vi "Q14070-Z060B B.vi"() -> ()   [LabVIEW 2013]
uses:
  <vilib>/Utility/file.llb/Read From Spreadsheet File (string).vi
  <vilib>/express/express arith-compare/Formula/XNode/ExpressFormulaBlockNode.xnode
  PCI8622_32.dll
  <vilib>/printing/EasyPrintingControls.llb/contents.ctl
  <vilib>/Utility/NIReport.llb/NI_ReportGenerationCore.lvlib
  <vilib>/printing/EasyPrintingControls.llb/report_type.ctl
  <vilib>/Utility/NIReport.llb/NI_report.lvclass
  <vilib>/printing/EasyPrinting.llb/Easy Print VI Panel or Documentation (path).vi
panel:
  out "监控点压力 2":dbl
  out "监控点压力":dbl
  out "右拉压力数组":dbl[](array[numeric])
  out "右位移数组":dbl[](array[numeric])
  out "左拉压力数组":dbl[](array[numeric])
  out "左位移数组":dbl[](array[numeric])
  out "左轴向力数组大小":i32
  in  "电动缸快速":dbl=15.0
  in  "电动缸慢速":dbl=1.0
  out "最大轴向力标准(N)":dbl=200.0 caption="L+Lmax(mm)" format="%#.3f"
  out "循环退出":bool
  in  "?":bool
  in  "密码":string
  in  "?":bool
  in  "?":bool
  in  "截取百分比":dbl=0.05
  in  "半行程":dbl=70.0
  in  "是否取消放行按钮":bool
  out "PLC":bool
  out "齿条传动比":dbl=200.0 caption="L+Lmax(mm)" format="%#.3f"
  out "右平均轴向力(N)":dbl caption="L+Lmax(mm)" format="%#.3f"
  out "左平均轴向力(N)":dbl caption="最大位移偏离Lmax(mm)" format="%#.3f"
  in  "确定按钮":bool
  out "员工ID":string
  in  "出支线工步号":dbl
  out "报警提示":string
  in  "报警工步号":dbl
  out "急停":bool
  out "DeviceHandle":u32
  in  "轴向力设定次数":dbl=5.0
  in  "最小间隙(mm)":dbl=0.0005 format="%#.3f"
  out "本备料状态H":bool
  out "本测试状态H":bool
  out "本自动状态H":bool
  out "夹头松开":bool
  out "测头右位":bool
  out "测头左位":bool
  in  "测头气缸右移":bool
  in  "测头气缸左移":bool
  in  "轴向力已做次数":dbl
  out "轴向力及全行程间隙合格":bool
  out "轴向力启动":bool
  out "间隙启动":bool
  out "夹头夹紧位":bool
  in  "夹头松开":bool
  in  "夹头夹紧":bool
  out "找帽扭矩":dbl=5.0 caption="压力传感器" format="%#.2f"
  out "error out":errorcluster
  out "型号数量":i32
  out "error out 4":errorcluster
  in  "间隙设定调整次数":dbl=5.0
  out "读取产品ID":string
  out "本备料状态":bool
  out "本测试状态":bool
  out "本自动状态":bool
  out "FGCS":string
  out "KSJJ":string
  out "Z060BRFID":string
  out "轴向力Y":dbl[](array[numeric])
  out "轴向力X":dbl[](array[numeric])
  out "间隙X数组":dbl[](array[numeric])
  out "间隙Y数组":dbl[](array[numeric])
  out "error out 3":errorcluster caption="错误输出"
  out "rfid工步号":u32
  out "芯片ID":string="201209190001"
  out "rfid完成":bool
  out "rfid触发":bool
  out "本序已做":bool
  in  "回零完成":bool
  in  "电动缸回零":bool
  in  "单点间隙已调试次数":dbl
  in  "需调整角度(度)":dbl
  in  "转向器中心":dbl
  out "扭矩到达":bool
  out "黄灯":bool
  out "红灯":bool
  out "基准位移":dbl caption="压力传感器" format="%#.4f"
  out "上序不合格":bool
  out "单点间隙合格":bool
  out "上序合格":bool
  out "测头机构电机":u32
  out "复位":bool
  in  "型号选择":u16(ring)=1 items=["J709", "J728", "J706"]
  in  "联线按钮":bool
  in  "工步号":u32
  in  "产品ID":string="201209190001"
  out "间隙位移(mm)":dbl caption="压力传感器" format="%#.3f"
  out "齿条推拉力(N)":dbl format="%#.2f"
  out "齿条扭矩(Nm)":dbl format="%#.2f"
  out "通讯状态":bool
  out "员工姓名":string
  out "工步提示":string
  out "ADODB._Connection Out 2":refnum<k7>
  out "旋转齿条电机":u32
  out "电动缸电机":u32
  in  "停止":bool
  in  "参数加载":bool
  in  "选项卡控件":T1(tab)
  in  "180°外全行程间隙标准(mm)":dbl=0.1 format="%#.3f"
  out "扭动曲线":cluster{"Y":dbl[], "Y":dbl[]}[](graph) caption="压球涨堵头1"
  out "中间位置间隙":dbl caption="间隙值L(mm)" format="%#.3f"
  in  "中间位置最大间隙标准(mm)":dbl=0.07 format="%#.3f"
  out "右180°外全行程间隙":dbl caption="正向最大间隙L1(mm)" format="%#.3f"
  out "左180°外全行程间隙":dbl caption="正向最大间隙L1(mm)" format="%#.3f"
  out "右180°内全行程间隙":dbl caption="正向最大间隙L1(mm)" format="%#.3f"
  out "左180°内全行程间隙":dbl caption="正向最大间隙L1(mm)" format="%#.3f"
  in  "180°内全行程间隙标准(mm)":dbl=0.07 format="%#.3f"
  in  "找帽OK":bool
  out "左全行程间隙":dbl caption="正向最大间隙L1(mm)" format="%#.3f"
  out "右全行程间隙":dbl caption="正向最大间隙L1(mm)" format="%#.3f"
  out "总圈数最大值":dbl
  out "总圈数标准":dbl
  out "总行程最大值":dbl
  out "总行程标准(mm)":dbl
  out "力波动标准(N)":dbl=60.0 caption="L+Lmax(mm)" format="%#.3f"
  out "轴向力标准(N)":dbl=100.0 caption="L+Lmax(mm)" format="%#.3f"
  out "右轴向力波动(N)":dbl caption="L+Lmax(mm)" format="%_4g"
  out "右最大轴向力(N)":dbl caption="L+Lmax(mm)" format="%_4g"
  out "左轴向力波动(N)":dbl caption="最大位移偏离Lmax(mm)" format="%_4g"
  out "左最大轴向力(N)":dbl caption="最大位移偏离Lmax(mm)" format="%_4g"
  out "行程跳动曲线":cluster{"Y":dbl[], "Y":dbl[]}[](graph) caption="压球涨堵头1"
  out "平均轴向力标准(N) max":dbl=200.0 caption="L+Lmax(mm)" format="%#.3f"
  out "总行程":dbl format="%_4g"
  out "总圈数":dbl format="%_4g"
  in  "不合格品":bool
  in  "扭矩停止值":dbl=16.0
  in  "齿条右极限":dbl=-70.0 caption="压力传感器" format="%#.2f"
  in  "齿条左极限":dbl=-262.0 caption="压力传感器" format="%#.2f"
  in  "齿条移动速度":dbl=5.0 caption="压力传感器" format="%#.2f"
  in  "旋转齿条轴找帽转速":dbl=5.0 caption="压力传感器" format="%#.2f"
  in  "测量点扭矩":dbl=4.0 caption="压力传感器" format="%#.2f"
  in  "旋转齿条轴测量转速":dbl caption="压力传感器" format="%#.2f"
  in  "测头机构轴后退位":dbl=30.0 caption="压力传感器" format="%#.2f"
  in  "测头机构轴待检位":dbl caption="压力传感器" format="%#.2f"
  in  "测头机构轴检测位":dbl caption="压力传感器" format="%#.2f"
  in  "测头机构轴移动速度":dbl caption="压力传感器" format="%#.2f"
  in  "机械间隙值":dbl=3.5
  in  "阻挡":bool
  in  "放行":bool
  in  "夹头松开":bool
  in  "夹头夹紧":bool
  in  "测头气缸右移":bool
  in  "测头气缸左移":bool
  in  "支线下降":bool
  in  "支线顶升":bool
  in  "出支线":bool
  in  "进支线":bool
  in  "主线下降":bool
  in  "主线顶升":bool
  in  "下阻挡器放行":bool
  in  "上阻挡器放行":bool
  in  "测头机构轴使能":bool
  in  "测头机构轴后退":bool
  in  "测头机构轴前进":bool
  in  "电动缸速度(mm/s)":dbl=10.0 format="%#.3f"
  out "电动缸位置(mm)":dbl=10000.0 format="%#.3f"
  in  "旋转齿条轴速度(°/s)":dbl=10.0 format="%#.3f"
  out "旋转齿条轴位置(°)":dbl=10000.0 format="%#.3f"
  in  "测头机构轴速度(mm/s)":dbl=10.0 format="%#.3f"
  out "测头机构轴位置(mm)":dbl=10000.0 format="%#.3f"
  in  "旋转齿条轴右转":bool
  in  "旋转齿条轴左转":bool
  in  "旋转齿条轴使能":bool
  in  "电动缸后退":bool
  in  "电动缸使能":bool
  in  "电动缸前进":bool
  in  "齿条扭矩比例偏移":dbl=1.0 format="%#.2f"
  in  "齿条扭矩零点偏移":dbl format="%#.2f"
  in  "齿条推拉力比例偏移":dbl=1.0 format="%#.2f"
  in  "齿条推拉力零点偏移":dbl format="%#.2f"
  in  "间隙位移比例偏移":dbl=1.0 format="%#.2f"
  in  "间隙位移零点偏移":dbl format="%#.2f"
  in  "传感器参数保存":bool
  in  "参数修改":bool
  in  "参数查询":bool
  in  "参数浏览表":string[][](table)
  # "芜湖机械转向器装配线"
  # "间隙及轴向力检测"
  # "湖北唯思凌科装备制造有限公司 设计开发 (C)2015"
  # "Q14070机械转向器装配线"
  # "≤"
  # "间隙测量结果"
  # "间隙测量判定值"
  # "≤"
  # "≤"
  # "≤"
  # "轴向力测量结果"
  # "轴向力测量标准"
  # "≥"
  # "≤"
  # "≥"
  # "≤"
  # "≤"
  # "≥"
  # "不得大于20NM"
  # "传感器校验区"
  # "关于传感器校验：\n1、传感器校验需要由具备资质的单位或部门进行校验。\n2、具备权限的用户才能够修改传感器校验参数和试验参数。\n3、修改校验参数方法：先将比例偏移置为1，修改零点偏移，使零点值与校验的传感器一致；然后根据增幅调整比例偏移。"
  # "注意：\n具备权限的用户才能够修改传感器校验参数和试验参数！"
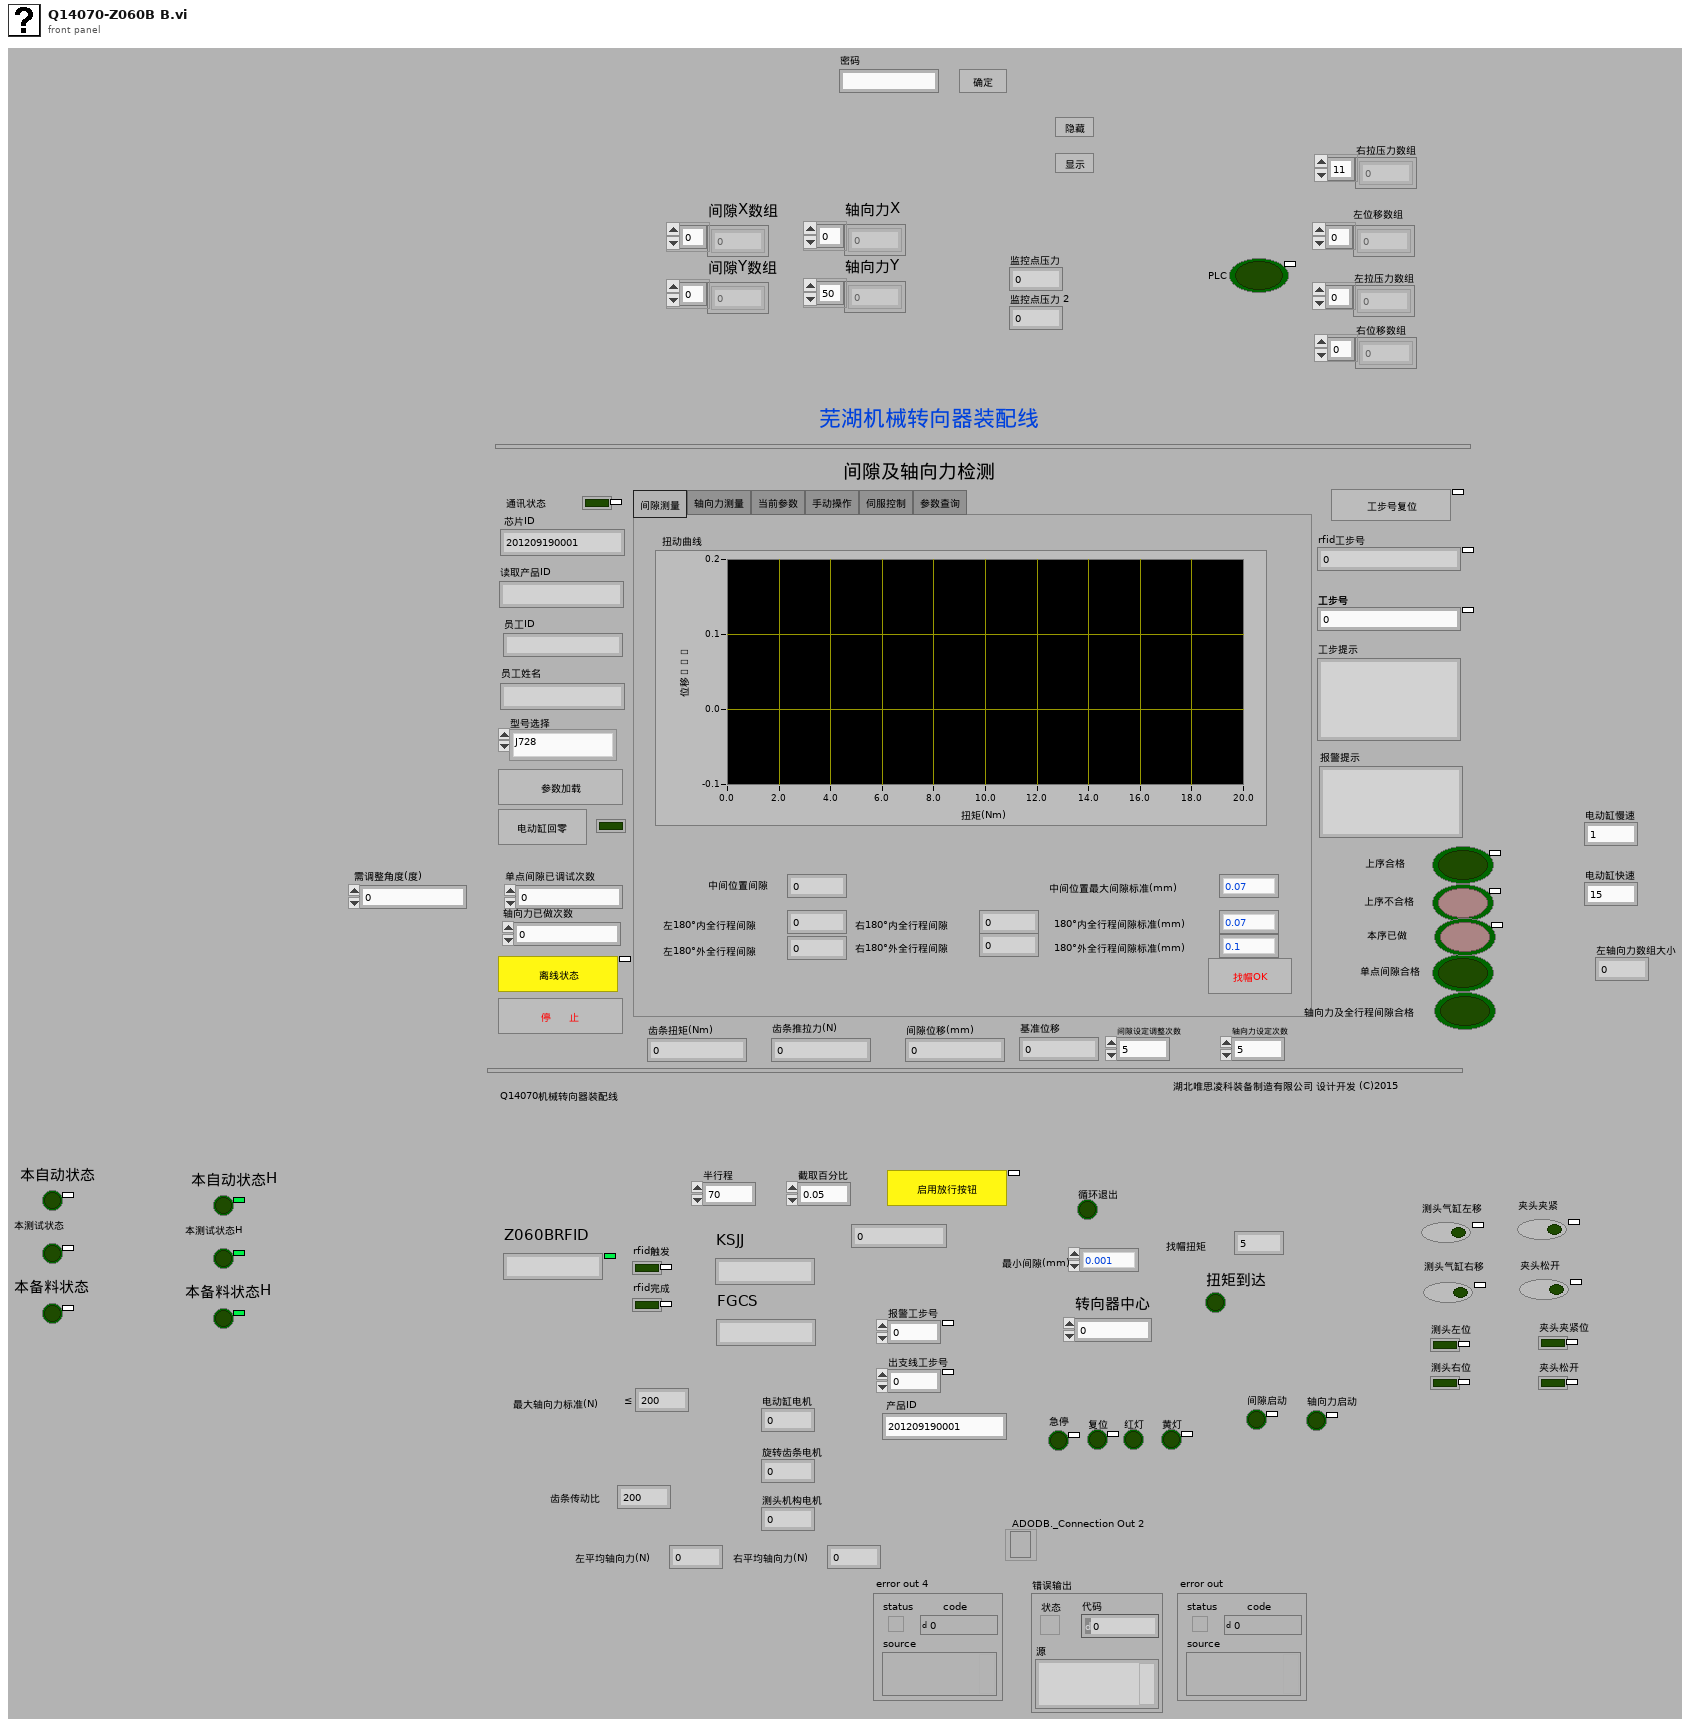
[diagram p1: front panel]
types:
  T1 = enum32{"间隙测量", "轴向力测量", "当前参数", "手动操作", "伺服控制", "传感器校验", "参数查询"}
  T2 = enum8{"Enabled", "Disabled", "Disabled and Grayed Out"}
  T3 = typedef "NI_ReportGenerationCore.lvlib/report_type.ctl" = u16
  T4 = typedef "NI_ReportGenerationCore.lvlib/contents.ctl" = u16
  T5 = typedef "imagedata.ctl" = cluster{"image type":i32, "image depth":i32, "image":u8[], "mask":u8[], "colors":u32[], "Rectangle":cluster{"left":i16, "top":i16, "right":i16, "bottom":i16}}
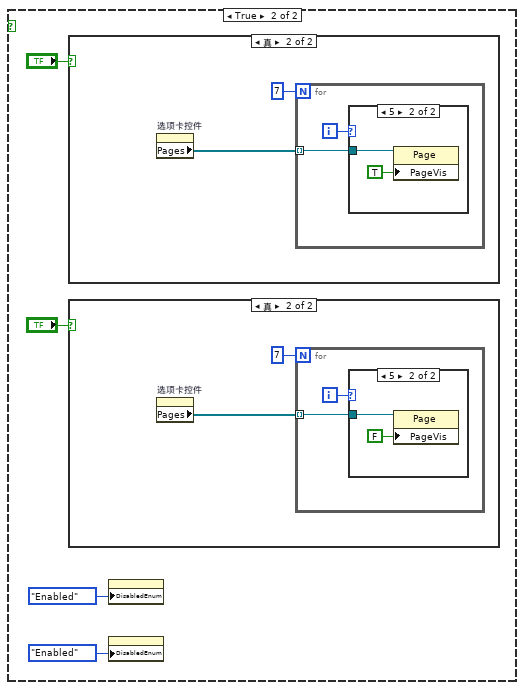
[diagram p2: hidden frame]
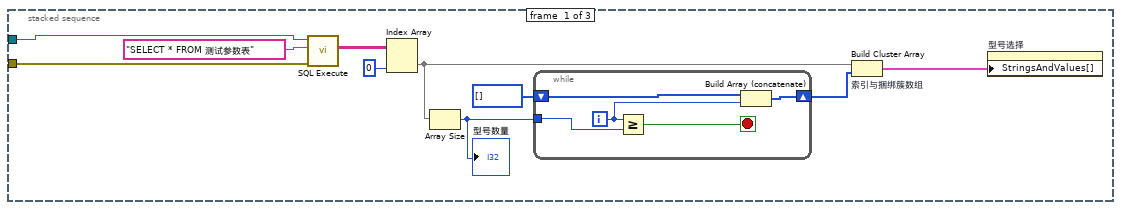
[diagram p9: hidden frame]
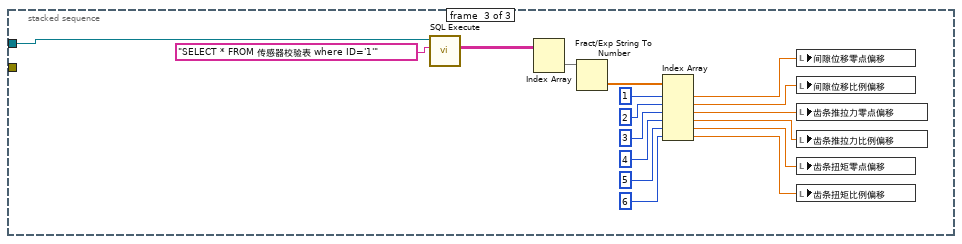
[diagram p10: hidden frame]
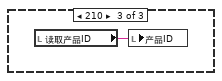
[diagram p12: hidden frame]
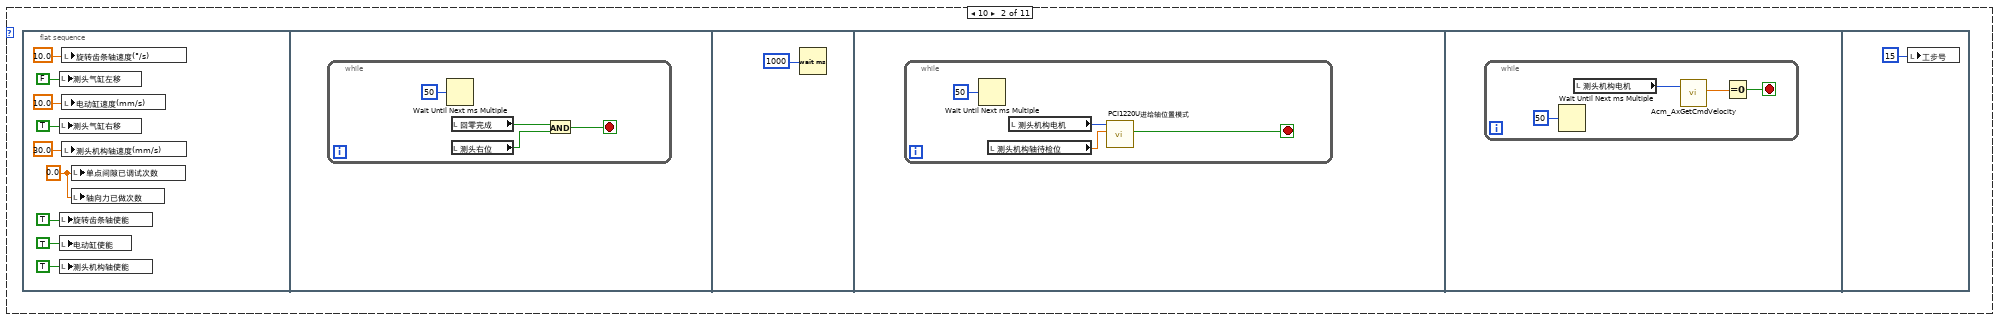
[diagram p14: hidden frame]
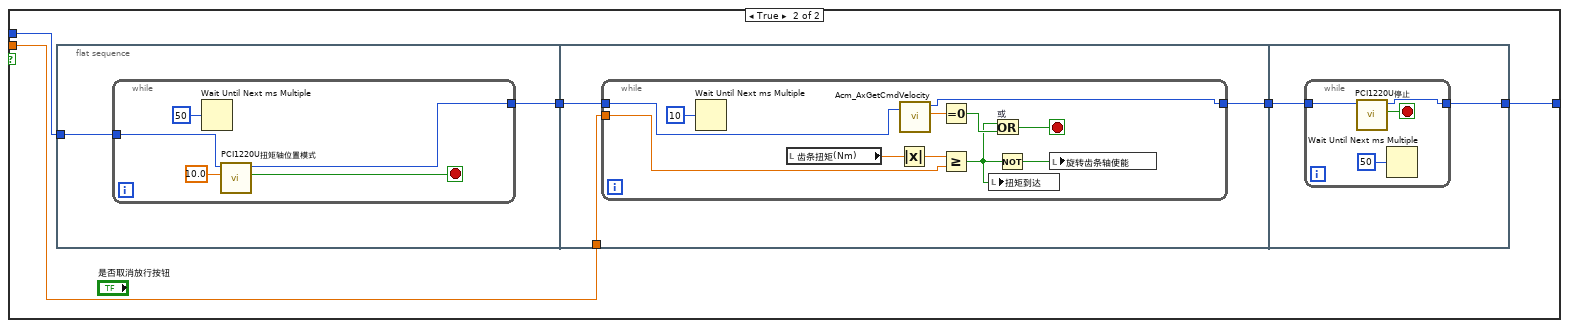
[diagram p15: hidden frame]
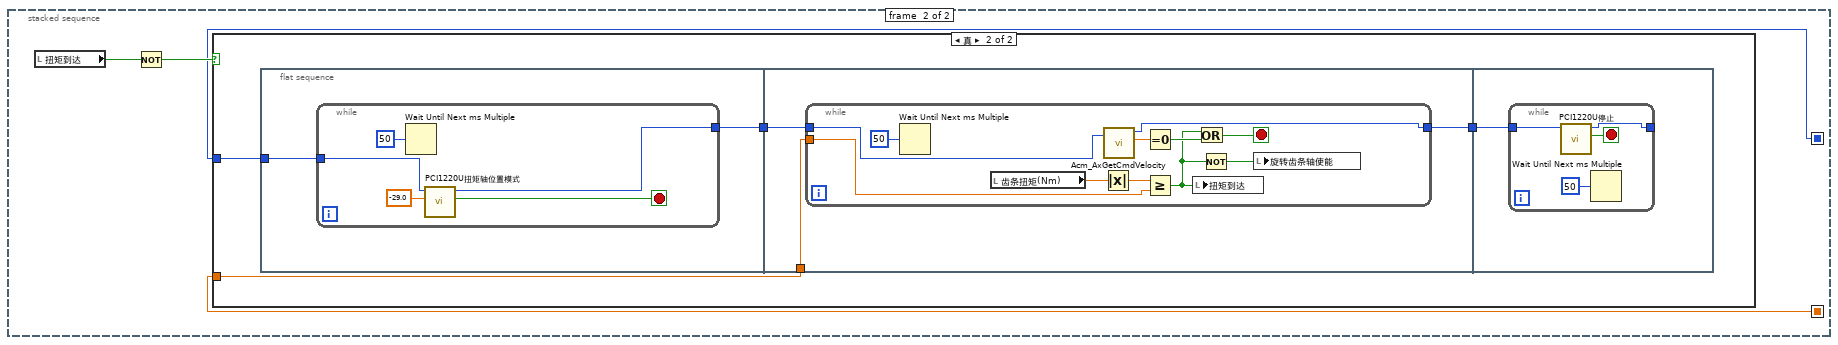
[diagram p16: hidden frame]
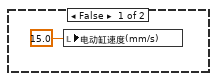
[diagram p17: hidden frame]
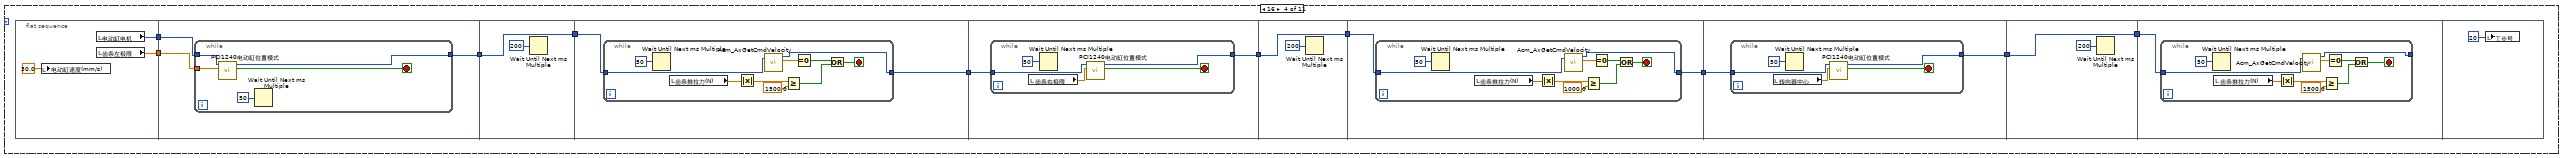
[diagram p19: hidden frame]
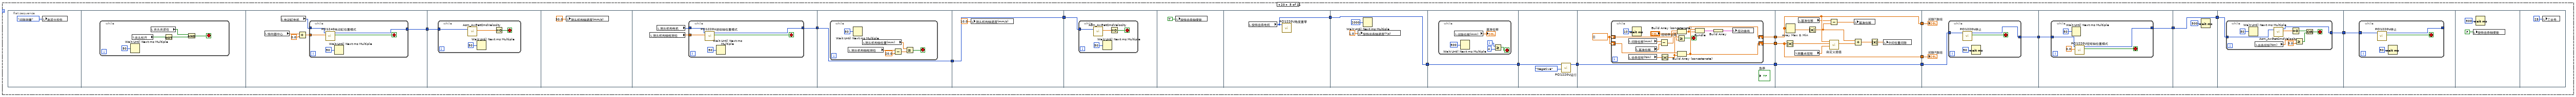
[diagram p20: hidden frame]
diagram:
  n1 = while {
    stop <- FALSE stop-if-true
    n2 = Equal?(x="密码", y="jizhuan") -> (x = y?=w8:bool)
    n3 = Compound Arithmetic op=AND(w8, "?") -> (w6:bool)
    n4 = case shown="假" w6 {
      frame False {
        n5 = property class="Bool (严格)"("DisabledEnum"=T2."Disabled and Grayed Out" ("禁用")) -> ()  [unwired: 2 in, 2 out]
        n6 = property class="Bool (严格)"("DisabledEnum"=T2."Disabled and Grayed Out" ("禁用")) -> ()  [unwired: 2 in, 2 out]
      }
      frame True {
        n7 = case shown="真" "?" {
          frame False {
          }
          frame True {
            n8 = property on="选项卡控件" class="TabCtl (严格)"() -> ("Pages"=w23:refnum<vi>[])  [unwired: 2 in, 2 out]
            n9 = for {
              N: 7 -> [_]
              tunnel: w23 -> [w25] mode=indexing
              i -> [w26]
              n10 = case shown="5" w26 {
                tunnel: w25 -> [_ w28]
                frame 0, Default {
                }
                frame 5 {
                  n11 = property class="Page"(reference=w28, "PageVis"=TRUE ("选项卡可见")) -> ()  [unwired: 1 in, 2 out]
                }
              }
            }
          }
        }
        n12 = case shown="真" "?" {
          frame False {
          }
          frame True {
            n13 = property on="选项卡控件" class="TabCtl (严格)"() -> ("Pages"=w17:refnum<vi>[])  [unwired: 2 in, 2 out]
            n14 = for {
              N: 7 -> [_]
              tunnel: w17 -> [w19] mode=indexing
              i -> [w20]
              n15 = case shown="5" w20 {
                tunnel: w19 -> [_ w22]
                frame 0, Default {
                }
                frame 5 {
                  n16 = property class="Page"(reference=w22, "PageVis"=FALSE ("选项卡可见")) -> ()  [unwired: 1 in, 2 out]
                }
              }
            }
          }
        }
        n17 = property class="Bool (严格)"("DisabledEnum"=T2."Enabled" ("禁用")) -> ()  [unwired: 2 in, 2 out]
        n18 = property class="Bool (严格)"("DisabledEnum"=T2."Enabled" ("禁用")) -> ()  [unwired: 2 in, 2 out]
      }
    }
  }
  n19 = flat-sequence {
    tunnel: [w32] -> w2
    tunnel: [w30] -> w1
    tunnel: w2 -> [w42]
    tunnel: w1 -> [w41]
    frame #0 {
      n20 = First Call?() -> (First Call?: T/F=w29:bool)
      n21 = case shown="真" w29 {
        frame False {
        }
        frame True {
          n22 = while {
            i -> [w37]
            stop <- w35 stop-if-true
            w40 = TRUE ("电动缸使能")
            n23 = local write "回零完成"(FALSE ("回零完成")) -> ()
            n24 = Wait Until Next ms Multiple(millisecond multiple=u32 50 ("毫秒倍数")) -> ()  [unwired: 1 out]
            n25 = local write "电动缸使能"(w40) -> ()
            n26 = local write "测头机构轴使能"(w40) -> ()
            n27 = local write "旋转齿条轴使能"(w40) -> ()
            n28 = Greater Or Equal?(x=w37, y=30) -> (x >= y?=w35:bool)
          }
        }
      }
      n29 = call "ADO Connection Create.vi"() -> ("error out"=w33:errorcluster, "ADODB._Connection Out"=w34:refnum<k7>)  [unwired: 10 in]
      n30 = call "ADO Connection Open.vi"("error in (no error)"=w33, "ConnectionString"="Provider=Microsoft.Jet.OLEDB.4.0;Data Source=D:\\Q14070-Z060人机界面\\参数\\参数Z060.mdb;Persist Security Info=False;Jet OLEDB:Database Password=1234;", "ADODB._Connection In"=w34) -> ("error out"=w30:errorcluster, "ADODB._Connection Out"=w32:refnum<k7>)  [unwired: 7 in]
    }
    frame #1 {
      n31 = while {
        tunnel: w42 -> [w44]
        tunnel: w41 -> [w43]
        stop <- w48 stop-if-true
        n32 = Wait (ms)(milliseconds to wait=u32 50 ("等待时间（毫秒）")) -> ()  [unwired: 1 out]
        n33 = First Call?() -> (First Call?: T/F=w47:bool)
        n34 = Or(x=w47, y="参数加载") -> (x .or. y?=w46:bool)
        n35 = case shown="真" w46 {
          tunnel: w44 -> [_ w51]
          tunnel: w43 -> [_ w50]
          frame False {
          }
          frame True {
            n36 = stacked-sequence {
              tunnel: w51 -> [w57 w68 w126]
              tunnel: w50 -> [w52 _ _]
              frame #0 {
                n37 = call "SQL Execute.vi"("error in (no error)"=w52, "Command Text"="SELECT * FROM 测试参数表", "ADODB._Connection In"=w57) -> ("Data"=w55:string[][])  [unwired: 5 in, 3 out]
                n38 = Index Array(array=w55, index (col)=0 ("索引 (行)")) -> (element=w59:string[])  [unwired: 1 in]
                n39 = Array Size(array=w59) -> (size(s)=w54:i32)
                "型号数量" <- w54
                n40 = while {
                  shift-right: [w66] -> w58
                  shift-left: i32[] [] -> [w65]
                  tunnel: w54 -> [w63]
                  i -> [w64]
                  stop <- w62 stop-if-true
                  n41 = Greater Or Equal?(x=w64, y=w63) -> (x >= y?=w62:bool)
                  n42 = Build Array (concatenate)(w65, w64) -> (w66:i32[])
                }
                n43 = Build Cluster Array "索引与捆绑簇数组"(w59, w58) -> (w53:cluster{"String":string, i32}[])
                n44 = property on="型号选择" class="Ring (严格)"("StringsAndValues[]"=w53) -> ()  [unwired: 2 in, 2 out]
              }
              frame #1 {
                n45 = property on="型号选择" class="Ring (严格)"() -> ("RingText.Text"=w69:string)  [unwired: 2 in, 2 out]
                n46 = call "创建文本2"("型号选择"=w69) -> ("Result"=w73:string)  [unwired: 13 in, 1 out]
                n47 = call "SQL Execute.vi"("Command Text"=w73, "ADODB._Connection In"=w68) -> ("Data"=w72:string[][])  [unwired: 6 in, 3 out]
                n48 = Index Array(array=w72, index (row)=0 ("索引 (行)")) -> (element=w70:string[])  [unwired: 1 in]
                n49 = Fract/Exp String To Number ("分数/指数字符串至数值转换")(string=w70) -> (number=w67:dbl[])  [unwired: 3 in, 1 out]
                n50 = stacked-sequence {
                  tunnel: w67 -> [w102]
                  frame #0 {
                    n51 = Index Array ("索引数组")(array=w102, index #1=2 ("索引"), index #2=3 ("索引"), index #3=4 ("索引"), index #4=5 ("索引"), index #5=6 ("索引"), index #6=7 ("索引"), index #7=8 ("索引"), index #8=9 ("索引"), index #9=10 ("索引"), index #10=11 ("索引"), index #11=12 ("索引"), index #12=13 ("索引"), index #13=14 ("索引"), index #14=15 ("索引"), index #15=16 ("索引"), index #16=17 ("索引"), index #17=18 ("索引"), index #18=19 ("索引"), index #19=20 ("索引")) -> (element #1=w101:dbl, element #2=w100:dbl, element #3=w99:dbl, element #4=w98:dbl, element #5=w97:dbl, element #6=w96:dbl, element #7=w95:dbl, element #8=w94:dbl, element #9=w93:dbl, element #10=w92:dbl, element #11=w85:dbl, element #12=w84:dbl, element #13=→"齿条传动比":dbl, element #14=→"力波动标准(N)":dbl, element #15=→"轴向力标准(N)":dbl, element #16=→"平均轴向力标准(N) max":dbl, element #17=→"总圈数标准":dbl, element #18=→"总圈数最大值":dbl, element #19=w80:dbl)
                    n52 = local write "测头机构轴移动速度"(w101) -> ()
                    n53 = local write "测头机构轴检测位"(w100) -> ()
                    n54 = local write "测头机构轴待检位"(w99) -> ()
                    n55 = local write "测头机构轴后退位"(w98) -> ()
                    n56 = local write "齿条移动速度"(w97) -> ()
                    n57 = local write "齿条左极限"(w96) -> ()
                    n58 = local write "齿条右极限"(w95) -> ()
                    n59 = local write "旋转齿条轴找帽转速"(w94) -> ()
                    n60 = local write "旋转齿条轴测量转速"(w93) -> ()
                    n61 = local write "测量点扭矩"(w92) -> ()
                    n62 = local write "总行程标准(mm)"(w85) -> ()
                    n63 = local write "总行程最大值"(w84) -> ()
                    n64 = local write "转向器中心"(w80) -> ()
                  }
                }
              }
              frame #2 {
                n65 = call "SQL Execute.vi"("Command Text"="SELECT * FROM 传感器校验表 where ID='1'", "ADODB._Connection In"=w126) -> ("Data"=w128:string[][])  [unwired: 6 in, 3 out]
                n66 = Index Array(array=w128) -> (element=w129:string[])  [unwired: 2 in]
                n67 = Fract/Exp String To Number ("分数/指数字符串至数值转换")(string=w129) -> (number=w119:dbl[])  [unwired: 3 in, 1 out]
                n68 = Index Array(array=w119, index #1=1 ("索引"), index #2=2 ("索引"), index #3=3 ("索引"), index #4=4 ("索引"), index #5=5 ("索引"), index #6=6 ("索引")) -> (element #1=w118:dbl, element #2=w117:dbl, element #3=w116:dbl, element #4=w115:dbl, element #5=w114:dbl, element #6=w113:dbl)
                n69 = local write "间隙位移零点偏移"(w118) -> ()
                n70 = local write "间隙位移比例偏移"(w117) -> ()
                n71 = local write "齿条推拉力零点偏移"(w116) -> ()
                n72 = local write "齿条推拉力比例偏移"(w115) -> ()
                n73 = local write "齿条扭矩零点偏移"(w114) -> ()
                n74 = local write "齿条扭矩比例偏移"(w113) -> ()
              }
            }
          }
        }
        n75 = local read "停止"() -> (w48:bool)
        "ADODB._Connection Out 2" <- w44
      }
    }
  }
  n76 = while {
    stop <- w131 stop-if-true
    n77 = stacked-sequence {
      frame #0 {
        n78 = flat-sequence {
          frame #0 {
          }
          frame #1 {
            "PLC" <- "阻挡"
          }
          frame #2 {
            n79 = First Call?() -> (First Call?: T/F=w133:bool)
            n80 = case shown="真" w133 {
              frame False {
              }
              frame True {
                n81 = call "员工管理测试程序.vi"() -> ("员工姓名"=w135:string, "员工ID"=w134:string)  [unwired: 10 in]
                n82 = local write "员工ID"(w134) -> ()
                n83 = local write "员工姓名"(w135) -> ()
              }
            }
          }
          frame #3 {
          }
          frame #4 {
          }
          frame #5 {
          }
          frame #6 {
          }
        }
      }
      frame #1 {
        n84 = flat-sequence {
          frame #0 {
            n85 = property on="型号选择" class="Ring (严格)"() -> ("RingText.Text"=w139:string)  [unwired: 2 in, 2 out]
            n86 = case shown="\"J728\"" w139 {
              frame "J709", Default {
                w140 = FALSE ("可见")
                w141 = TRUE ("可见")
                n87 = property on="左全行程间隙" class="DigNum (严格)"("Visible"=w141) -> ()  [unwired: 2 in, 2 out]
                n88 = property on="右全行程间隙" class="DigNum (严格)"("Visible"=w141) -> ()  [unwired: 2 in, 2 out]
                n89 = property on="左180°内全行程间隙" class="DigNum (严格)"("Visible"=w140) -> ()  [unwired: 2 in, 2 out]
                n90 = property on="左180°外全行程间隙" class="DigNum (严格)"("Visible"=w140) -> ()  [unwired: 2 in, 2 out]
                n91 = property on="右180°内全行程间隙" class="DigNum (严格)"("Visible"=w140) -> ()  [unwired: 2 in, 2 out]
                n92 = property on="右180°外全行程间隙" class="DigNum (严格)"("Visible"=w140) -> ()  [unwired: 2 in, 2 out]
              }
              frame "J706" {
                w142 = TRUE ("可见")
                w143 = FALSE ("可见")
                n93 = property on="左全行程间隙" class="DigNum (严格)"("Visible"=w143) -> ()  [unwired: 2 in, 2 out]
                n94 = property on="右全行程间隙" class="DigNum (严格)"("Visible"=w143) -> ()  [unwired: 2 in, 2 out]
                n95 = property on="左180°内全行程间隙" class="DigNum (严格)"("Visible"=w142) -> ()  [unwired: 2 in, 2 out]
                n96 = property on="左180°外全行程间隙" class="DigNum (严格)"("Visible"=w142) -> ()  [unwired: 2 in, 2 out]
                n97 = property on="右180°内全行程间隙" class="DigNum (严格)"("Visible"=w142) -> ()  [unwired: 2 in, 2 out]
                n98 = property on="右180°外全行程间隙" class="DigNum (严格)"("Visible"=w142) -> ()  [unwired: 2 in, 2 out]
              }
              frame "J728" {
                w144 = TRUE ("可见")
                w145 = FALSE ("可见")
                n99 = property on="左全行程间隙" class="DigNum (严格)"("Visible"=w145) -> ()  [unwired: 2 in, 2 out]
                n100 = property on="右全行程间隙" class="DigNum (严格)"("Visible"=w145) -> ()  [unwired: 2 in, 2 out]
                n101 = property on="左180°内全行程间隙" class="DigNum (严格)"("Visible"=w144) -> ()  [unwired: 2 in, 2 out]
                n102 = property on="左180°外全行程间隙" class="DigNum (严格)"("Visible"=w144) -> ()  [unwired: 2 in, 2 out]
                n103 = property on="右180°内全行程间隙" class="DigNum (严格)"("Visible"=w144) -> ()  [unwired: 2 in, 2 out]
                n104 = property on="右180°外全行程间隙" class="DigNum (严格)"("Visible"=w144) -> ()  [unwired: 2 in, 2 out]
              }
            }
          }
          frame #1 {
            (unwired) string[] ["I急停按钮", "I自动旋钮", "I启动按钮", "I备用按钮", "I复位按钮", "I上阻挡器放行", "I下阻挡器放行", "I进支线按钮"] ("I0说明")
            (unwired) string[] ["I出支线按钮", "I主线顶升按钮", "I主线下降按钮", "I支线顶升按钮", "I支线下降按钮", "I气压报警", "未使用", "未使用"] ("I0说明")
            n105 = local read "间隙位移(mm)"() -> (w148:dbl)
            n106 = Greater Or Equal?(x=w148, y=4.0) -> (x >= y?=w146:bool)
            n107 = case shown="真" w146 {
              frame False {
              }
              frame True {
                n108 = local write "测头机构轴使能"(FALSE ("测头机构轴使能")) -> ()
              }
            }
          }
          frame #2 {
            (unwired) string[] ["I电动缸SRDY", "I电动缸ZSPD", "I电动缸ALRM", "I间隙进给SRDY", "I间隙进给ZSPD", "I间隙进给ALRM", "I间隙旋转SRPD", "I间隙旋转ZSPD"] ("I0说明")
            n109 = local read "测头机构轴位置(mm)"() -> (w152:dbl)
            n110 = Greater Or Equal?(x=w152, y=90.0) -> (x >= y?=w150:bool)
            n111 = case shown="假" w150 {
              frame False {
                w153 = T2."Enabled" ("禁用")
                n112 = property on="测头气缸左移" class="Bool (严格)"("DisabledEnum"=w153) -> ()  [unwired: 2 in, 2 out]
                n113 = property on="测头气缸右移" class="Bool (严格)"("DisabledEnum"=w153) -> ()  [unwired: 2 in, 2 out]
                n114 = property on="测头气缸左移" class="Bool"("DisabledEnum"=w153) -> ()  [unwired: 2 in, 2 out]
                n115 = property on="测头气缸右移" class="Bool"("DisabledEnum"=w153) -> ()  [unwired: 2 in, 2 out]
              }
              frame True {
                w154 = T2."Disabled" ("禁用")
                w155 = FALSE ("测头气缸右移")
                n116 = local write "测头气缸右移"(w155) -> ()
                n117 = local write "测头气缸左移"(w155) -> ()
                n118 = property on="测头气缸左移" class="Bool (严格)"("DisabledEnum"=w154) -> ()  [unwired: 2 in, 2 out]
                n119 = property on="测头气缸右移" class="Bool (严格)"("DisabledEnum"=w154) -> ()  [unwired: 2 in, 2 out]
                n120 = property on="测头气缸左移" class="Bool"("DisabledEnum"=w154) -> ()  [unwired: 2 in, 2 out]
                n121 = property on="测头气缸右移" class="Bool"("DisabledEnum"=w154) -> ()  [unwired: 2 in, 2 out]
              }
            }
          }
          frame #3 {
            (unwired) string[] ["I间隙旋转ALRM", "I扭矩旋转SRPD", "I扭矩旋转ZSPD", "I扭矩旋转ALRM", "I拧紧机合格", "I拧紧机不合格", "I拧紧机报警", "未使用"] ("I0说明")
          }
        }
        n122 = local read "急停"() -> (w138:bool)
        n123 = local read "复位"() -> (w137:bool)
        n124 = Compound Arithmetic op=OR(invert w138, w137) -> (→"循环退出":bool)
      }
      frame #2 {
        n125 = flat-sequence {
          frame #0 {
            (unwired) string[] ["I自制气缸进位", "I自制气缸原位", "I上工位检测", "I本工位检测", "I下工位检测", "I主线顶升上位", "I主线顶升下位", "I支线顶升上位"] ("I0说明")
          }
          frame #1 {
            (unwired) string[] ["I支线顶升下位", "I支线进到位", "I支线退到位", "I位移气缸原位", "I位移气缸进位", "I拧紧机在位", "I电动缸原位", "I电动缸进位"] ("I0说明")
          }
          frame #2 {
            (unwired) string[] ["未使用", "未使用", "未使用", "未使用", "未使用", "未使用", "未使用", "未使用"] ("I0说明")
          }
          frame #3 {
            (unwired) string[] ["未使用", "未使用", "未使用", "未使用", "未使用", "未使用", "未使用", "未使用"] ("I0说明")
          }
        }
        n126 = local read "本备料状态"() -> (w156:bool)
        n127 = local read "本自动状态"() -> (w158:bool)
        n128 = local read "本测试状态"() -> (w157:bool)
        n129 = local write "本备料状态H"(w156) -> ()
        n130 = local write "本自动状态H"(w158) -> ()
        n131 = local write "本测试状态H"(w157) -> ()
      }
      frame #3 {
        n132 = local read "报警工步号"() -> (w160:dbl)
        n133 = local read "工步号"() -> (w162:u32)
        n134 = case shown="3" w160 {
          tunnel: [_ "操作步骤错请取胶瓶" "操作步骤错误请点标" "测头气缸不在原位" "急停被按下" "气压报警" "电动缸伺服报警" "旋转伺服服报警" "测头伺服服报警"] -> w159
          frame 0, Default {
          }
          frame 1 {
          }
          frame 3 {
          }
          frame 2 {
          }
          frame 4 {
          }
          frame 5 {
          }
          frame 6 {
          }
          frame 7 {
          }
          frame 8 {
          }
        }
        "报警提示" <- w159
        n135 = case shown="0, 默认" w162 {
          tunnel: [w172 "请取胶瓶" ("工步描述") "请对锁紧螺母加力" ("工步描述") "灵敏度测试中" ("工步描述") "有油刚度测试中" ("工步描述") "安装好锁紧螺母后，按顶升按钮，夹具夹紧" ("工步描述") "请点击启动按钮进行试验" ("工步描述") "探头气缸右移" ("工步描述") "电动缸前进找中" ("工步描述") "探头前进测试开始" ("工步描述") "探头退回" ("工步描述") "轴向力测试中" ("工步描述") "测头后退夹抓松开" ("工步描述") "伺服回零" ("工步描述") "力特性试验完成" ("工步描述") "套好输出轴把手，按启动按钮，做回正力试验" ("工步描述") "回正力试验中" ("工步描述") "试验完成，将把手拉回，取下油管，按顶升按钮" ("工步描述") "拆下锁紧螺母和输入轴万向节，按顶升按钮" ("工步描述")] -> w161
          frame 0, Default {
            n136 = local read "联线按钮"() -> (w171:bool)
            n137 = case shown="真" w171 {
              tunnel: ["等待工件" ("工步描述") "等待扫描条码" ("工步描述")] -> w172
              frame False {
              }
              frame True {
              }
            }
          }
          frame 1 {
          }
          frame 2 {
          }
          frame 3 {
          }
          frame 4 {
          }
          frame 5 {
          }
          frame 6 {
          }
          frame 10 {
          }
          frame 15 {
          }
          frame 20 {
          }
          frame 30 {
          }
          frame 40 {
          }
          frame 45 {
          }
          frame 50 {
          }
          frame 55 {
          }
          frame 60 {
          }
          frame 70 {
          }
          frame 80 {
          }
          frame 56 {
          }
        }
        "工步提示" <- w161
      }
      frame #4 {
        n138 = local read "急停"() -> (w193:bool)
        n139 = local read "红灯"() -> (w195:bool)
        n140 = local read "复位"() -> (w196:bool)
        n141 = local read "复位"() -> (w198:bool)
        n142 = local read "停止"() -> (w200:bool)
        n143 = local read "红灯"() -> (w197:bool)
        n144 = case shown="假" w193 {
          frame False {
            n145 = local write "红灯"(TRUE ("红灯")) -> ()
          }
          frame True {
            n146 = local write "红灯"(FALSE ("复位")) -> ()
          }
        }
        n147 = Or(x=w195, y=w196) -> (x .or. y?=w194:bool)
        n148 = Compound Arithmetic op=OR(w198, w200, w197) -> (w199:bool)
        n149 = case shown="真" w194 {
          frame False {
          }
          frame True {
            n150 = local write "回零完成"(FALSE ("夹头夹紧控制")) -> ()
          }
        }
        n151 = case shown="真" w199 {
          frame False {
          }
          frame True {
            n152 = local read "电动缸电机"() -> (w206:u32)
            n153 = local read "旋转齿条电机"() -> (w205:u32)
            n154 = local read "测头机构电机"() -> (w204:u32)
            n155 = call "PCI1220U停止.vi"("AxisHandle IN"=w206) -> ()  [unwired: 9 in, 2 out]
            n156 = call "PCI1220U停止.vi"("AxisHandle IN"=w205) -> ()  [unwired: 9 in, 2 out]
            n157 = call "PCI1220U停止.vi"("AxisHandle IN"=w204) -> ()  [unwired: 9 in, 2 out]
          }
        }
      }
      frame #5 {
        n158 = local read "齿条扭矩(Nm)"() -> (w209:dbl)
        n159 = local read "旋转齿条轴左转"() -> (w215:bool)
        n160 = local read "旋转齿条轴右转"() -> (w210:bool)
        n161 = Absolute Value(x=w209) -> (abs(x)=w214:dbl)
        n162 = Not(x=w215) -> (.not. x?=w211:bool)
        n163 = Less?(x=w214, y=20.0) -> (x < y?=w212:bool)
        n164 = local read "黄灯"() -> (w207:bool)
        n165 = Compound Arithmetic op=AND(w210, w211, w212, w207) -> (w208:bool)
        n166 = case shown="真" w208 {
          frame False {
          }
          frame True {
            n167 = flat-sequence {
              tunnel: [w219] -> w217
              tunnel: w217 -> [w221]
              tunnel: [w221] -> w216
              tunnel: w216 -> [w232]
              frame #0 {
                n168 = local read "旋转齿条电机"() -> (w218:u32)
                n169 = call "PCI1220U运行.vi"("方向"=enum32{"Negative", "Positive"}."Negative" ("Direction"), "AxisHandle IN"=w218) -> ("AxisHandle OUT"=w219:u32)  [unwired: 9 in]
              }
              frame #1 {
                n170 = while {
                  stop <- w225 stop-if-true
                  n171 = Wait (ms)(milliseconds to wait=u32 50 ("毫秒倍数")) -> ()  [unwired: 1 out]
                  n172 = local read "齿条扭矩(Nm)"() -> (w230:dbl)
                  n173 = local read "旋转齿条轴右转"() -> (w227:bool)
                  n174 = Absolute Value(x=w230) -> (abs(x)=w229:dbl)
                  n175 = Not(x=w227) -> (.not. x?=w224:bool)
                  n176 = Greater?(x=w229, y=10.0) -> (0:w226:bool)
                  n177 = local read "复位"() -> (w223:bool)
                  n178 = local read "红灯"() -> (w222:bool)
                  n179 = Compound Arithmetic op=OR(w226, w224, w223, w222) -> (w225:bool)
                }
              }
              frame #2 {
                n180 = call "PCI1220U停止.vi"("AxisHandle IN"=w232) -> ()  [unwired: 9 in, 2 out]
              }
            }
          }
        }
      }
      frame #6 {
        n181 = local read "齿条扭矩(Nm)"() -> (w237:dbl)
        n182 = local read "旋转齿条轴右转"() -> (w241:bool)
        n183 = local read "旋转齿条轴左转"() -> (w239:bool)
        n184 = Absolute Value(x=w237) -> (abs(x)=w236:dbl)
        n185 = Not(x=w241) -> (.not. x?=w238:bool)
        n186 = Less?(x=w236, y=20.0) -> (x < y?=w234:bool)
        n187 = local read "黄灯"() -> (w233:bool)
        n188 = Compound Arithmetic op=AND(w239, w238, w234, w233) -> (w240:bool)
        n189 = case shown="真" w240 {
          frame False {
          }
          frame True {
            n190 = flat-sequence {
              tunnel: [w245] -> w243
              tunnel: w243 -> [w247]
              tunnel: [w247] -> w242
              tunnel: w242 -> [w258]
              frame #0 {
                n191 = local read "旋转齿条电机"() -> (w244:u32)
                n192 = call "PCI1220U运行.vi"("方向"=enum32{"Negative", "Positive"}."Positive" ("Direction"), "AxisHandle IN"=w244) -> ("AxisHandle OUT"=w245:u32)  [unwired: 9 in]
              }
              frame #1 {
                n193 = while {
                  stop <- w250 stop-if-true
                  n194 = Wait (ms)(milliseconds to wait=u32 50 ("毫秒倍数")) -> ()  [unwired: 1 out]
                  n195 = local read "齿条扭矩(Nm)"() -> (w256:dbl)
                  n196 = local read "旋转齿条轴左转"() -> (w253:bool)
                  n197 = Absolute Value(x=w256) -> (abs(x)=w255:dbl)
                  n198 = Not(x=w253) -> (.not. x?=w251:bool)
                  n199 = Greater?(x=w255, y=10.0) -> (0:w252:bool)
                  n200 = local read "复位"() -> (w249:bool)
                  n201 = local read "红灯"() -> (w248:bool)
                  n202 = Compound Arithmetic op=OR(w249, w248, w252, w251) -> (w250:bool)
                }
              }
              frame #2 {
                n203 = call "PCI1220U停止.vi"("AxisHandle IN"=w258) -> ()  [unwired: 9 in, 2 out]
              }
            }
          }
        }
      }
      frame #7 {
        n204 = local read "齿条推拉力(N)"() -> (w263:dbl)
        n205 = Absolute Value(x=w263) -> (abs(x)=w267:dbl)
        n206 = local read "电动缸后退"() -> (w259:bool)
        n207 = local read "电动缸前进"() -> (w260:bool)
        n208 = Less?(x=w267, y=1000.0) -> (x < y?=w265:bool)
        n209 = Not(x=w259) -> (.not. x?=w264:bool)
        n210 = local read "黄灯"() -> (w261:bool)
        n211 = Compound Arithmetic op=AND(w260, w264, w261, w265) -> (w262:bool)
        n212 = case shown="真" w262 {
          frame False {
          }
          frame True {
            n213 = flat-sequence {
              tunnel: [w271] -> w269
              tunnel: w269 -> [w273]
              tunnel: [w273] -> w268
              tunnel: w268 -> [w284]
              frame #0 {
                n214 = local read "电动缸电机"() -> (w270:u32)
                n215 = call "PCI1220U运行.vi"("方向"=enum32{"Negative", "Positive"}."Positive" ("Direction"), "AxisHandle IN"=w270) -> ("AxisHandle OUT"=w271:u32)  [unwired: 9 in]
              }
              frame #1 {
                n216 = while {
                  stop <- w281 stop-if-true
                  n217 = Wait (ms)(milliseconds to wait=u32 50 ("毫秒倍数")) -> ()  [unwired: 1 out]
                  n218 = local read "齿条推拉力(N)"() -> (w275:dbl)
                  n219 = Absolute Value(x=w275) -> (abs(x)=w277:dbl)
                  n220 = local read "电动缸前进"() -> (w278:bool)
                  n221 = Greater?(x=w277, y=1000.0) -> (0:w274:bool)
                  n222 = Not(x=w278) -> (.not. x?=w282:bool)
                  n223 = local read "复位"() -> (w280:bool)
                  n224 = local read "红灯"() -> (w279:bool)
                  n225 = Compound Arithmetic op=OR(w280, w279, w282, w274) -> (w281:bool)
                }
              }
              frame #2 {
                n226 = call "PCI1220U停止.vi"("AxisHandle IN"=w284) -> ()  [unwired: 9 in, 2 out]
              }
            }
          }
        }
      }
      frame #8 {
        n227 = local read "齿条推拉力(N)"() -> (w289:dbl)
        n228 = Absolute Value(x=w289) -> (abs(x)=w293:dbl)
        n229 = local read "电动缸前进"() -> (w285:bool)
        n230 = local read "电动缸后退"() -> (w286:bool)
        n231 = Less?(x=w293, y=1000.0) -> (x < y?=w291:bool)
        n232 = Not(x=w285) -> (.not. x?=w290:bool)
        n233 = local read "黄灯"() -> (w287:bool)
        n234 = Compound Arithmetic op=AND(w286, w290, w287, w291) -> (w288:bool)
        n235 = case shown="真" w288 {
          frame False {
          }
          frame True {
            n236 = flat-sequence {
              tunnel: [w297] -> w295
              tunnel: w295 -> [w299]
              tunnel: [w299] -> w294
              tunnel: w294 -> [w310]
              frame #0 {
                n237 = local read "电动缸电机"() -> (w296:u32)
                n238 = call "PCI1220U运行.vi"("方向"=enum32{"Negative", "Positive"}."Negative" ("Direction"), "AxisHandle IN"=w296) -> ("AxisHandle OUT"=w297:u32)  [unwired: 9 in]
              }
              frame #1 {
                n239 = while {
                  stop <- w307 stop-if-true
                  n240 = Wait (ms)(milliseconds to wait=u32 50 ("毫秒倍数")) -> ()  [unwired: 1 out]
                  n241 = local read "齿条推拉力(N)"() -> (w303:dbl)
                  n242 = Absolute Value(x=w303) -> (abs(x)=w301:dbl)
                  n243 = local read "电动缸后退"() -> (w304:bool)
                  n244 = Greater?(x=w301, y=1000.0) -> (0:w300:bool)
                  n245 = Not(x=w304) -> (.not. x?=w308:bool)
                  n246 = local read "复位"() -> (w305:bool)
                  n247 = local read "红灯"() -> (w306:bool)
                  n248 = Compound Arithmetic op=OR(w305, w306, w308, w300) -> (w307:bool)
                }
              }
              frame #2 {
                n249 = call "PCI1220U停止.vi"("AxisHandle IN"=w310) -> ()  [unwired: 9 in, 2 out]
              }
            }
          }
        }
      }
      frame #9 {
        n250 = local read "测头机构轴后退"() -> (w311:bool)
        n251 = local read "测头机构轴前进"() -> (w312:bool)
        n252 = Not(x=w311) -> (.not. x?=w315:bool)
        n253 = local read "黄灯"() -> (w313:bool)
        n254 = Compound Arithmetic op=AND(w312, w315, w313) -> (w314:bool)
        n255 = case shown="真" w314 {
          frame False {
          }
          frame True {
            n256 = flat-sequence {
              tunnel: [w319] -> w317
              tunnel: w317 -> [w321]
              tunnel: [w321] -> w316
              tunnel: w316 -> [w328]
              frame #0 {
                n257 = local read "测头机构电机"() -> (w318:u32)
                n258 = call "PCI1220U运行.vi"("方向"=enum32{"Negative", "Positive"}."Positive" ("Direction"), "AxisHandle IN"=w318) -> ("AxisHandle OUT"=w319:u32)  [unwired: 9 in]
              }
              frame #1 {
                n259 = while {
                  stop <- w325 stop-if-true
                  n260 = local read "测头机构轴前进"() -> (w322:bool)
                  n261 = Wait (ms)(milliseconds to wait=u32 50 ("毫秒倍数")) -> ()  [unwired: 1 out]
                  n262 = Not(x=w322) -> (.not. x?=w326:bool)
                  n263 = local read "复位"() -> (w324:bool)
                  n264 = local read "红灯"() -> (w323:bool)
                  n265 = Compound Arithmetic op=OR(w324, w323, w326) -> (w325:bool)
                }
              }
              frame #2 {
                n266 = call "PCI1220U停止.vi"("AxisHandle IN"=w328) -> ()  [unwired: 9 in, 2 out]
              }
            }
          }
        }
      }
      frame #10 {
        n267 = local read "测头机构轴前进"() -> (w329:bool)
        n268 = local read "测头机构轴后退"() -> (w330:bool)
        n269 = Not(x=w329) -> (.not. x?=w333:bool)
        n270 = local read "黄灯"() -> (w331:bool)
        n271 = Compound Arithmetic op=AND(w330, w333, w331) -> (w332:bool)
        n272 = case shown="真" w332 {
          frame False {
          }
          frame True {
            n273 = flat-sequence {
              tunnel: [w337] -> w335
              tunnel: w335 -> [w339]
              tunnel: [w339] -> w334
              tunnel: w334 -> [w346]
              frame #0 {
                n274 = local read "测头机构电机"() -> (w336:u32)
                n275 = call "PCI1220U运行.vi"("方向"=enum32{"Negative", "Positive"}."Negative" ("Direction"), "AxisHandle IN"=w336) -> ("AxisHandle OUT"=w337:u32)  [unwired: 9 in]
              }
              frame #1 {
                n276 = while {
                  stop <- w343 stop-if-true
                  n277 = local read "测头机构轴后退"() -> (w340:bool)
                  n278 = Wait (ms)(milliseconds to wait=u32 50 ("毫秒倍数")) -> ()  [unwired: 1 out]
                  n279 = Not(x=w340) -> (.not. x?=w344:bool)
                  n280 = local read "复位"() -> (w341:bool)
                  n281 = local read "红灯"() -> (w342:bool)
                  n282 = Compound Arithmetic op=OR(w341, w342, w344) -> (w343:bool)
                }
              }
              frame #2 {
                n283 = call "PCI1220U停止.vi"("AxisHandle IN"=w346) -> ()  [unwired: 9 in, 2 out]
              }
            }
          }
        }
      }
      frame #11 {
        n284 = local read "电动缸回零"() -> (w347:bool)
        n285 = case shown="真" w347 {
          frame False {
          }
          frame True {
            n286 = stacked-sequence {
              frame #0 {
                n287 = flat-sequence {
                  tunnel: [w363] -> w353
                  tunnel: [w356] -> w352
                  tunnel: w353 -> [w366]
                  tunnel: [w366] -> w351
                  tunnel: [w364] -> w350
                  tunnel: w352 -> [w364]
                  tunnel: w351 -> [w368]
                  tunnel: [w368] -> w349
                  tunnel: w350 -> [w367]
                  tunnel: [w367] -> w348
                  tunnel: w349 -> [w384]
                  tunnel: w348 -> [w383]
                  frame #0 {
                    n288 = local write "电动缸速度(mm/s)"(15.0 ("电动缸速度(mm/s)")) -> ()
                    n289 = local write "测头机构轴速度(mm/s)"(10.0 ("电动缸速度(mm/s)")) -> ()
                  }
                  frame #1 {
                    n290 = local read "测头机构电机"() -> (w360:u32)
                    n291 = local read "电动缸电机"() -> (w357:u32)
                    n292 = call <userlib>:"Acm_AxHome.vi"("DirMode"=u32 0, "HomeMode"=u32 11, "AxisHandle"=w360) -> ("AxisHandle"=w363:u32)  [unwired: 1 in, 2 out]
                    n293 = call <userlib>:"Acm_AxHome.vi"("DirMode"=u32 1, "HomeMode"=u32 11, "AxisHandle"=w357) -> ("AxisHandle"=w356:u32)  [unwired: 1 in, 2 out]
                  }
                  frame #2 {
                    n294 = Wait Until Next ms Multiple(millisecond multiple=u32 100 ("毫秒倍数")) -> ()  [unwired: 1 out]
                  }
                  frame #3 {
                    n295 = while {
                      tunnel: w368 -> [w382]
                      stop <- w378 stop-if-true
                      n296 = call <userlib>:"Acm_AxGetCmdVelocity.vi"("AxisHandle"=w382) -> ("Velocity"=w381:dbl)  [unwired: 1 in, 3 out]
                      n297 = Wait Until Next ms Multiple(millisecond multiple=u32 50 ("毫秒倍数")) -> ()  [unwired: 1 out]
                      n298 = Equal To 0?(x=w381) -> (x = 0?=w379:bool)
                      n299 = local read "急停"() -> (w376:bool)
                      n300 = local read "复位"() -> (w377:bool)
                      n301 = Compound Arithmetic op=OR(invert w376, w377, w379) -> (w378:bool)
                    }
                    n302 = while {
                      tunnel: w367 -> [w375]
                      stop <- w370 stop-if-true
                      n303 = call <userlib>:"Acm_AxGetCmdVelocity.vi"("AxisHandle"=w375) -> ("Velocity"=w374:dbl)  [unwired: 1 in, 3 out]
                      n304 = Wait Until Next ms Multiple(millisecond multiple=u32 50 ("毫秒倍数")) -> ()  [unwired: 1 out]
                      n305 = Equal To 0?(x=w374) -> (x = 0?=w369:bool)
                      n306 = local read "急停"() -> (w371:bool)
                      n307 = local read "复位"() -> (w372:bool)
                      n308 = Compound Arithmetic op=OR(invert w371, w372, w369) -> (w370:bool)
                    }
                  }
                  frame #4 {
                    n309 = call "PCI1220U角度置零.vi"("AxisHandle IN"=w384) -> ()  [unwired: 10 in, 1 out]
                    n310 = call "PCI1220U角度置零.vi"("AxisHandle IN"=w383) -> ()  [unwired: 10 in, 1 out]
                  }
                }
              }
              frame #1 {
                n311 = flat-sequence {
                  tunnel: [w396] -> w391
                  tunnel: w391 -> [w398]
                  tunnel: [w398] -> w390
                  tunnel: w390 -> [w399]
                  tunnel: [w399] -> w389
                  tunnel: w389 -> [w408]
                  tunnel: [w407] -> w386
                  tunnel: w386 -> [w410]
                  tunnel: [w410] -> w385
                  tunnel: w385 -> [w412]
                  tunnel: [w411] -> w388
                  tunnel: w388 -> [w421]
                  tunnel: [w421] -> w387
                  tunnel: w387 -> [w429]
                  frame #0 {
                    n312 = local write "旋转齿条轴速度(°/s)"(5.0 ("电动缸速度(mm/s)")) -> ()
                  }
                  frame #1 {
                    n313 = local read "旋转齿条电机"() -> (w393:u32)
                    n314 = call <userlib>:"Acm_AxHome.vi"("DirMode"=u32 0, "HomeMode"=u32 11, "AxisHandle"=w393) -> ("AxisHandle"=w396:u32)  [unwired: 1 in, 2 out]
                  }
                  frame #2 {
                    n315 = Wait Until Next ms Multiple(millisecond multiple=u32 100 ("毫秒倍数")) -> ()  [unwired: 1 out]
                  }
                  frame #3 {
                    n316 = while {
                      tunnel: w399 -> [w406]
                      stop <- w400 stop-if-true
                      n317 = call <userlib>:"Acm_AxGetCmdVelocity.vi"("AxisHandle"=w406) -> ("Velocity"=w405:dbl)  [unwired: 1 in, 3 out]
                      n318 = Wait Until Next ms Multiple(millisecond multiple=u32 50 ("毫秒倍数")) -> ()  [unwired: 1 out]
                      n319 = Equal To 0?(x=w405) -> (x = 0?=w401:bool)
                      n320 = local read "急停"() -> (w403:bool)
                      n321 = local read "复位"() -> (w402:bool)
                      n322 = Compound Arithmetic op=OR(invert w403, w402, w401) -> (w400:bool)
                    }
                  }
                  frame #4 {
                    n323 = call "PCI1220U角度置零.vi"("AxisHandle IN"=w408) -> ("AxisHandle OUT"=w407:u32)  [unwired: 10 in]
                  }
                  frame #5 {
                    n324 = Wait (ms)(milliseconds to wait=u32 100 ("等待时间（毫秒）")) -> ()  [unwired: 1 out]
                  }
                  frame #6 {
                    n325 = while {
                      tunnel: [w419] -> w411
                      tunnel: w412 -> [w417]
                      stop <- w414 stop-if-true
                      n326 = call "PCI1220U扭矩轴位置模式.vi"("Distance"=10.0, "AxisHandle IN"=w417) -> ("AbsSuccess"=w413:bool, "AxisHandle OUT"=w419:u32)  [unwired: 8 in]
                      n327 = Wait Until Next ms Multiple(millisecond multiple=u32 50 ("毫秒倍数")) -> ()  [unwired: 1 out]
                      n328 = local read "急停"() -> (w416:bool)
                      n329 = local read "复位"() -> (w415:bool)
                      n330 = Compound Arithmetic op=OR(invert w416, w415, w413) -> (w414:bool)
                    }
                  }
                  frame #7 {
                    n331 = while {
                      tunnel: w421 -> [w427]
                      stop <- w422 stop-if-true
                      n332 = call <userlib>:"Acm_AxGetCmdVelocity.vi"("AxisHandle"=w427) -> ("Velocity"=w428:dbl)  [unwired: 1 in, 3 out]
                      n333 = Wait Until Next ms Multiple(millisecond multiple=u32 50 ("毫秒倍数")) -> ()  [unwired: 1 out]
                      n334 = Equal To 0?(x=w428) -> (x = 0?=w423:bool)
                      n335 = local read "急停"() -> (w425:bool)
                      n336 = local read "复位"() -> (w424:bool)
                      n337 = Compound Arithmetic op=OR(w423, invert w425, w424) -> (w422:bool)
                    }
                  }
                  frame #8 {
                    n338 = call "PCI1220U角度置零.vi"("AxisHandle IN"=w429) -> ()  [unwired: 10 in, 1 out]
                  }
                }
              }
              frame #2 {
                n339 = flat-sequence {
                  frame #0 {
                    n340 = while {
                      stop <- w430 stop-if-true
                      n341 = local read "电动缸回零"() -> (w437:bool)
                      n342 = local write "回零完成"(TRUE ("回零完成")) -> ()
                      n343 = local write "电动缸回零"(FALSE ("电动缸回零")) -> ()
                      n344 = Wait Until Next ms Multiple(millisecond multiple=u32 50 ("毫秒倍数")) -> ()  [unwired: 1 out]
                      n345 = Not(x=w437) -> (.not. x?=w431:bool)
                      n346 = local read "急停"() -> (w432:bool)
                      n347 = local read "复位"() -> (w433:bool)
                      n348 = Compound Arithmetic op=OR(w431, invert w432, w433) -> (w430:bool)
                    }
                  }
                }
              }
            }
          }
        }
      }
    }
    n349 = Wait (ms)(milliseconds to wait=u32 50 ("毫秒倍数")) -> ()  [unwired: 1 out]
    n350 = local read "停止"() -> (w131:bool)
  }
  n351 = flat-sequence {
    tunnel: [w438] -> w4
    tunnel: w4 -> [w444]
    tunnel: [w443] -> w3
    tunnel: w3 -> [w510]
    frame #0 {
      n352 = call "PCI1240U初始化.vi"() -> ("旋转电机"=→"旋转齿条电机":u32, "电动缸电机"=→"电动缸电机":u32, "DeviceHandle"=→"DeviceHandle":u32, "进给电机"=→"测头机构电机":u32)  [unwired: 6 in, 2 out]
      n353 = call "PCI8622配置.vi"() -> ("DeviceID"=w438:i32)  [unwired: 11 in]
    }
    frame #1 {
      n354 = while {
        tunnel: w444 -> [w446]
        tunnel: [w445] -> w443
        stop <- "停止" stop-if-true
        n355 = stacked-sequence {
          tunnel: w446 -> [_ _ w486]
          tunnel: [_ _ w486] -> w445
          frame #0 {
            n356 = local read "测头机构电机"() -> (w455:u32)
            n357 = Boolean To (0,1)(Boolean="测头机构轴使能") -> (0, 1=w453:i16)
            n358 = call <userlib>:"Acm_AxSetSvOn.vi"("OnOff"=w453, "AxisHandle"=w455) -> ("AxisHandle"=w452:u32)  [unwired: 1 in, 2 out]
            n359 = call "PCI1220U进给轴速度设置.vi"("Change Velocity"="测头机构轴速度(mm/s)", "AxisHandle IN"=w452) -> ("AxisHandle OUT"=w450:u32)  [unwired: 9 in]
            n360 = call "PCI1220U进给轴读取位置.vi"("AxisHandle IN"=w450) -> ("位置"=→"测头机构轴位置(mm)":dbl)  [unwired: 9 in, 1 out]
          }
          frame #1 {
            n361 = local read "旋转齿条电机"() -> (w464:u32)
            n362 = local read "电动缸电机"() -> (w465:u32)
            n363 = Boolean To (0,1)(Boolean="电动缸使能") -> (0, 1=w469:i16)
            n364 = Boolean To (0,1)(Boolean="旋转齿条轴使能") -> (0, 1=w463:i16)
            n365 = call <userlib>:"Acm_AxSetSvOn.vi"("OnOff"=w469, "AxisHandle"=w465) -> ("AxisHandle"=w468:u32)  [unwired: 1 in, 2 out]
            n366 = call <userlib>:"Acm_AxSetSvOn.vi"("OnOff"=w463, "AxisHandle"=w464) -> ("AxisHandle"=w466:u32)  [unwired: 1 in, 2 out]
            n367 = call "PCI1240电动缸速度设置.vi"("Change Velocity"="电动缸速度(mm/s)", "AxisHandle IN"=w468) -> ("AxisHandle OUT"=w456:u32)  [unwired: 9 in]
            n368 = call "PCI1220U扭矩轴速度设置.vi"("Change Velocity"="旋转齿条轴速度(°/s)", "AxisHandle IN"=w466) -> ("AxisHandle OUT"=w467:u32)  [unwired: 9 in]
            n369 = call "PCI1240电动缸读取位置.vi"("AxisHandle IN"=w456) -> ("位置"=→"电动缸位置(mm)":dbl)  [unwired: 9 in, 1 out]
            n370 = call "PCI1220U扭矩轴读取位置.vi"("AxisHandle IN"=w467) -> ("位置"=→"旋转齿条轴位置(°)":dbl)  [unwired: 9 in, 1 out]
          }
          frame #2 {
            w502 = 0  # nRetSizeWords
            w503 = 2048  # nReadSizeWords
            # "hDevice"
            n371 = Initialize Array(u16 0, 2048 ("dimension size")) -> (w493:u16[])
            n372 = dll-call lib="PCI8622_32.dll" fn="PCI8622_ReadDeviceProAD_Npt" label="ReadDeviceProAD_Npt"("hDevice"=w486, "ADBuffer[]"=w493, "nReadSizeWords"=w503, "nRetSizeWords"=w502) -> ("ADBuffer[]"=w496:u16[])  [unwired: 7 in, 2 out]
            n373 = Divide(x=w496, y=65536.01) -> (x/y=w497:dbl[])
            n374 = Multiply(x=w497, y=20) -> (x*y=w500:dbl[])
            n375 = Subtract(x=w500, y=10) -> (x-y=w492:dbl[])
            n376 = Decimate 1D Array ("抽取一维数组")(w492) -> (w480:dbl[], w481:dbl[], w479:dbl[])  [unwired: 5 out]
            n377 = Add Array Elements(numeric array=w480) -> (sum=w489:dbl)
            n378 = Add Array Elements(numeric array=w481) -> (sum=w485:dbl)
            n379 = Add Array Elements(numeric array=w479) -> (sum=w490:dbl)
            n380 = Array Size(array=w480) -> (size(s)=w488:i32)
            n381 = Array Size(array=w481) -> (size(s)=w487:i32)
            n382 = Array Size(array=w479) -> (size(s)=w491:i32)
            n383 = local read "齿条推拉力比例偏移"() -> (w505:dbl)
            n384 = local read "齿条推拉力零点偏移"() -> (w504:dbl)
            n385 = local read "齿条扭矩比例偏移"() -> (w509:dbl)
            n386 = local read "齿条扭矩零点偏移"() -> (w508:dbl)
            n387 = Divide(x=w489, y=w488) -> (x/y=w478:dbl)
            n388 = Divide(x=w485, y=w487) -> (x/y=w475:dbl)
            n389 = Divide(x=w490, y=w491) -> (x/y=w472:dbl)
            n390 = local read "间隙位移比例偏移"() -> (w507:dbl)
            n391 = local read "间隙位移零点偏移"() -> (w506:dbl)
            n392 = Multiply(x=w478, y=2.0) -> (x*y=w473:dbl)
            n393 = Multiply(x=w475, y=200.0) -> (x*y=w474:dbl)
            n394 = Subtract(x=w472, y=4.43) -> (x-y=w470:dbl)
            n395 = call "传感器校订.vi"("零点"=w508, "比例"=w509, "传感器"=w473) -> ("示值"=→"齿条扭矩(Nm)":dbl)  [unwired: 8 in]
            n396 = call "传感器校订.vi"("零点"=w504, "比例"=w505, "传感器"=w474) -> ("示值"=→"齿条推拉力(N)":dbl)  [unwired: 8 in]
            n397 = call "传感器校订.vi"("零点"=w506, "比例"=w507, "传感器"=w470) -> ("示值"=→"间隙位移(mm)":dbl)  [unwired: 8 in]
          }
        }
        n398 = Wait Until Next ms Multiple(millisecond multiple=u32 50 ("毫秒倍数")) -> ()  [unwired: 1 out]
      }
    }
    frame #2 {
      n399 = dll-call lib="PCI8622_32.dll" fn="PCI8622_ReleaseDevice" label="ReleaseDevice"("hDevice"=w510) -> ()  [unwired: 5 in, 2 out]
      n400 = dll-call lib="PCI8622_32.dll" fn="PCI8622_StopDeviceProAD" label="StopDeviceProAD"("hDevice"=w510) -> ("hDevice"=w511:i32)  [unwired: 4 in, 2 out]
      n401 = dll-call lib="PCI8622_32.dll" fn="PCI8622_ReleaseDeviceProAD" label="ReleaseDeviceProAD"("hDevice"=w511) -> ()  [unwired: 5 in, 2 out]
    }
  }
  n402 = while {
    stop <- w512 stop-if-true
    n403 = Wait (ms)(milliseconds to wait=u32 50 ("毫秒倍数")) -> ()  [unwired: 1 out]
    n404 = event shown="[1] \"停止\": 值改变" {
      selector: _ -> [_ _ _ _ _ _]
      dyn-events: _ -> [_ _ _ _ _ _]
      timeout: 500 -> [_ _ _ _ _ _]
      event Timeout {
        n405 = event-data() -> ()  [unwired: 3 out]
      }
      event "停止": Value Change {
        n406 = event-data() -> ()  [unwired: 6 out]
        n407 = flat-sequence {
          frame #0 {
            n408 = Wait (ms)(milliseconds to wait=u32 1000 ("毫秒倍数")) -> ()  [unwired: 1 out]
          }
          frame #1 {
            n409 = Quit LabVIEW(quit? (T)=TRUE ("停止？(T)")) -> ()
          }
        }
      }
      event "参数修改": Value Change {
        n410 = event-data() -> ()  [unwired: 6 out]
        n411 = while {
          i -> [w519]
          stop <- w518 stop-if-true
          n412 = local read "参数浏览表"() -> (w521:string[][])
          n413 = local read "型号数量"() -> (w520:i32)
          n414 = Wait Until Next ms Multiple(millisecond multiple=u32 50 ("毫秒倍数")) -> ()  [unwired: 1 out]
          n415 = Greater Or Equal?(x=w519, y=w520) -> (x >= y?=w518:bool)
          n416 = Index Array(array=w521, index (col)=w519) -> (element=w517:string[])  [unwired: 1 in]
          n417 = stacked-sequence {
            tunnel: w517 -> [w557]
            frame #0 {
              n418 = Index Array(array=w557, index #1=0 ("索引"), index #2=2 ("索引"), index #3=3 ("索引"), index #4=4 ("索引"), index #5=5 ("索引"), index #6=6 ("索引"), index #7=7 ("索引"), index #8=8 ("索引"), index #9=9 ("索引"), index #10=10 ("索引"), index #11=11 ("索引"), index #12=12 ("索引"), index #13=13 ("索引"), index #14=14 ("索引"), index #15=15 ("索引"), index #16=16 ("索引"), index #17=17 ("索引"), index #18=18 ("索引"), index #19=19 ("索引"), index #20=20 ("索引")) -> (element #1=w524:string, element #2=w553:string, element #3=w552:string, element #4=w551:string, element #5=w550:string, element #6=w549:string, element #7=w548:string, element #8=w547:string, element #9=w546:string, element #10=w545:string, element #11=w544:string, element #12=w535:string, element #13=w534:string, element #14=w533:string, element #15=w532:string, element #16=w531:string, element #17=w530:string, element #18=w527:string, element #19=w526:string, element #20=w523:string)
              n419 = local read "ADODB._Connection Out 2"() -> (w542:refnum<k7>)
              n420 = call "创建文本"("测头机构轴移动速度"=w553, "测头机构轴检测位"=w552, "测头机构轴待检位"=w551, "测头机构轴后退位"=w550, "齿条移动速度"=w549, "齿条左极限"=w548, "齿条右极限"=w547, "旋转齿条轴找帽转速"=w546, "旋转齿条轴测量转速"=w545, "测量点扭矩"=w544, "总行程最小值"=w535, "总行程最大值"=w534, "最大轴向力"=w533, "轴向力波动"=w532, "平均轴向力最小值"=w531, "平均轴向力最大值"=w530, "总圈数最小值"=w527, "总圈数最大值"=w526, "中间位置"=w523, "产品型号"=w524) -> ("Result"=w543:string)  [unwired: 6 in, 1 out]
              n421 = call "SQL Execute.vi"("Command Text"=w543, "ADODB._Connection In"=w542) -> ("error out"=w555:errorcluster, "ADODB._Connection Out"=w556:refnum<k7>)  [unwired: 6 in, 2 out]
              n422 = call "ADO Connection Close.vi"("error in (no error)"=w555, "ADODB._Connection In"=w556) -> ("error out"=→"error out":errorcluster)  [unwired: 8 in, 1 out]
            }
          }
        }
      }
      event "参数查询": Value Change {
        n423 = event-data() -> ()  [unwired: 6 out]
        n424 = flat-sequence {
          tunnel: [w580] -> w573
          tunnel: [w579] -> w572
          tunnel: [w578] -> w569
          tunnel: w573 -> [w584]
          tunnel: w572 -> [w586]
          tunnel: [w586] -> w571
          tunnel: [w585] -> w570
          tunnel: w569 -> [w585]
          tunnel: w571 -> [_]
          tunnel: w570 -> [_]
          frame #0 {
            n425 = call-poly <vilib>:"Read From Spreadsheet File.vi"("file path (dialog if empty)"=path "D:/Q14070-Z060人机界面/参数/参数项.txt") -> ("first row"=w574:string[])  [unwired: 6 in, 4 out]
            n426 = property on="参数浏览表" class="Tbl (严格)"("Row Headers[]"=w574) -> ()  [unwired: 2 in, 2 out]
          }
          frame #1 {
            n427 = local read "ADODB._Connection Out 2"() -> (w577:refnum<k7>)
            n428 = call "SQL Execute.vi"("Command Text"="SELECT * FROM 测试参数表;", "ADODB._Connection In"=w577) -> ("error out"=w578:errorcluster, "Data"=w582:string[][], "ADODB._Connection Out"=w579:refnum<k7>)  [unwired: 6 in, 1 out]
            n429 = Transpose 2D Array "二维数组转置"(2D array=w582) -> (transposed array=w580:string[][])
            n430 = Index Array(array=w580, index (row)=0 ("索引 (行)")) -> (element=w581:string[])  [unwired: 1 in]
            n431 = property on="参数浏览表" class="Tbl (严格)"("Column Headers[]"=w581) -> ()  [unwired: 2 in, 2 out]
          }
          frame #2 {
            n432 = local write "参数浏览表"(w584) -> ()
          }
          frame #3 {
          }
        }
      }
      event "传感器参数保存": Value Change {
        n433 = event-data() -> ()  [unwired: 6 out]
        n434 = flat-sequence {
          frame #0 {
            n435 = local read "齿条推拉力零点偏移"() -> (w591:dbl)
            n436 = local read "齿条推拉力比例偏移"() -> (w587:dbl)
            n437 = local read "间隙位移零点偏移"() -> (w598:dbl)
            n438 = local read "齿条扭矩零点偏移"() -> (w590:dbl)
            n439 = local read "间隙位移比例偏移"() -> (w588:dbl)
            n440 = local read "齿条扭矩比例偏移"() -> (w589:dbl)
            n441 = local read "ADODB._Connection Out 2"() -> (w606:refnum<k7>)
            n442 = Number To Fractional String(number=w598, precision (6)=i16 2 ("精度(6)")) -> (F-format string=w605:string)  [unwired: 2 in]
            n443 = Number To Fractional String(number=w591, precision (6)=i16 2 ("精度(6)")) -> (F-format string=w604:string)  [unwired: 2 in]
            n444 = Number To Fractional String(number=w590, precision (6)=i16 2 ("精度(6)")) -> (F-format string=w603:string)  [unwired: 2 in]
            n445 = Number To Fractional String(number=w588, precision (6)=i16 2 ("精度(6)")) -> (F-format string=w602:string)  [unwired: 2 in]
            n446 = Number To Fractional String(number=w587, precision (6)=i16 2 ("精度(6)")) -> (F-format string=w601:string)  [unwired: 2 in]
            n447 = Number To Fractional String(number=w589, precision (6)=i16 2 ("精度(6)")) -> (F-format string=w600:string)  [unwired: 2 in]
            n448 = call "创建文本3"("4"=w602, "6"=w600, "1"=w605, "2"=w604, "3"=w603, "5"=w601) -> ("Result"=w607:string)  [unwired: 8 in, 1 out]
            n449 = call "SQL Execute.vi"("Command Text"=w607, "ADODB._Connection In"=w606) -> ("error out"=→"error out 4":errorcluster)  [unwired: 6 in, 3 out]
          }
        }
      }
      event "产品ID": Value Change {
        n450 = event-data() -> ()  [unwired: 7 out]
        n451 = Format Date/Time String(time format string (%c)="%Y%m%d%H%M" ("时间格式字符串(%c)")) -> (date/time string=w608:string)  [unwired: 2 in]
        n452 = local write "KSJJ"(w608) -> ()
      }
    }
    n453 = local read "停止"() -> (w512:bool)
  }
  n454 = while {
    stop <- w612 stop-if-true
    n455 = local read "工步号"() -> (w610:u32)
    n456 = Wait (ms)(milliseconds to wait=u32 50 ("毫秒倍数")) -> ()  [unwired: 1 out]
    n457 = case shown="15" w610 {
      frame 0, Default {
      }
      frame 10 {
        n458 = flat-sequence {
          frame #0 {
            w613 = 0.0 ("已调试次数")
            n459 = local write "测头气缸左移"(FALSE ("测头气缸左移")) -> ()
            n460 = local write "测头气缸右移"(TRUE ("测头气缸右移")) -> ()
            n461 = local write "旋转齿条轴使能"(TRUE ("旋转齿条轴使能")) -> ()
            n462 = local write "电动缸使能"(TRUE ("电动缸使能")) -> ()
            n463 = local write "测头机构轴使能"(TRUE ("调整机构轴使能")) -> ()
            n464 = local write "旋转齿条轴速度(°/s)"(10.0 ("旋转齿条轴速度(°/s)")) -> ()
            n465 = local write "电动缸速度(mm/s)"(10.0 ("电动缸速度(mm/s)")) -> ()
            n466 = local write "测头机构轴速度(mm/s)"(30.0 ("调整机构轴速度(mm/s)")) -> ()
            n467 = local write "单点间隙已调试次数"(w613) -> ()
            n468 = local write "轴向力已做次数"(w613) -> ()
          }
          frame #1 {
            n469 = while {
              stop <- w622 stop-if-true
              n470 = Wait Until Next ms Multiple(millisecond multiple=u32 50 ("毫秒倍数")) -> ()  [unwired: 1 out]
              n471 = local read "回零完成"() -> (w624:bool)
              n472 = local read "测头右位"() -> (w623:bool)
              n473 = And(x=w624, y=w623) -> (x .and. y?=w622:bool)
            }
          }
          frame #2 {
            n474 = Wait (ms)(milliseconds to wait=u32 1000 ("等待时间（毫秒）")) -> ()  [unwired: 1 out]
          }
          frame #3 {
            n475 = while {
              stop <- w630 stop-if-true
              n476 = Wait Until Next ms Multiple(millisecond multiple=u32 50 ("毫秒倍数")) -> ()  [unwired: 1 out]
              n477 = local read "测头机构轴待检位"() -> (w627:dbl)
              n478 = local read "测头机构电机"() -> (w628:u32)
              n479 = call "PCI1220U进给轴位置模式.vi"("Distance"=w627, "AxisHandle IN"=w628) -> ("AbsSuccess"=w630:bool)  [unwired: 8 in, 1 out]
            }
          }
          frame #4 {
            n480 = while {
              stop <- w633 stop-if-true
              n481 = Wait Until Next ms Multiple(millisecond multiple=u32 50 ("毫秒倍数")) -> ()  [unwired: 1 out]
              n482 = local read "测头机构电机"() -> (w631:u32)
              n483 = call <userlib>:"Acm_AxGetCmdVelocity.vi"("AxisHandle"=w631) -> ("Velocity"=w634:dbl)  [unwired: 1 in, 3 out]
              n484 = Equal To 0?(x=w634) -> (x = 0?=w633:bool)
            }
          }
          frame #5 {
            n485 = local write "工步号"(u32 15 ("工步号")) -> ()
          }
        }
      }
      frame 15 {
        n486 = flat-sequence {
          tunnel: [w648] -> w639
          tunnel: w639 -> [w750]
          tunnel: [w750] -> w637
          tunnel: w637 -> [w754]
          tunnel: [w754] -> w636
          tunnel: [w761] -> w642
          tunnel: ["转向器中心"] -> w641
          tunnel: w636 -> [w761]
          tunnel: w642 -> [w770]
          tunnel: w641 -> [w769]
          tunnel: [w768] -> w640
          tunnel: w640 -> [w777]
          tunnel: [w776] -> w638
          tunnel: w638 -> [w788]
          frame #0 {
            n487 = local write "扭矩到达"(FALSE ("扭矩到达")) -> ()
            n488 = local write "旋转齿条轴速度(°/s)"(10.0 ("旋转齿条轴速度(°/s)")) -> ()
            n489 = local write "选项卡控件"(T1."间隙测量" ("选项卡控件")) -> ()
            "找帽扭矩" <- 10.0 ("找帽扭矩")
          }
          frame #1 {
            n490 = while {
              stop <- w651 stop-if-true
              n491 = stacked-sequence {
                seq-local: [w653 _] -> [_ w694]
                seq-local: [w657 _] -> [_ w693]
                frame #0 {
                  n492 = local read "扭矩到达"() -> (w655:bool)
                  n493 = local read "旋转齿条电机"() -> (w654:u32)
                  n494 = local read "找帽扭矩"() -> (w653:dbl)
                  n495 = Not(x=w655) -> (.not. x?=w656:bool)
                  n496 = case shown="假" w656 {
                    tunnel: [w659 w660] -> w657
                    tunnel: w654 -> [w659 w664]
                    tunnel: w653 -> [_ w662]
                    frame False {
                      n497 = local write "电动缸速度(mm/s)"(15.0 ("电动缸速度(mm/s)")) -> ()
                    }
                    frame True {
                      n498 = flat-sequence {
                        tunnel: w664 -> [w666]
                        tunnel: [w665] -> w663
                        tunnel: w663 -> [w674]
                        tunnel: w662 -> [w673]
                        tunnel: [w672] -> w661
                        tunnel: w661 -> [w687]
                        tunnel: [w686] -> w660
                        frame #0 {
                          n499 = while {
                            tunnel: [w670] -> w665
                            tunnel: w666 -> [w667]
                            stop <- w669 stop-if-true
                            n500 = Wait Until Next ms Multiple(millisecond multiple=u32 50 ("毫秒倍数")) -> ()  [unwired: 1 out]
                            n501 = call "PCI1220U扭矩轴位置模式.vi"("Distance"=10.0, "AxisHandle IN"=w667) -> ("AbsSuccess"=w669:bool, "AxisHandle OUT"=w670:u32)  [unwired: 8 in]
                          }
                        }
                        frame #1 {
                          n502 = while {
                            tunnel: w674 -> [w684]
                            tunnel: w673 -> [w679]
                            tunnel: [w678] -> w672
                            stop <- w680 stop-if-true
                            n503 = Wait Until Next ms Multiple(millisecond multiple=u32 10 ("毫秒倍数")) -> ()  [unwired: 1 out]
                            n504 = local read "齿条扭矩(Nm)"() -> (w677:dbl)
                            n505 = Absolute Value(x=w677) -> (abs(x)=w682:dbl)
                            n506 = call <userlib>:"Acm_AxGetCmdVelocity.vi"("AxisHandle"=w684) -> ("Velocity"=w683:dbl, "AxisHandle"=w678:u32)  [unwired: 1 in, 2 out]
                            n507 = Equal To 0?(x=w683) -> (x = 0?=w681:bool)
                            n508 = Greater Or Equal?(x=w682, y=w679) -> (x >= y?=w676:bool)
                            n509 = local write "扭矩到达"(w676) -> ()
                            n510 = Or "或"(x=w676, y=w681) -> (x .or. y?=w680:bool)
                            n511 = Not(x=w676) -> (.not. x?=w675:bool)
                            n512 = local write "旋转齿条轴使能"(w675) -> ()
                          }
                        }
                        frame #2 {
                          n513 = while {
                            tunnel: w687 -> [w691]
                            tunnel: [w688] -> w686
                            stop <- w690 stop-if-true
                            n514 = call "PCI1220U停止.vi"("AxisHandle IN"=w691) -> ("完成"=w690:bool, "AxisHandle OUT"=w688:u32)  [unwired: 9 in]
                            n515 = Wait Until Next ms Multiple(millisecond multiple=u32 50 ("毫秒倍数")) -> ()  [unwired: 1 out]
                          }
                        }
                      }
                    }
                  }
                }
                frame #1 {
                  n516 = local read "扭矩到达"() -> (w692:bool)
                  n517 = Not(x=w692) -> (.not. x?=w695:bool)
                  n518 = case shown="真" w695 {
                    tunnel: w693 -> [_ w700]
                    tunnel: w694 -> [_ w698]
                    frame False {
                      n519 = local write "电动缸速度(mm/s)"(15.0 ("电动缸速度(mm/s)")) -> ()
                    }
                    frame True {
                      n520 = flat-sequence {
                        tunnel: w700 -> [w701]
                        tunnel: [w702] -> w699
                        tunnel: w699 -> [w710]
                        tunnel: w698 -> [w709]
                        tunnel: [w708] -> w697
                        tunnel: w697 -> [w722]
                        frame #0 {
                          n521 = while {
                            tunnel: [w706] -> w702
                            tunnel: w701 -> [w703]
                            stop <- w705 stop-if-true
                            n522 = Wait Until Next ms Multiple(millisecond multiple=u32 50 ("毫秒倍数")) -> ()  [unwired: 1 out]
                            n523 = call "PCI1220U扭矩轴位置模式.vi"("Distance"=-29.0, "AxisHandle IN"=w703) -> ("AbsSuccess"=w705:bool, "AxisHandle OUT"=w706:u32)  [unwired: 8 in]
                          }
                        }
                        frame #1 {
                          n524 = while {
                            tunnel: w710 -> [w720]
                            tunnel: [w715] -> w708
                            tunnel: w709 -> [w714]
                            stop <- w716 stop-if-true
                            n525 = Wait Until Next ms Multiple(millisecond multiple=u32 50 ("毫秒倍数")) -> ()  [unwired: 1 out]
                            n526 = local read "齿条扭矩(Nm)"() -> (w713:dbl)
                            n527 = Absolute Value(x=w713) -> (abs(x)=w718:dbl)
                            n528 = call <userlib>:"Acm_AxGetCmdVelocity.vi"("AxisHandle"=w720) -> ("Velocity"=w719:dbl, "AxisHandle"=w715:u32)  [unwired: 1 in, 2 out]
                            n529 = Equal To 0?(x=w719) -> (x = 0?=w717:bool)
                            n530 = Greater Or Equal?(x=w718, y=w714) -> (x >= y?=w711:bool)
                            n531 = local write "扭矩到达"(w711) -> ()
                            n532 = Or(x=w711, y=w717) -> (x .or. y?=w716:bool)
                            n533 = Not(x=w711) -> (.not. x?=w712:bool)
                            n534 = local write "旋转齿条轴使能"(w712) -> ()
                          }
                        }
                        frame #2 {
                          n535 = while {
                            tunnel: w722 -> [w726]
                            tunnel: [w723] -> _
                            stop <- w725 stop-if-true
                            n536 = call "PCI1220U停止.vi"("AxisHandle IN"=w726) -> ("完成"=w725:bool, "AxisHandle OUT"=w723:u32)  [unwired: 9 in]
                            n537 = Wait Until Next ms Multiple(millisecond multiple=u32 50 ("毫秒倍数")) -> ()  [unwired: 1 out]
                          }
                        }
                      }
                    }
                  }
                }
              }
              n538 = Wait Until Next ms Multiple(millisecond multiple=u32 50 ("毫秒倍数")) -> ()  [unwired: 1 out]
              n539 = local read "扭矩到达"() -> (w651:bool)
            }
            n540 = Wait Until Next ms Multiple(millisecond multiple=u32 50 ("毫秒倍数")) -> ()  [unwired: 1 out]
            n541 = flat-sequence {
              tunnel: [w728] -> w650
              tunnel: w650 -> [w734]
              tunnel: [w734] -> w647
              tunnel: [w743] -> w648
              tunnel: w647 -> [w743]
              frame #0 {
                n542 = local write "电动缸速度(mm/s)"(5.0 ("电动缸速度(mm/s)")) -> ()
              }
              frame #1 {
                n543 = while {
                  tunnel: [w732] -> w728
                  stop <- w731 stop-if-true
                  n544 = local read "电动缸电机"() -> (w733:u32)
                  n545 = local read "齿条左极限"() -> (w729:dbl)
                  n546 = Wait Until Next ms Multiple(millisecond multiple=u32 50 ("毫秒倍数")) -> ()  [unwired: 1 out]
                  n547 = call "PCI1240电动缸位置模式 .vi"("Distance"=w729, "AxisHandle IN"=w733) -> ("AbsSuccess"=w731:bool, "AxisHandle OUT"=w732:u32)  [unwired: 8 in]
                }
              }
              frame #2 {
                n548 = while {
                  tunnel: w734 -> [w741]
                  stop <- w738 stop-if-true
                  n549 = Wait Until Next ms Multiple(millisecond multiple=u32 50 ("毫秒倍数")) -> ()  [unwired: 1 out]
                  n550 = local read "齿条推拉力(N)"() -> (w737:dbl)
                  n551 = call <userlib>:"Acm_AxGetCmdVelocity.vi"("AxisHandle"=w741) -> ("Velocity"=w742:dbl)  [unwired: 1 in, 3 out]
                  n552 = Less Or Equal?(x=w737, y=-500.0) -> (x <= y?=w735:bool)
                  n553 = Equal To 0?(x=w742) -> (x = 0?=w739:bool)
                  n554 = Or(x=w739, y=w735) -> (x .or. y?=w738:bool)
                }
              }
              frame #3 {
                n555 = while {
                  tunnel: w743 -> [w747]
                  tunnel: [w744] -> _
                  stop <- w746 stop-if-true
                  n556 = call "PCI1220U停止.vi"("AxisHandle IN"=w747) -> ("完成"=w746:bool, "AxisHandle OUT"=w744:u32)  [unwired: 9 in]
                  n557 = Wait Until Next ms Multiple(millisecond multiple=u32 50 ("毫秒倍数")) -> ()  [unwired: 1 out]
                }
              }
            }
          }
          frame #2 {
            n558 = while {
              stop <- "找帽OK" stop-if-true
              n559 = Wait Until Next ms Multiple(millisecond multiple=u32 50 ("毫秒倍数")) -> ()  [unwired: 1 out]
            }
            n560 = local write "夹头松开"(FALSE ("夹头松开")) -> ()
            n561 = local write "夹头夹紧"(TRUE ("夹头夹紧")) -> ()
            n562 = Wait (ms)(milliseconds to wait=u32 1000 ("毫秒倍数")) -> ()  [unwired: 1 out]
          }
          frame #3 {
            n563 = while {
              stop <- w756 stop-if-true
              n564 = local read "夹头松开"() -> (w759:bool)
              n565 = Wait Until Next ms Multiple(millisecond multiple=u32 50 ("毫秒倍数")) -> ()  [unwired: 1 out]
              n566 = local read "夹头夹紧位"() -> (w757:bool)
              n567 = Not(x=w759) -> (.not. x?=w758:bool)
              n568 = And(x=w757, y=w758) -> (x .and. y?=w756:bool)
            }
          }
          frame #4 {
            n569 = disable-structure shown="禁用" {
              disable-tunnel: [w763 _] -> _
              frame Disabled {
                n570 = local read "齿条左极限"() -> (w767:dbl)
                n571 = local read "齿条右极限"() -> (w766:dbl)
                n572 = Add(x=w767, y=w766) -> (x+y=w765:dbl)
                n573 = Divide(x=w765, y=2.0) -> (x/y=w763:dbl)
              }
              frame Enabled {
              }
            }
            n574 = local write "电动缸速度(mm/s)"(15.0 ("电动缸轴移动速度")) -> ()
          }
          frame #5 {
            n575 = while {
              tunnel: w770 -> [w775]
              tunnel: w769 -> [w774]
              tunnel: [w771] -> w768
              stop <- w773 stop-if-true
              n576 = call "PCI1240电动缸位置模式 .vi"("Distance"=w774, "AxisHandle IN"=w775) -> ("AbsSuccess"=w773:bool, "AxisHandle OUT"=w771:u32)  [unwired: 8 in]
              n577 = Wait Until Next ms Multiple(millisecond multiple=u32 50 ("毫秒倍数")) -> ()  [unwired: 1 out]
            }
          }
          frame #6 {
            n578 = while {
              tunnel: w777 -> [w787]
              tunnel: [w778] -> w776
              stop <- w779 stop-if-true
              n579 = Wait Until Next ms Multiple(millisecond multiple=u32 50 ("毫秒倍数")) -> ()  [unwired: 1 out]
              n580 = local read "齿条推拉力(N)"() -> (w784:dbl)
              n581 = Absolute Value(x=w784) -> (abs(x)=w783:dbl)
              n582 = call <userlib>:"Acm_AxGetCmdVelocity.vi"("AxisHandle"=w787) -> ("Velocity"=w786:dbl, "AxisHandle"=w778:u32)  [unwired: 1 in, 2 out]
              n583 = Greater Or Equal?(x=w783, y=1500.0) -> (x >= y?=w780:bool)
              n584 = Equal To 0?(x=w786) -> (x = 0?=w781:bool)
              n585 = Or(x=w781, y=w780) -> (x .or. y?=w779:bool)
            }
          }
          frame #7 {
            n586 = while {
              tunnel: w788 -> [w792]
              tunnel: [w791] -> _
              stop <- w790 stop-if-true
              n587 = call "PCI1220U停止.vi"("AxisHandle IN"=w792) -> ("完成"=w790:bool, "AxisHandle OUT"=w791:u32)  [unwired: 9 in]
              n588 = Wait (ms)(milliseconds to wait=u32 50 ("毫秒倍数")) -> ()  [unwired: 1 out]
            }
          }
          frame #8 {
            n589 = local write "工步号"(u32 16 ("工步号")) -> ()
          }
        }
      }
      frame 16 {
        n590 = flat-sequence {
          tunnel: [w806] -> w803
          tunnel: [w805] -> w802
          tunnel: w803 -> [w809]
          tunnel: w802 -> [w808]
          tunnel: [w807] -> w801
          tunnel: w801 -> [w816]
          tunnel: [w816] -> w800
          tunnel: w800 -> [w818]
          tunnel: [w817] -> w799
          tunnel: w799 -> [w830]
          tunnel: [w829] -> w797
          tunnel: [w836] -> w798
          tunnel: w797 -> [w836]
          tunnel: w798 -> [w839]
          tunnel: [w838] -> w796
          tunnel: w796 -> [w851]
          tunnel: [w850] -> w794
          tunnel: [w857] -> w795
          tunnel: w794 -> [w857]
          tunnel: w795 -> [w859]
          frame #0 {
            n591 = local write "电动缸速度(mm/s)"(30.0 ("齿条移动速度")) -> ()
            n592 = local read "电动缸电机"() -> (w806:u32)
            n593 = local read "齿条左极限"() -> (w805:dbl)
          }
          frame #1 {
            n594 = while {
              tunnel: w809 -> [w814]
              tunnel: w808 -> [w813]
              tunnel: [w810] -> w807
              stop <- w812 stop-if-true
              n595 = call "PCI1240电动缸位置模式 .vi"("Distance"=w813, "AxisHandle IN"=w814) -> ("AbsSuccess"=w812:bool, "AxisHandle OUT"=w810:u32)  [unwired: 8 in]
              n596 = Wait Until Next ms Multiple(millisecond multiple=u32 50 ("毫秒倍数")) -> ()  [unwired: 1 out]
            }
          }
          frame #2 {
            n597 = Wait Until Next ms Multiple(millisecond multiple=u32 200 ("毫秒倍数")) -> ()  [unwired: 1 out]
          }
          frame #3 {
            n598 = while {
              tunnel: w818 -> [w828]
              tunnel: [w819] -> w817
              stop <- w820 stop-if-true
              n599 = Wait Until Next ms Multiple(millisecond multiple=u32 50 ("毫秒倍数")) -> ()  [unwired: 1 out]
              n600 = local read "齿条推拉力(N)"() -> (w825:dbl)
              n601 = Absolute Value(x=w825) -> (abs(x)=w824:dbl)
              n602 = call <userlib>:"Acm_AxGetCmdVelocity.vi"("AxisHandle"=w828) -> ("Velocity"=w827:dbl, "AxisHandle"=w819:u32)  [unwired: 1 in, 2 out]
              n603 = Greater Or Equal?(x=w824, y=1500.0) -> (x >= y?=w821:bool)
              n604 = Equal To 0?(x=w827) -> (x = 0?=w822:bool)
              n605 = Or(x=w822, y=w821) -> (x .or. y?=w820:bool)
            }
          }
          frame #4 {
            n606 = while {
              tunnel: w830 -> [w835]
              tunnel: [w832] -> w829
              stop <- w834 stop-if-true
              n607 = local read "齿条右极限"() -> (w831:dbl)
              n608 = Wait Until Next ms Multiple(millisecond multiple=u32 50 ("毫秒倍数")) -> ()  [unwired: 1 out]
              n609 = call "PCI1240电动缸位置模式 .vi"("Distance"=w831, "AxisHandle IN"=w835) -> ("AbsSuccess"=w834:bool, "AxisHandle OUT"=w832:u32)  [unwired: 8 in]
            }
          }
          frame #5 {
            n610 = Wait Until Next ms Multiple(millisecond multiple=u32 200 ("毫秒倍数")) -> ()  [unwired: 1 out]
          }
          frame #6 {
            n611 = while {
              tunnel: w839 -> [w849]
              tunnel: [w840] -> w838
              stop <- w841 stop-if-true
              n612 = Wait Until Next ms Multiple(millisecond multiple=u32 50 ("毫秒倍数")) -> ()  [unwired: 1 out]
              n613 = local read "齿条推拉力(N)"() -> (w846:dbl)
              n614 = Absolute Value(x=w846) -> (abs(x)=w845:dbl)
              n615 = call <userlib>:"Acm_AxGetCmdVelocity.vi"("AxisHandle"=w849) -> ("Velocity"=w848:dbl, "AxisHandle"=w840:u32)  [unwired: 1 in, 2 out]
              n616 = Greater Or Equal?(x=w845, y=1000.0) -> (x >= y?=w842:bool)
              n617 = Equal To 0?(x=w848) -> (x = 0?=w843:bool)
              n618 = Or(x=w843, y=w842) -> (x .or. y?=w841:bool)
            }
          }
          frame #7 {
            n619 = while {
              tunnel: w851 -> [w856]
              tunnel: [w853] -> w850
              stop <- w855 stop-if-true
              n620 = local read "转向器中心"() -> (w852:dbl)
              n621 = Wait Until Next ms Multiple(millisecond multiple=u32 50 ("毫秒倍数")) -> ()  [unwired: 1 out]
              n622 = call "PCI1240电动缸位置模式 .vi"("Distance"=w852, "AxisHandle IN"=w856) -> ("AbsSuccess"=w855:bool, "AxisHandle OUT"=w853:u32)  [unwired: 8 in]
            }
          }
          frame #8 {
            n623 = Wait Until Next ms Multiple(millisecond multiple=u32 200 ("毫秒倍数")) -> ()  [unwired: 1 out]
          }
          frame #9 {
            n624 = while {
              tunnel: w859 -> [w869]
              tunnel: [w860] -> _
              stop <- w861 stop-if-true
              n625 = Wait Until Next ms Multiple(millisecond multiple=u32 50 ("毫秒倍数")) -> ()  [unwired: 1 out]
              n626 = local read "齿条推拉力(N)"() -> (w866:dbl)
              n627 = Absolute Value(x=w866) -> (abs(x)=w865:dbl)
              n628 = call <userlib>:"Acm_AxGetCmdVelocity.vi"("AxisHandle"=w869) -> ("Velocity"=w868:dbl, "AxisHandle"=w860:u32)  [unwired: 1 in, 2 out]
              n629 = Greater Or Equal?(x=w865, y=1500.0) -> (x >= y?=w862:bool)
              n630 = Equal To 0?(x=w868) -> (x = 0?=w863:bool)
              n631 = Or(x=w863, y=w862) -> (x .or. y?=w861:bool)
            }
          }
          frame #10 {
            n632 = local write "工步号"(u32 20 ("工步号")) -> ()
          }
        }
      }
      frame 20 {
        n633 = flat-sequence {
          tunnel: [w899] -> w880
          tunnel: w880 -> [w905]
          tunnel: [w912] -> w876
          tunnel: w876 -> [w919]
          tunnel: [w919] -> w875
          tunnel: w875 -> [w927]
          tunnel: [w927] -> w874
          tunnel: w874 -> [w928]
          tunnel: [w934] -> w878
          tunnel: [w936] -> w879
          tunnel: w878 -> [w936]
          tunnel: [w938] -> w885
          tunnel: w879 -> [w938]
          tunnel: w885 -> [w945]
          tunnel: [w944] -> w884
          tunnel: [w949] -> w883
          tunnel: [w948] -> w882
          tunnel: w884 -> [w947]
          tunnel: [w947] -> w881
          tunnel: [w976] -> w888
          tunnel: [w973] -> w887
          tunnel: w883 -> [w973]
          tunnel: [w972] -> w886
          tunnel: w882 -> [w972]
          tunnel: w881 -> [w976]
          tunnel: w888 -> [w980]
          tunnel: [w979] -> w877
          tunnel: w887 -> [w977]
          tunnel: w886 -> [w978]
          tunnel: w877 -> [w986]
          tunnel: [w985] -> w872
          tunnel: w872 -> [w993]
          tunnel: [w993] -> w871
          tunnel: w871 -> [w995]
          tunnel: [w994] -> w873
          tunnel: w873 -> [w1005]
          frame #0 {
            n634 = local write "选项卡控件"(T1."间隙测量" ("选项卡控件")) -> ()
          }
          frame #1 {
            n635 = while {
              stop <- w890 stop-if-true
              n636 = Wait Until Next ms Multiple(millisecond multiple=u32 50 ("毫秒倍数")) -> ()  [unwired: 1 out]
              n637 = local read "夹头松开"() -> (w892:bool)
              n638 = local read "夹头夹紧位"() -> (w891:bool)
              n639 = Not(x=w892) -> (.not. x?=w893:bool)
              n640 = And(x=w891, y=w893) -> (x .and. y?=w890:bool)
            }
          }
          frame #2 {
            n641 = local read "转向器中心"() -> (w895:dbl)
            n642 = local read "电动缸电机"() -> (w898:u32)
            n643 = Add(x=w895, y=0.0) -> (x+y=w897:dbl)
            n644 = while {
              tunnel: w898 -> [w904]
              tunnel: w897 -> [w903]
              tunnel: [w900] -> w899
              stop <- w902 stop-if-true
              n645 = call "PCI1240电动缸位置模式 .vi"("Distance"=w903, "AxisHandle IN"=w904) -> ("AbsSuccess"=w902:bool, "AxisHandle OUT"=w900:u32)  [unwired: 8 in]
              n646 = Wait Until Next ms Multiple(millisecond multiple=u32 50 ("毫秒倍数")) -> ()  [unwired: 1 out]
            }
          }
          frame #3 {
            n647 = while {
              tunnel: w905 -> [w909]
              stop <- w907 stop-if-true
              n648 = call <userlib>:"Acm_AxGetCmdVelocity.vi"("AxisHandle"=w909) -> ("Velocity"=w908:dbl)  [unwired: 1 in, 3 out]
              n649 = Wait Until Next ms Multiple(millisecond multiple=u32 50 ("毫秒倍数")) -> ()  [unwired: 1 out]
              n650 = Equal To 0?(x=w908) -> (x = 0?=w907:bool)
            }
          }
          frame #4 {
            n651 = local write "测头机构轴速度(mm/s)"(30.0 ("测头机构轴速度(mm/s)")) -> ()
          }
          frame #5 {
            n652 = local read "测头机构轴检测位"() -> (w911:dbl)
            n653 = local read "测头机构电机"() -> (w913:u32)
            n654 = while {
              tunnel: w913 -> [w916]
              tunnel: w911 -> [w915]
              tunnel: [w914] -> w912
              stop <- w918 stop-if-true
              n655 = call "PCI1220U进给轴位置模式.vi"("Distance"=w915, "AxisHandle IN"=w916) -> ("AbsSuccess"=w918:bool, "AxisHandle OUT"=w914:u32)  [unwired: 8 in]
              n656 = Wait Until Next ms Multiple(millisecond multiple=u32 50 ("毫秒倍数")) -> ()  [unwired: 1 out]
            }
          }
          frame #6 {
            n657 = while {
              stop <- w922 stop-if-true
              n658 = local read "测头机构轴检测位"() -> (w924:dbl)
              n659 = Wait Until Next ms Multiple(millisecond multiple=u32 50 ("毫秒倍数")) -> ()  [unwired: 1 out]
              n660 = local read "测头机构轴位置(mm)"() -> (w921:dbl)
              n661 = Subtract(x=w924, y=20.0) -> (x-y=w920:dbl)
              n662 = Greater Or Equal?(x=w921, y=w920) -> (x >= y?=w922:bool)
            }
          }
          frame #7 {
            n663 = local write "测头机构轴速度(mm/s)"(10.0 ("测头机构轴速度(mm/s)")) -> ()
          }
          frame #8 {
            n664 = while {
              tunnel: w928 -> [w932]
              stop <- w930 stop-if-true
              n665 = call <userlib>:"Acm_AxGetCmdVelocity.vi"("AxisHandle"=w932) -> ("Velocity"=w931:dbl)  [unwired: 1 in, 3 out]
              n666 = Wait Until Next ms Multiple(millisecond multiple=u32 50 ("毫秒倍数")) -> ()  [unwired: 1 out]
              n667 = Equal To 0?(x=w931) -> (x = 0?=w930:bool)
            }
          }
          frame #9 {
            n668 = local write "旋转齿条轴使能"(TRUE ("旋转齿条轴使能")) -> ()
          }
          frame #10 {
            n669 = local read "旋转齿条电机"() -> (w934:u32)
            n670 = call "PCI1220U角度置零.vi"("AxisHandle IN"=w934) -> ()  [unwired: 10 in, 1 out]
          }
          frame #11 {
            n671 = local write "旋转齿条轴速度(°/s)"(1.0 ("旋转齿条轴速度(°/s)")) -> ()
            n672 = Wait Until Next ms Multiple(millisecond multiple=u32 2000 ("毫秒倍数")) -> ()  [unwired: 1 out]
          }
          frame #12 {
            n673 = while {
              i -> [w941]
              stop <- w939 stop-if-true
              n674 = local read "间隙位移(mm)"() -> (→"基准位移":dbl)
              n675 = Wait Until Next ms Multiple(millisecond multiple=u32 500 ("毫秒倍数")) -> ()  [unwired: 1 out]
              n676 = Greater Or Equal?(x=w941, y=4) -> (x >= y?=w939:bool)
            }
          }
          frame #13 {
            n677 = call "PCI1220U运行.vi"("方向"=enum32{"Negative", "Positive"}."Negative" ("Direction"), "AxisHandle IN"=w945) -> ("AxisHandle OUT"=w944:u32)  [unwired: 9 in]
          }
          frame #14 {
            w950 = dbl[] []
            n678 = while {
              shift-right: [w961] -> w949
              shift-left: w950 -> [w963]
              shift-right: [w960] -> w948
              shift-left: w950 -> [w962]
              stop <- w953 stop-if-true
              n679 = local read "间隙位移(mm)"() -> (w956:dbl)
              n680 = local read "齿条扭矩(Nm)"() -> (w957:dbl)
              n681 = Wait (ms)(milliseconds to wait=u32 10 ("毫秒倍数")) -> ()  [unwired: 1 out]
              n682 = local read "基准位移"() -> (w954:dbl)
              n683 = Subtract(x=w956, y=w954) -> (x-y=w955:dbl)
              n684 = Absolute Value(x=w957) -> (abs(x)=w952:dbl)
              n685 = Greater Or Equal?(x=w952, y="扭矩停止值") -> (x >= y?=w953:bool)
              n686 = Build Array (concatenate) ("创建数组")(w962, w955) -> (w960:dbl[])
              n687 = Build Array (concatenate) ("创建数组")(w963, w952) -> (w961:dbl[])
              n688 = Bundle ("捆绑")(w961, w960) -> (w958:cluster{dbl[], dbl[]})  [unwired: 1 in]
              n689 = Build Array ("创建数组")(w958) -> (w959:cluster{dbl[], dbl[]}[])
              n690 = local write "扭动曲线"(w959) -> ()
            }
          }
          frame #15 {
            n691 = Absolute Value(x=w973) -> (abs(x)=w974:dbl[])
            n692 = Array Max & Min(array=w972) -> (min value=w971:dbl)  [unwired: 3 out]
            n693 = local read "测量点扭矩"() -> (w975:dbl)
            n694 = local read "基准位移"() -> (w969:dbl)
            n695 = Absolute Value(x=w971) -> (abs(x)=w968:dbl)
            n696 = Subtract(x=w969, y=w968) -> (x-y=w967:dbl)
            n697 = call "自定义插值.vi"("压力"=w975, "扭矩数组"=w974, "位移数组"=w972) -> ("扭矩值"=w970:dbl)  [unwired: 8 in]
            n698 = Add(x=w968, y=w970) -> (x+y=w965:dbl)
            n699 = local write "基准位移"(w967) -> ()
            n700 = Absolute Value(x=w965) -> (abs(x)=w966:dbl)
            n701 = local write "中间位置间隙"(w966) -> ()
          }
          frame #16 {
            n702 = while {
              tunnel: w980 -> [w984]
              tunnel: [w983] -> w979
              stop <- w982 stop-if-true
              n703 = call "PCI1220U停止.vi"("AxisHandle IN"=w984) -> ("完成"=w982:bool, "AxisHandle OUT"=w983:u32)  [unwired: 9 in]
              n704 = Wait (ms)(milliseconds to wait=u32 50 ("毫秒倍数")) -> ()  [unwired: 1 out]
            }
            "间隙Y数组" <- w978
            "间隙X数组" <- w977
          }
          frame #17 {
            n705 = while {
              tunnel: [w991] -> w985
              tunnel: w986 -> [w989]
              stop <- w990 stop-if-true
              n706 = Wait Until Next ms Multiple(millisecond multiple=u32 50 ("毫秒倍数")) -> ()  [unwired: 1 out]
              n707 = call "PCI1220U扭矩轴位置模式.vi"("Distance"=0.0, "AxisHandle IN"=w989) -> ("AbsSuccess"=w990:bool, "AxisHandle OUT"=w991:u32)  [unwired: 8 in]
            }
          }
          frame #18 {
            n708 = Wait (ms)(milliseconds to wait=u32 500 ("等待时间（毫秒）")) -> ()  [unwired: 1 out]
          }
          frame #19 {
            n709 = while {
              tunnel: w995 -> [w1003]
              tunnel: [w999] -> w994
              stop <- w1000 stop-if-true
              n710 = Wait Until Next ms Multiple(millisecond multiple=u32 50 ("毫秒倍数")) -> ()  [unwired: 1 out]
              n711 = local read "齿条扭矩(Nm)"() -> (w998:dbl)
              n712 = call <userlib>:"Acm_AxGetCmdVelocity.vi"("AxisHandle"=w1003) -> ("Velocity"=w1004:dbl, "AxisHandle"=w999:u32)  [unwired: 1 in, 2 out]
              n713 = Equal To 0?(x=w1004) -> (x = 0?=w1001:bool)
              n714 = Greater Or Equal?(x=w998, y=3.0) -> (x >= y?=w996:bool)
              n715 = Or(x=w1001, y=w996) -> (x .or. y?=w1000:bool)
            }
          }
          frame #20 {
            n716 = while {
              tunnel: w1005 -> [w1009]
              tunnel: [w1008] -> _
              stop <- w1007 stop-if-true
              n717 = call "PCI1220U停止.vi"("AxisHandle IN"=w1009) -> ("完成"=w1007:bool, "AxisHandle OUT"=w1008:u32)  [unwired: 9 in]
              n718 = Wait (ms)(milliseconds to wait=u32 50 ("毫秒倍数")) -> ()  [unwired: 1 out]
            }
          }
          frame #21 {
            n719 = local write "旋转齿条轴使能"(FALSE ("旋转齿条轴使能")) -> ()
            n720 = Wait (ms)(milliseconds to wait=u32 500 ("毫秒倍数")) -> ()  [unwired: 1 out]
          }
          frame #22 {
            n721 = local write "工步号"(u32 25 ("工步号")) -> ()
          }
        }
      }
      frame 25 {
        n722 = flat-sequence {
          frame #0 {
            n723 = local read "中间位置最大间隙标准(mm)"() -> (w1014:dbl)
            n724 = local read "中间位置间隙"() -> (w1015:dbl)
            n725 = local read "最小间隙(mm)"() -> (w1013:dbl)
            n726 = In Range and Coerce(upper limit=w1014, x=w1015, lower limit=w1013) -> (In Range?=w1018:bool)  [unwired: 1 out]
            n727 = case shown="假" w1018 {
              tunnel: [FALSE ("本序合格") TRUE ("本序合格")] -> w1017
              tunnel: [w1023 0.0 ("需调整角度(度)")] -> w1016
              tunnel: w1015 -> [w1021 _]
              tunnel: w1014 -> [w1020 _]
              tunnel: w1013 -> [w1019 _]
              frame False {
                n728 = xnode "公式"("X"=w1021, "Xmax"=w1020, "Xmin"=w1019) -> ("结果"=w1023:dbl)  [unwired: 1 in, 1 out]
              }
              frame True {
              }
            }
            n729 = local write "需调整角度(度)"(w1016) -> ()
            n730 = local write "单点间隙合格"(w1017) -> ()
          }
          frame #1 {
            n731 = local read "单点间隙合格"() -> (w1038:bool)
            n732 = case shown="假" w1038 {
              frame False {
                n733 = local read "单点间隙已调试次数"() -> (w1041:dbl)
                n734 = Less?(x=w1041, y="间隙设定调整次数") -> (x < y?=w1040:bool)
                n735 = case shown="假" w1040 {
                  frame False {
                    n736 = local write "工步号"(u32 45 ("变更工步号")) -> ()
                  }
                  frame True {
                    n737 = local write "工步号"(u32 30 ("变更工步号")) -> ()
                  }
                }
              }
              frame True {
                n738 = local write "工步号"(u32 40 ("变更工步号")) -> ()
              }
            }
          }
        }
      }
      frame 30 {
        # "人工调整"
        n739 = flat-sequence {
          tunnel: [w1047] -> w1045
          tunnel: w1045 -> [w1054]
          frame #0 {
            n740 = local write "测头机构轴速度(mm/s)"(30.0 ("测头机构轴速度(mm/s)")) -> ()
          }
          frame #1 {
            n741 = local read "测头机构电机"() -> (w1048:u32)
            n742 = while {
              tunnel: w1048 -> [w1051]
              tunnel: [w1050] -> w1047
              stop <- w1053 stop-if-true
              n743 = Wait Until Next ms Multiple(millisecond multiple=u32 50 ("毫秒倍数")) -> ()  [unwired: 1 out]
              n744 = local read "测头机构轴待检位"() -> (w1049:dbl)
              n745 = call "PCI1220U进给轴位置模式.vi"("Distance"=w1049, "AxisHandle IN"=w1051) -> ("AbsSuccess"=w1053:bool, "AxisHandle OUT"=w1050:u32)  [unwired: 8 in]
            }
          }
          frame #2 {
            n746 = while {
              tunnel: w1054 -> [w1058]
              stop <- w1056 stop-if-true
              n747 = call <userlib>:"Acm_AxGetCmdVelocity.vi"("AxisHandle"=w1058) -> ("Velocity"=w1057:dbl)  [unwired: 1 in, 3 out]
              n748 = Wait Until Next ms Multiple(millisecond multiple=u32 50 ("毫秒倍数")) -> ()  [unwired: 1 out]
              n749 = Equal To 0?(x=w1057) -> (x = 0?=w1056:bool)
            }
          }
          frame #3 {
            n750 = while {
              stop <- w1060 stop-if-true
              n751 = Wait Until Next ms Multiple(millisecond multiple=u32 50 ("毫秒倍数")) -> ()  [unwired: 1 out]
              n752 = local read "测头机构轴位置(mm)"() -> (w1062:dbl)
              n753 = Less Or Equal?(x=w1062, y=35.0) -> (x <= y?=w1060:bool)
            }
          }
          frame #4 {
            n754 = local write "测头气缸左移"(TRUE ("测头气缸左移")) -> ()
            n755 = local write "测头气缸右移"(FALSE ("测头气缸右移")) -> ()
          }
          frame #5 {
            n756 = while {
              stop <- w1065 stop-if-true
              # "等待启动"
              n757 = local read "间隙启动"() -> (w1065:bool)
              n758 = Wait Until Next ms Multiple(millisecond multiple=u32 50 ("毫秒倍数")) -> ()  [unwired: 1 out]
            }
          }
          frame #6 {
            n759 = local read "不合格品"() -> (w1067:bool)
            n760 = case shown="真" w1067 {
              frame False {
                n761 = flat-sequence {
                  frame #0 {
                    n762 = local write "测头气缸右移"(TRUE ("测头气缸左移")) -> ()
                    n763 = local write "测头气缸左移"(FALSE ("测头气缸左移")) -> ()
                    n764 = local read "单点间隙已调试次数"() -> (w1070:dbl)
                    n765 = Add(x=w1070, y=1.0 ("已调试次数")) -> (x+y=w1072:dbl)
                    n766 = local write "单点间隙已调试次数"(w1072) -> ()
                  }
                  frame #1 {
                    n767 = while {
                      stop <- w1073 stop-if-true
                      n768 = Wait Until Next ms Multiple(millisecond multiple=u32 50 ("毫秒倍数")) -> ()  [unwired: 1 out]
                      n769 = local read "测头右位"() -> (w1073:bool)
                    }
                  }
                  frame #2 {
                    n770 = local write "工步号"(u32 20 ("工步号")) -> ()
                  }
                }
              }
              frame True {
                n771 = local write "工步号"(u32 45 ("工步号")) -> ()
              }
            }
          }
        }
      }
      frame 40 {
        n772 = flat-sequence {
          tunnel: [w1198] -> w1194
          tunnel: w1194 -> [w1200]
          tunnel: [w1199] -> w1193
          tunnel: w1193 -> [w1208]
          tunnel: [w1208] -> w1192
          tunnel: w1192 -> [w1220]
          tunnel: [w1220] -> w1191
          tunnel: w1191 -> [w1222]
          tunnel: [w1221] -> w1190
          tunnel: w1190 -> [w1230]
          tunnel: [w1230] -> w1189
          tunnel: w1189 -> [w1240]
          tunnel: [w1240] -> w1188
          tunnel: w1188 -> [w1248]
          tunnel: [w1248] -> w1187
          tunnel: w1187 -> [w1250]
          tunnel: [w1251] -> w1186
          tunnel: [w1249] -> w1185
          tunnel: w1186 -> [w1264]
          tunnel: w1185 -> [w1259]
          tunnel: [w1262] -> w1184
          tunnel: [w1261] -> w1183
          tunnel: [w1260] -> w1182
          tunnel: [w1259] -> w1181
          tunnel: [w1299] -> w1180
          tunnel: [w1302] -> w1179
          tunnel: w1184 -> [w1302]
          tunnel: [w1301] -> w1178
          tunnel: w1183 -> [w1301]
          tunnel: [w1300] -> w1177
          tunnel: w1182 -> [w1300]
          tunnel: w1181 -> [w1299]
          tunnel: w1180 -> [w1308]
          tunnel: [w1304] -> w1176
          tunnel: [w1307] -> w1175
          tunnel: w1179 -> [w1307]
          tunnel: [w1306] -> w1174
          tunnel: w1178 -> [w1306]
          tunnel: [w1305] -> w1173
          tunnel: w1177 -> [w1305]
          tunnel: [w1303] -> w1172
          tunnel: [w1323] -> w1168
          tunnel: [w1322] -> w1169
          tunnel: [w1321] -> w1170
          tunnel: w1176 -> [w1316]
          tunnel: w1175 -> [w1320]
          tunnel: w1174 -> [w1319]
          tunnel: w1173 -> [w1318]
          tunnel: w1172 -> [w1317]
          tunnel: [w1316] -> w1171
          tunnel: [w1374] -> w1167
          tunnel: [w1359] -> w1166
          tunnel: [w1373] -> w1165
          tunnel: [w1372] -> w1164
          tunnel: [w1371] -> w1163
          tunnel: [w1370] -> w1162
          tunnel: [w1369] -> w1161
          tunnel: w1171 -> [w1373]
          tunnel: w1170 -> [w1372]
          tunnel: w1169 -> [w1359]
          tunnel: w1168 -> [w1374]
          tunnel: [w1360] -> w1160
          tunnel: w1167 -> [w1396]
          tunnel: [w1396] -> w1159
          tunnel: w1166 -> [w1395]
          tunnel: [w1395] -> w1158
          tunnel: w1165 -> [w1394]
          tunnel: [w1383] -> w1157
          tunnel: [w1382] -> w1156
          tunnel: [w1393] -> w1155
          tunnel: w1164 -> [w1393]
          tunnel: w1163 -> [w1390]
          tunnel: w1162 -> [w1392]
          tunnel: w1161 -> [w1391]
          tunnel: [w1385] -> w1154
          tunnel: [w1384] -> w1153
          tunnel: w1160 -> [w1381]
          tunnel: w1159 -> [w1409]
          tunnel: w1158 -> [w1408]
          tunnel: w1157 -> [w1404]
          tunnel: w1156 -> [w1411]
          tunnel: [w1411] -> w1151
          tunnel: w1155 -> [w1410]
          tunnel: [w1406] -> w1150
          tunnel: w1154 -> [w1413]
          tunnel: [w1413] -> w1149
          tunnel: w1153 -> [w1412]
          tunnel: [w1412] -> w1148
          tunnel: [w1407] -> w1152
          tunnel: [w1405] -> w1147
          tunnel: [w1404] -> w1146
          tunnel: w1152 -> [w1456]
          tunnel: [w1456] -> w1145
          tunnel: [w1450] -> w1144
          tunnel: w1151 -> [w1455]
          tunnel: [w1455] -> w1143
          tunnel: w1150 -> [w1454]
          tunnel: [w1454] -> w1142
          tunnel: w1149 -> [w1453]
          tunnel: [w1453] -> w1141
          tunnel: w1148 -> [w1452]
          tunnel: [w1452] -> w1140
          tunnel: [w1451] -> w1139
          tunnel: w1147 -> [w1451]
          tunnel: w1146 -> [w1450]
          tunnel: w1145 -> [w1463]
          tunnel: [w1463] -> w1138
          tunnel: w1144 -> [w1457]
          tunnel: w1143 -> [w1462]
          tunnel: [w1462] -> w1137
          tunnel: w1142 -> [w1461]
          tunnel: [w1461] -> w1136
          tunnel: w1141 -> [w1460]
          tunnel: [w1460] -> w1135
          tunnel: w1140 -> [w1459]
          tunnel: [w1459] -> w1134
          tunnel: [w1457] -> w1133
          tunnel: [w1458] -> w1132
          tunnel: w1139 -> [w1458]
          tunnel: [w1479] -> w1131
          tunnel: [w1478] -> w1130
          tunnel: w1138 -> [w1471]
          tunnel: [w1470] -> w1129
          tunnel: w1137 -> [w1473]
          tunnel: [w1473] -> w1128
          tunnel: w1136 -> [w1474]
          tunnel: [w1477] -> w1127
          tunnel: w1135 -> [w1475]
          tunnel: w1134 -> [w1476]
          tunnel: [w1476] -> w1126
          tunnel: [w1475] -> w1125
          tunnel: w1133 -> [w1470]
          tunnel: w1132 -> [w1472]
          tunnel: w1131 -> [w1520]
          tunnel: w1130 -> [w1526]
          tunnel: [w1526] -> w1124
          tunnel: w1129 -> [w1523]
          tunnel: [w1523] -> w1123
          tunnel: w1128 -> [w1525]
          tunnel: [w1525] -> w1122
          tunnel: w1127 -> [w1524]
          tunnel: [w1524] -> w1121
          tunnel: [w1520] -> w1120
          tunnel: [w1519] -> w1119
          tunnel: [w1518] -> w1118
          tunnel: w1126 -> [w1516]
          tunnel: w1125 -> [w1517]
          tunnel: [w1517] -> w1117
          tunnel: [w1516] -> w1116
          tunnel: [w1515] -> w1115
          tunnel: w1124 -> [w1539]
          tunnel: [w1573] -> w1114
          tunnel: w1123 -> [w1573]
          tunnel: [w1572] -> w1113
          tunnel: w1122 -> [w1572]
          tunnel: w1121 -> [w1571]
          tunnel: [w1569] -> w1112
          tunnel: w1120 -> [w1568]
          tunnel: w1119 -> [w1566]
          tunnel: w1118 -> [w1565]
          tunnel: [w1563] -> w1111
          tunnel: [w1562] -> w1110
          tunnel: [w1561] -> w1109
          tunnel: [w1536] -> w1108
          tunnel: [w1535] -> w1107
          tunnel: w1117 -> [w1558]
          tunnel: w1116 -> [w1557]
          tunnel: [w1558] -> w1106
          tunnel: [w1557] -> w1105
          tunnel: [w1556] -> w1104
          tunnel: [w1555] -> w1103
          tunnel: [w1552] -> w1102
          tunnel: [w1547] -> w1101
          tunnel: [w1542] -> w1100
          tunnel: [w1534] -> w1099
          tunnel: w1115 -> [w1533]
          tunnel: w1114 -> [w1600]
          tunnel: [w1600] -> w1098
          tunnel: w1113 -> [_]
          tunnel: [w1597] -> w1097
          tunnel: w1112 -> [w1599]
          tunnel: [w1596] -> w1096
          tunnel: w1111 -> [w1595]
          tunnel: w1110 -> [w1594]
          tunnel: w1109 -> [w1593]
          tunnel: [w1592] -> w1095
          tunnel: [w1591] -> w1094
          tunnel: w1108 -> [w1590]
          tunnel: w1107 -> [w1589]
          tunnel: w1106 -> [w1585]
          tunnel: w1105 -> [w1584]
          tunnel: [w1585] -> w1093
          tunnel: [w1584] -> w1092
          tunnel: [w1583] -> w1091
          tunnel: [w1582] -> w1090
          tunnel: w1104 -> [w1582]
          tunnel: [w1581] -> w1089
          tunnel: w1103 -> [w1581]
          tunnel: [w1580] -> w1088
          tunnel: [w1579] -> w1087
          tunnel: w1102 -> [w1578]
          tunnel: [w1577] -> w1086
          tunnel: w1101 -> [w1577]
          tunnel: [w1576] -> w1085
          tunnel: w1100 -> [w1576]
          tunnel: w1099 -> [w1575]
          tunnel: w1098 -> [w1617]
          tunnel: [w1617] -> w1084
          tunnel: w1097 -> [w1616]
          tunnel: [w1616] -> w1083
          tunnel: w1096 -> [w1615]
          tunnel: [w1615] -> w1082
          tunnel: w1095 -> [w1610]
          tunnel: w1094 -> [w1609]
          tunnel: w1093 -> [w1612]
          tunnel: w1092 -> [w1611]
          tunnel: w1091 -> [w1608]
          tunnel: w1090 -> [w1607]
          tunnel: w1089 -> [w1606]
          tunnel: w1088 -> [w1605]
          tunnel: w1087 -> [w1604]
          tunnel: w1086 -> [w1602]
          tunnel: w1085 -> [w1601]
          tunnel: w1084 -> [w1631]
          tunnel: [w1630] -> w1081
          tunnel: w1083 -> [w1629]
          tunnel: w1082 -> [w1628]
          tunnel: [w1628] -> w1080
          tunnel: w1081 -> [w1638]
          tunnel: [w1638] -> w1079
          tunnel: w1080 -> [w1637]
          tunnel: [w1637] -> w1078
          tunnel: w1079 -> [w1645]
          tunnel: [w1644] -> w1077
          tunnel: w1078 -> [w1643]
          tunnel: w1077 -> [w1651]
          frame #0 {
            n773 = local read "电动缸快速"() -> (w1195:dbl)
            n774 = local write "单点间隙已调试次数"(0.0 ("单点间隙已调试次数")) -> ()
            n775 = local write "选项卡控件"(T1."轴向力测量" ("选项卡控件")) -> ()
            n776 = local write "电动缸速度(mm/s)"(w1195) -> ()
            n777 = local read "电动缸电机"() -> (w1198:u32)
          }
          frame #1 {
            n778 = while {
              tunnel: w1200 -> [w1207]
              tunnel: [w1206] -> w1199
              stop <- w1201 stop-if-true
              n779 = local read "齿条左极限"() -> (w1204:dbl)
              n780 = Wait (ms)(milliseconds to wait=u32 50 ("毫秒倍数")) -> ()  [unwired: 1 out]
              n781 = local read "循环退出"() -> (w1203:bool)
              n782 = call "PCI1240电动缸位置模式 .vi"("Distance"=w1204, "AxisHandle IN"=w1207) -> ("AbsSuccess"=w1202:bool, "AxisHandle OUT"=w1206:u32)  [unwired: 8 in]
              n783 = Compound Arithmetic op=OR(w1202, w1203) -> (w1201:bool)
            }
          }
          frame #2 {
            n784 = while {
              tunnel: w1208 -> [w1209]
              stop <- w1211 stop-if-true
              n785 = Wait (ms)(milliseconds to wait=u32 50 ("毫秒倍数")) -> ()  [unwired: 1 out]
              n786 = local read "齿条推拉力(N)"() -> (w1215:dbl)
              n787 = call <userlib>:"Acm_AxGetCmdVelocity.vi"("AxisHandle"=w1209) -> ("Velocity"=w1217:dbl)  [unwired: 1 in, 3 out]
              n788 = Less Or Equal?(x=w1215, y=-500.0) -> (x <= y?=w1212:bool)
              n789 = local read "循环退出"() -> (w1210:bool)
              n790 = Equal To 0?(x=w1217) -> (x = 0?=w1213:bool)
              n791 = Compound Arithmetic op=OR(w1213, w1212, w1210) -> (w1211:bool)
            }
          }
          frame #3 {
            n792 = Wait (ms)(milliseconds to wait=u32 100 ("等待时间（毫秒）")) -> ()  [unwired: 1 out]
            n793 = local read "电动缸慢速"() -> (w1218:dbl)
            n794 = local write "电动缸速度(mm/s)"(w1218) -> ()
          }
          frame #4 {
            n795 = while {
              tunnel: w1222 -> [w1229]
              tunnel: [w1227] -> w1221
              stop <- w1223 stop-if-true
              n796 = Wait (ms)(milliseconds to wait=u32 50 ("毫秒倍数")) -> ()  [unwired: 1 out]
              n797 = call "PCI1240电动缸位置模式 .vi"("Distance"=10000.0, "AxisHandle IN"=w1229) -> ("AbsSuccess"=w1224:bool, "AxisHandle OUT"=w1227:u32)  [unwired: 8 in]
              n798 = local read "循环退出"() -> (w1225:bool)
              n799 = Compound Arithmetic op=OR(w1224, w1225) -> (w1223:bool)
            }
          }
          frame #5 {
            n800 = while {
              tunnel: w1230 -> [w1231]
              stop <- w1233 stop-if-true
              n801 = Wait (ms)(milliseconds to wait=u32 50 ("毫秒倍数")) -> ()  [unwired: 1 out]
              n802 = local read "齿条推拉力(N)"() -> (w1237:dbl)
              n803 = call <userlib>:"Acm_AxGetCmdVelocity.vi"("AxisHandle"=w1231) -> ("Velocity"=w1239:dbl)  [unwired: 1 in, 3 out]
              n804 = local read "循环退出"() -> (w1232:bool)
              n805 = Less Or Equal?(x=w1237, y=-500.0) -> (x <= y?=w1234:bool)
              n806 = Equal To 0?(x=w1239) -> (x = 0?=w1235:bool)
              n807 = Compound Arithmetic op=OR(w1235, w1234, w1232) -> (w1233:bool)
            }
          }
          frame #6 {
            n808 = while {
              tunnel: w1240 -> [w1245]
              stop <- w1241 stop-if-true
              n809 = call "PCI1220U停止.vi"("AxisHandle IN"=w1245) -> ("完成"=w1242:bool)  [unwired: 9 in, 1 out]
              n810 = Wait (ms)(milliseconds to wait=u32 50 ("毫秒倍数")) -> ()  [unwired: 1 out]
              n811 = local read "循环退出"() -> (w1243:bool)
              n812 = Compound Arithmetic op=OR(w1242, w1243) -> (w1241:bool)
            }
          }
          frame #7 {
            n813 = local read "电动缸快速"() -> (w1246:dbl)
            n814 = Wait (ms)(milliseconds to wait=u32 100 ("毫秒倍数")) -> ()  [unwired: 1 out]
            n815 = local write "电动缸速度(mm/s)"(w1246) -> ()
          }
          frame #8 {
            n816 = while {
              tunnel: w1250 -> [w1258]
              tunnel: [w1256] -> w1249
              stop <- w1252 stop-if-true
              n817 = local read "齿条右极限"() -> (w1255:dbl)
              n818 = Wait (ms)(milliseconds to wait=u32 50 ("毫秒倍数")) -> ()  [unwired: 1 out]
              n819 = call "PCI1240电动缸位置模式 .vi"("Distance"=w1255, "AxisHandle IN"=w1258) -> ("AbsSuccess"=w1253:bool, "AxisHandle OUT"=w1256:u32)  [unwired: 8 in]
              n820 = local read "循环退出"() -> (w1254:bool)
              n821 = Compound Arithmetic op=OR(w1253, w1254) -> (w1252:bool)
            }
            n822 = local read "转向器中心"() -> (w1251:dbl)
          }
          frame #9 {
            w1263 = dbl[] []
            n823 = while {
              shift-right: [w1286] -> w1261
              shift-left: w1263 -> [w1296]
              shift-right: [w1294] -> w1262
              shift-left: w1263 -> [w1295]
              tunnel: w1259 -> [w1290]
              tunnel: w1264 -> [w1289]
              shift-right: [w1285] -> w1260
              shift-left: w1263 -> [w1287]
              stop <- w1279 stop-if-true
              n824 = call <userlib>:"Acm_AxGetCmdVelocity.vi"("AxisHandle"=w1290) -> ("Velocity"=w1284:dbl)  [unwired: 1 in, 3 out]
              n825 = local read "电动缸位置(mm)"() -> (w1266:dbl)
              n826 = local read "齿条推拉力(N)"() -> (w1282:dbl)
              n827 = local read "间隙位移(mm)"() -> (w1275:dbl)
              n828 = Wait (ms)(milliseconds to wait=u32 50 ("毫秒倍数")) -> ()  [unwired: 1 out]
              n829 = local read "基准位移"() -> (w1291:dbl)
              n830 = local read "中间位置间隙"() -> (w1276:dbl)
              n831 = local read "循环退出"() -> (w1265:bool)
              n832 = Subtract(x=w1266, y=w1289) -> (x-y=w1269:dbl)
              n833 = Subtract(x=w1275, y=w1291) -> (x-y=w1278:dbl)
              n834 = Equal To 0?(x=w1284) -> (x = 0?=w1281:bool)
              n835 = Greater Or Equal?(x=w1275, y=4.0) -> (x >= y?=w1273:bool)
              n836 = Less Or Equal?(x=w1275, y=-1.0) -> (x <= y?=w1274:bool)
              n837 = Greater Or Equal?(x=w1282, y=500.0) -> (x >= y?=w1280:bool)
              n838 = Or(x=w1273, y=w1274) -> (x .or. y?=w1272:bool)
              n839 = Add(x=w1278, y=w1276) -> (x+y=w1277:dbl)
              n840 = Compound Arithmetic op=OR(w1281, w1280, w1265) -> (w1279:bool)
              n841 = Multiply(x=w1269, y=1.0) -> (x*y=w1267:dbl)
              n842 = Build Array (concatenate) ("创建数组")(w1287, w1282) -> (w1285:dbl[])
              n843 = Build Array (concatenate) ("创建数组")(w1296, w1267) -> (w1286:dbl[])
              n844 = property on="间隙位移(mm)" class="DigNum (严格)"("Blinking"=w1272) -> ()  [unwired: 2 in, 2 out]
              n845 = Build Array (concatenate) ("创建数组")(w1295, w1277) -> (w1294:dbl[])
              n846 = Bundle ("捆绑")(w1286, w1285) -> (w1288:cluster{dbl[], dbl[]})  [unwired: 1 in]
              n847 = Bundle ("捆绑")(w1286, w1294) -> (w1292:cluster{dbl[], dbl[]})  [unwired: 1 in]
              n848 = Build Array ("创建数组")(w1292, w1288) -> (w1293:cluster{dbl[], dbl[]}[])
              n849 = local write "行程跳动曲线"(w1293) -> ()
            }
          }
          frame #10 {
            n850 = local read "电动缸慢速"() -> (w1298:dbl)
            n851 = local write "电动缸速度(mm/s)"(w1298) -> ()
          }
          frame #11 {
            n852 = while {
              tunnel: w1308 -> [w1315]
              tunnel: [w1313] -> w1304
              stop <- w1309 stop-if-true
              n853 = Wait (ms)(milliseconds to wait=u32 50 ("毫秒倍数")) -> ()  [unwired: 1 out]
              n854 = call "PCI1240电动缸位置模式 .vi"("Distance"=-10.0, "AxisHandle IN"=w1315) -> ("AbsSuccess"=w1310:bool, "AxisHandle OUT"=w1313:u32)  [unwired: 8 in]
              n855 = local read "循环退出"() -> (w1311:bool)
              n856 = Compound Arithmetic op=OR(w1310, w1311) -> (w1309:bool)
            }
            n857 = local read "转向器中心"() -> (w1303:dbl)
          }
          frame #12 {
            n858 = while {
              shift-right: [w1345] -> w1322
              shift-left: w1319 -> [w1355]
              shift-right: [w1353] -> w1323
              shift-left: w1320 -> [w1354]
              tunnel: w1316 -> [w1349]
              tunnel: w1317 -> [w1348]
              shift-right: [w1344] -> w1321
              shift-left: w1318 -> [w1346]
              stop <- w1338 stop-if-true
              n859 = call <userlib>:"Acm_AxGetCmdVelocity.vi"("AxisHandle"=w1349) -> ("Velocity"=w1343:dbl)  [unwired: 1 in, 3 out]
              n860 = local read "电动缸位置(mm)"() -> (w1325:dbl)
              n861 = local read "齿条推拉力(N)"() -> (w1341:dbl)
              n862 = local read "间隙位移(mm)"() -> (w1334:dbl)
              n863 = Wait (ms)(milliseconds to wait=u32 50 ("毫秒倍数")) -> ()  [unwired: 1 out]
              n864 = local read "基准位移"() -> (w1350:dbl)
              n865 = local read "中间位置间隙"() -> (w1335:dbl)
              n866 = local read "循环退出"() -> (w1324:bool)
              n867 = Subtract(x=w1325, y=w1348) -> (x-y=w1328:dbl)
              n868 = Subtract(x=w1334, y=w1350) -> (x-y=w1337:dbl)
              n869 = Equal To 0?(x=w1343) -> (x = 0?=w1340:bool)
              n870 = Greater Or Equal?(x=w1334, y=4.0) -> (x >= y?=w1332:bool)
              n871 = Less Or Equal?(x=w1334, y=-1.0) -> (x <= y?=w1333:bool)
              n872 = Greater Or Equal?(x=w1341, y=500.0) -> (x >= y?=w1339:bool)
              n873 = Or(x=w1332, y=w1333) -> (x .or. y?=w1331:bool)
              n874 = Add(x=w1337, y=w1335) -> (x+y=w1336:dbl)
              n875 = Compound Arithmetic op=OR(w1340, w1339, w1324) -> (w1338:bool)
              n876 = Multiply(x=w1328, y=1.0) -> (x*y=w1326:dbl)
              n877 = Build Array (concatenate) ("创建数组")(w1355, w1326) -> (w1345:dbl[])
              n878 = Build Array (concatenate) ("创建数组")(w1346, w1341) -> (w1344:dbl[])
              n879 = Build Array (concatenate) ("创建数组")(w1354, w1336) -> (w1353:dbl[])
              n880 = property on="间隙位移(mm)" class="DigNum (严格)"("Blinking"=w1331) -> ()  [unwired: 2 in, 2 out]
              n881 = Bundle ("捆绑")(w1345, w1353) -> (w1351:cluster{dbl[], dbl[]})  [unwired: 1 in]
              n882 = Bundle ("捆绑")(w1345, w1344) -> (w1347:cluster{dbl[], dbl[]})  [unwired: 1 in]
              n883 = Build Array ("创建数组")(w1351, w1347) -> (w1352:cluster{dbl[], dbl[]}[])
              n884 = local write "行程跳动曲线"(w1352) -> ()
            }
          }
          frame #13 {
            n885 = while {
              tunnel: w1373 -> [w1380]
              tunnel: [w1379] -> _
              stop <- w1375 stop-if-true
              n886 = call "PCI1220U停止.vi"("AxisHandle IN"=w1380) -> ("完成"=w1376:bool, "AxisHandle OUT"=w1379:u32)  [unwired: 9 in]
              n887 = Wait (ms)(milliseconds to wait=u32 50 ("毫秒倍数")) -> ()  [unwired: 1 out]
              n888 = local read "循环退出"() -> (w1377:bool)
              n889 = Compound Arithmetic op=OR(w1376, w1377) -> (w1375:bool)
            }
            n890 = Array Size(array=w1359) -> (size(s)=w1358:i32)
            n891 = call "间隙计算.vi"("扭矩数组"=w1374) -> ("峰值间隙1"=w1368:dbl, "峰值间隙2"=w1367:dbl)  [unwired: 6 in, 3 out]
            n892 = local read "电动缸快速"() -> (w1357:dbl)
            n893 = local write "左轴向力数组大小"(w1358) -> ()
            n894 = local write "左180°内全行程间隙"(w1368) -> ()
            n895 = local write "左180°外全行程间隙"(w1367) -> ()
            n896 = local read "180°内全行程间隙标准(mm)"() -> (w1366:dbl)
            n897 = local read "180°外全行程间隙标准(mm)"() -> (w1363:dbl)
            n898 = local write "电动缸速度(mm/s)"(w1357) -> ()
            n899 = Greater?(x=w1368, y=w1366) -> (0:w1365:bool)
            n900 = Greater?(x=w1367, y=w1363) -> (0:w1364:bool)
            n901 = call "功能计算_何 截取位移左.vi"("位移数组"=w1359, "拉压力数组"=w1372, "半行程"="半行程", "截取百分比"="截取百分比") -> ("峰值扭矩"=w1371:dbl, "平均扭矩"=w1370:dbl, "扭差"=w1369:dbl)  [unwired: 12 in, 1 out]
            "左轴向力波动(N)" <- w1369
            "左最大轴向力(N)" <- w1371
            n902 = local write "左平均轴向力(N)"(w1370) -> ()
            n903 = property on="左180°内全行程间隙" class="DigNum (严格)"("Blinking"=w1365) -> ()  [unwired: 2 in, 2 out]
            n904 = property on="左180°外全行程间隙" class="DigNum (严格)"("Blinking"=w1364) -> ()  [unwired: 2 in, 2 out]
            n905 = local read "最大轴向力标准(N)"() -> (w1360:dbl)
            "左位移数组" <- w1359
            "左拉压力数组" <- w1372
          }
          frame #14 {
            n906 = while {
              tunnel: w1394 -> [w1403]
              tunnel: [w1400] -> w1383
              stop <- w1397 stop-if-true
              n907 = local read "齿条左极限"() -> (w1401:dbl)
              n908 = Wait (ms)(milliseconds to wait=u32 50 ("毫秒倍数")) -> ()  [unwired: 1 out]
              n909 = call "PCI1240电动缸位置模式 .vi"("Distance"=w1401, "AxisHandle IN"=w1403) -> ("AbsSuccess"=w1398:bool, "AxisHandle OUT"=w1400:u32)  [unwired: 8 in]
              n910 = local read "循环退出"() -> (w1399:bool)
              n911 = Compound Arithmetic op=OR(w1398, w1399) -> (w1397:bool)
            }
            n912 = local read "平均轴向力标准(N) max"() -> (w1387:dbl)
            n913 = local read "轴向力标准(N)"() -> (w1388:dbl)
            n914 = local read "力波动标准(N)"() -> (w1386:dbl)
            n915 = call "判断.vi"("y 3"=w1386, "y 2-2"=w1387, "y 2-1"=w1388, "y"=w1381, "x 3"=w1391, "x 2"=w1392, "x"=w1390) -> ("非x? 3"=w1384:bool, "非x? 2"=w1389:bool, "非x?"=w1385:bool)  [unwired: 2 in]
            n916 = property on="左最大轴向力(N)" class="DigNum (严格)"("Blinking"=w1385) -> ()  [unwired: 2 in, 2 out]
            n917 = property on="左平均轴向力(N)" class="DigNum (严格)"("Blinking"=w1389) -> ()  [unwired: 2 in, 2 out]
            n918 = property on="左轴向力波动(N)" class="DigNum (严格)"("Blinking"=w1384) -> ()  [unwired: 2 in, 2 out]
            n919 = local read "转向器中心"() -> (w1382:dbl)
          }
          frame #15 {
            n920 = while {
              shift-right: [w1438] -> w1405
              shift-left: w1408 -> [w1447]
              shift-right: [w1445] -> w1407
              shift-left: w1409 -> [w1446]
              tunnel: w1404 -> [w1440]
              tunnel: w1411 -> [w1439]
              shift-right: [w1435] -> w1406
              shift-left: w1410 -> [w1436]
              stop <- w1430 stop-if-true
              n921 = call <userlib>:"Acm_AxGetCmdVelocity.vi"("AxisHandle"=w1440) -> ("Velocity"=w1428:dbl)  [unwired: 1 in, 3 out]
              n922 = local read "电动缸位置(mm)"() -> (w1415:dbl)
              n923 = local read "齿条推拉力(N)"() -> (w1434:dbl)
              n924 = Wait (ms)(milliseconds to wait=u32 50 ("毫秒倍数")) -> ()  [unwired: 1 out]
              n925 = local read "间隙位移(mm)"() -> (w1422:dbl)
              n926 = local read "循环退出"() -> (w1414:bool)
              n927 = local read "基准位移"() -> (w1441:dbl)
              n928 = Add(x=1.47, y=w1415) -> (x+y=w1417:dbl)
              n929 = Less Or Equal?(x=w1434, y=-500.0) -> (x <= y?=w1431:bool)
              n930 = Equal To 0?(x=w1428) -> (x = 0?=w1432:bool)
              n931 = local read "中间位置间隙"() -> (w1427:dbl)
              n932 = Subtract(x=w1417, y=w1439) -> (x-y=w1420:dbl)
              n933 = Subtract(x=w1422, y=w1441) -> (x-y=w1442:dbl)
              n934 = Compound Arithmetic op=OR(w1432, w1431, w1414) -> (w1430:bool)
              n935 = Greater Or Equal?(x=w1422, y=4.0) -> (x >= y?=w1425:bool)
              n936 = Less Or Equal?(x=w1422, y=-1.0) -> (x <= y?=w1426:bool)
              n937 = Or(x=w1425, y=w1426) -> (x .or. y?=w1421:bool)
              n938 = Add(x=w1442, y=w1427) -> (x+y=w1429:dbl)
              n939 = Multiply(x=w1420, y=1.0) -> (x*y=w1418:dbl)
              n940 = property on="间隙位移(mm)" class="DigNum (严格)"("Blinking"=w1421) -> ()  [unwired: 2 in, 2 out]
              n941 = Build Array (concatenate) ("创建数组")(w1447, w1418) -> (w1438:dbl[])
              n942 = Build Array (concatenate) ("创建数组")(w1436, w1434) -> (w1435:dbl[])
              n943 = Build Array (concatenate) ("创建数组")(w1446, w1429) -> (w1445:dbl[])
              n944 = Bundle ("捆绑")(w1438, w1445) -> (w1443:cluster{dbl[], dbl[]})  [unwired: 1 in]
              n945 = Bundle ("捆绑")(w1438, w1435) -> (w1437:cluster{dbl[], dbl[]})  [unwired: 1 in]
              n946 = Build Array ("创建数组")(w1443, w1437) -> (w1444:cluster{dbl[], dbl[]}[])
              n947 = local write "行程跳动曲线"(w1444) -> ()
            }
          }
          frame #16 {
            n948 = local read "电动缸慢速"() -> (w1449:dbl)
            n949 = local write "电动缸速度(mm/s)"(w1449) -> ()
          }
          frame #17 {
            n950 = while {
              tunnel: w1457 -> [w1469]
              stop <- w1464 stop-if-true
              n951 = Wait (ms)(milliseconds to wait=u32 50 ("毫秒倍数")) -> ()  [unwired: 1 out]
              n952 = call "PCI1240电动缸位置模式 .vi"("Distance"=160.0, "AxisHandle IN"=w1469) -> ("AbsSuccess"=w1465:bool)  [unwired: 8 in, 1 out]
              n953 = local read "循环退出"() -> (w1466:bool)
              n954 = Compound Arithmetic op=OR(w1465, w1466) -> (w1464:bool)
            }
          }
          frame #18 {
            n955 = while {
              shift-right: [w1504] -> w1478
              shift-left: w1472 -> [w1513]
              shift-right: [w1511] -> w1479
              shift-left: w1471 -> [w1512]
              tunnel: w1470 -> [w1506]
              tunnel: w1473 -> [w1505]
              shift-right: [w1501] -> w1477
              shift-left: w1474 -> [w1502]
              stop <- w1496 stop-if-true
              n956 = call <userlib>:"Acm_AxGetCmdVelocity.vi"("AxisHandle"=w1506) -> ("Velocity"=w1494:dbl)  [unwired: 1 in, 3 out]
              n957 = local read "电动缸位置(mm)"() -> (w1481:dbl)
              n958 = local read "齿条推拉力(N)"() -> (w1500:dbl)
              n959 = Wait (ms)(milliseconds to wait=u32 50 ("毫秒倍数")) -> ()  [unwired: 1 out]
              n960 = local read "间隙位移(mm)"() -> (w1488:dbl)
              n961 = local read "循环退出"() -> (w1480:bool)
              n962 = local read "基准位移"() -> (w1507:dbl)
              n963 = Add(x=1.45, y=w1481) -> (x+y=w1483:dbl)
              n964 = Less Or Equal?(x=w1500, y=-500.0) -> (x <= y?=w1497:bool)
              n965 = Equal To 0?(x=w1494) -> (x = 0?=w1498:bool)
              n966 = local read "中间位置间隙"() -> (w1493:dbl)
              n967 = Subtract(x=w1483, y=w1505) -> (x-y=w1486:dbl)
              n968 = Subtract(x=w1488, y=w1507) -> (x-y=w1508:dbl)
              n969 = Compound Arithmetic op=OR(w1498, w1497, w1480) -> (w1496:bool)
              n970 = Greater Or Equal?(x=w1488, y=4.0) -> (x >= y?=w1491:bool)
              n971 = Less Or Equal?(x=w1488, y=-1.0) -> (x <= y?=w1492:bool)
              n972 = Or(x=w1491, y=w1492) -> (x .or. y?=w1487:bool)
              n973 = Add(x=w1508, y=w1493) -> (x+y=w1495:dbl)
              n974 = Multiply(x=w1486, y=1.0) -> (x*y=w1484:dbl)
              n975 = property on="间隙位移(mm)" class="DigNum (严格)"("Blinking"=w1487) -> ()  [unwired: 2 in, 2 out]
              n976 = Build Array (concatenate) ("创建数组")(w1513, w1484) -> (w1504:dbl[])
              n977 = Build Array (concatenate) ("创建数组")(w1502, w1500) -> (w1501:dbl[])
              n978 = Build Array (concatenate) ("创建数组")(w1512, w1495) -> (w1511:dbl[])
              n979 = Bundle ("捆绑")(w1504, w1511) -> (w1509:cluster{dbl[], dbl[]})  [unwired: 1 in]
              n980 = Bundle ("捆绑")(w1504, w1501) -> (w1503:cluster{dbl[], dbl[]})  [unwired: 1 in]
              n981 = Build Array ("创建数组")(w1509, w1503) -> (w1510:cluster{dbl[], dbl[]}[])
              n982 = local write "行程跳动曲线"(w1510) -> ()
            }
          }
          frame #19 {
            n983 = while {
              tunnel: w1523 -> [w1532]
              tunnel: [w1531] -> _
              stop <- w1527 stop-if-true
              n984 = call "PCI1220U停止.vi"("AxisHandle IN"=w1532) -> ("完成"=w1528:bool, "AxisHandle OUT"=w1531:u32)  [unwired: 9 in]
              n985 = Wait (ms)(milliseconds to wait=u32 50 ("毫秒倍数")) -> ()  [unwired: 1 out]
              n986 = local read "循环退出"() -> (w1529:bool)
              n987 = Compound Arithmetic op=OR(w1528, w1529) -> (w1527:bool)
            }
            n988 = Array Max & Min(array=w1520) -> (max value=w1522:dbl, min value=w1521:dbl)  [unwired: 2 out]
            n989 = Absolute Value(x=w1522) -> (abs(x)=w1519:dbl)
            n990 = Absolute Value(x=w1521) -> (abs(x)=w1518:dbl)
            n991 = local write "左全行程间隙"(w1519) -> ()
            n992 = local write "右全行程间隙"(w1518) -> ()
            n993 = local read "左轴向力数组大小"() -> (w1515:i32)
          }
          frame #20 {
            n994 = local read "截取百分比"() -> (w1537:dbl)
            n995 = local read "半行程"() -> (w1538:dbl)
            n996 = Split 1D Array(array=w1568, index=w1533) -> (second subarray=w1567:dbl[])  [unwired: 1 out]
            n997 = Array Max & Min(array=w1539) -> (max value=w1560:dbl, min value=w1559:dbl)  [unwired: 2 out]
            n998 = Split 1D Array(array=w1539, index=w1533) -> (second subarray=w1540:dbl[])  [unwired: 1 out]
            "右位移数组" <- w1540
            n999 = Split 1D Array(array=w1571, index=w1533) -> (second subarray=w1570:dbl[])  [unwired: 1 out]
            "右拉压力数组" <- w1570
            n1000 = local read "机械间隙值"() -> (w1553:dbl)
            n1001 = local read "180°内全行程间隙标准(mm)"() -> (w1564:dbl)
            n1002 = local read "总行程标准(mm)"() -> (w1549:dbl)
            n1003 = Subtract(x=w1560, y=w1559) -> (x-y=w1554:dbl)
            n1004 = call "功能计算_何 截取位移右.vi"("位移数组"=w1540, "拉压力数组"=w1570, "半行程"=w1538, "截取百分比"=w1537) -> ("峰值扭矩"=w1536:dbl, "平均扭矩"=w1569:dbl, "扭差"=w1535:dbl)  [unwired: 12 in, 1 out]
            "右最大轴向力(N)" <- w1536
            "右轴向力波动(N)" <- w1535
            n1005 = local read "总行程最大值"() -> (w1550:dbl)
            n1006 = call "间隙计算.vi"("扭矩数组"=w1567) -> ("峰值间隙1"=w1562:dbl, "峰值间隙2"=w1561:dbl)  [unwired: 6 in, 3 out]
            n1007 = local read "齿条传动比"() -> (w1541:dbl)
            n1008 = local write "右平均轴向力(N)"(w1569) -> ()
            n1009 = local write "右180°内全行程间隙"(w1562) -> ()
            n1010 = local write "右180°外全行程间隙"(w1561) -> ()
            n1011 = Subtract(x=w1554, y=w1553) -> (x-y=w1551:dbl)
            n1012 = local read "总圈数最大值"() -> (w1546:dbl)
            n1013 = local read "总圈数标准"() -> (w1545:dbl)
            n1014 = local write "总行程"(w1551) -> ()
            n1015 = In Range and Coerce(upper limit=w1550, x=w1551, lower limit=w1549) -> (In Range?=w1548:bool)  [unwired: 1 out]
            n1016 = Divide(x=w1551, y=w1541) -> (x/y=w1544:dbl)
            n1017 = local read "180°外全行程间隙标准(mm)"() -> (w1552:dbl)
            n1018 = local read "180°内全行程间隙标准(mm)"() -> (w1563:dbl)
            n1019 = local write "总圈数"(w1544) -> ()
            n1020 = Greater?(x=w1566, y=w1564) -> (0:w1556:bool)
            n1021 = Greater?(x=w1565, y=w1564) -> (0:w1555:bool)
            n1022 = In Range and Coerce(upper limit=w1546, x=w1544, lower limit=w1545) -> (In Range?=w1543:bool)  [unwired: 1 out]
            n1023 = Not(x=w1548) -> (.not. x?=w1547:bool)
            n1024 = local read "最大轴向力标准(N)"() -> (w1534:dbl)
            n1025 = property on="总行程" class="DigNum (严格)"("Blinking"=w1547) -> ()  [unwired: 2 in, 2 out]
            n1026 = property on="左全行程间隙" class="DigNum (严格)"("Blinking"=w1556) -> ()  [unwired: 2 in, 2 out]
            n1027 = property on="右全行程间隙" class="DigNum (严格)"("Blinking"=w1555) -> ()  [unwired: 2 in, 2 out]
            n1028 = Not(x=w1543) -> (.not. x?=w1542:bool)
            n1029 = property on="总圈数" class="DigNum (严格)"("Blinking"=w1542) -> ()  [unwired: 2 in, 2 out]
            "轴向力X" <- w1539
            "轴向力Y" <- w1571
          }
          frame #21 {
            n1030 = Greater?(x=w1594, y=w1595) -> (0:w1580:bool)
            n1031 = Greater?(x=w1593, y=w1578) -> (0:w1579:bool)
            n1032 = local read "电动缸快速"() -> (w1574:dbl)
            n1033 = local read "平均轴向力标准(N) max"() -> (w1587:dbl)
            n1034 = property on="右180°内全行程间隙" class="DigNum (严格)"("Blinking"=w1580) -> ()  [unwired: 2 in, 2 out]
            n1035 = property on="右180°外全行程间隙" class="DigNum (严格)"("Blinking"=w1579) -> ()  [unwired: 2 in, 2 out]
            n1036 = local read "轴向力标准(N)"() -> (w1588:dbl)
            n1037 = local read "力波动标准(N)"() -> (w1586:dbl)
            n1038 = local write "电动缸速度(mm/s)"(w1574) -> ()
            n1039 = local read "转向器中心"() -> (w1596:dbl)
            n1040 = call "判断.vi"("y 3"=w1586, "y 2-2"=w1587, "y 2-1"=w1588, "y"=w1575, "x 3"=w1589, "x 2"=w1599, "x"=w1590) -> ("非x? 3"=w1583:bool, "非x? 2"=w1591:bool, "非x?"=w1592:bool)  [unwired: 2 in]
            n1041 = Add(x=w1596, y=-10.0) -> (x+y=w1597:dbl)
          }
          frame #22 {
            n1042 = property on="右最大轴向力(N)" class="DigNum (严格)"("Blinking"=w1610) -> ()  [unwired: 2 in, 2 out]
            n1043 = property on="右平均轴向力(N)" class="DigNum (严格)"("Blinking"=w1609) -> ()  [unwired: 2 in, 2 out]
            n1044 = property on="右轴向力波动(N)" class="DigNum (严格)"("Blinking"=w1608) -> ()  [unwired: 2 in, 2 out]
            n1045 = Compound Arithmetic op=OR(w1607, w1606, w1605, w1604) -> (w1603:bool)
            n1046 = Compound Arithmetic op=OR(w1601, w1603, w1610, w1608, w1612, w1611, w1602) -> (w1614:bool)
            n1047 = Not(x=w1614) -> (.not. x?=w1613:bool)
            n1048 = local write "轴向力及全行程间隙合格"(w1613) -> ()
          }
          frame #23 {
            n1049 = while {
              tunnel: w1631 -> [w1635]
              tunnel: [w1633] -> w1630
              tunnel: w1629 -> [w1632]
              stop <- w1634 stop-if-true
              n1050 = call "PCI1240电动缸位置模式 .vi"("Distance"=w1632, "AxisHandle IN"=w1635) -> ("AbsSuccess"=w1634:bool, "AxisHandle OUT"=w1633:u32)  [unwired: 8 in]
              n1051 = Wait (ms)(milliseconds to wait=u32 50 ("毫秒倍数")) -> ()  [unwired: 1 out]
            }
            n1052 = local read "左拉压力数组"() -> (w1624:dbl[])
            n1053 = local read "右拉压力数组"() -> (w1627:dbl[])
            n1054 = local read "左位移数组"() -> (w1623:dbl[])
            n1055 = local read "右位移数组"() -> (w1626:dbl[])
            n1056 = Multiply(x=-1.0, y=w1627) -> (x*y=w1620:dbl[])
            n1057 = call "压力位移插值.vi"("压力数组"=w1623, "监控点位移"=300.0, "位移数组"=w1624) -> ("监控点压力"=→"监控点压力":dbl)  [unwired: 2 in]
            n1058 = call "压力位移插值.vi"("压力数组"=w1626, "监控点位移"=300.0, "位移数组"=w1620) -> ("监控点压力"=→"监控点压力 2":dbl)  [unwired: 2 in]
          }
          frame #24 {
            n1059 = while {
              tunnel: w1638 -> [w1642]
              stop <- w1640 stop-if-true
              n1060 = call <userlib>:"Acm_AxGetCmdVelocity.vi"("AxisHandle"=w1642) -> ("Velocity"=w1641:dbl)  [unwired: 1 in, 3 out]
              n1061 = Wait Until Next ms Multiple(millisecond multiple=u32 50 ("毫秒倍数")) -> ()  [unwired: 1 out]
              n1062 = Equal To 0?(x=w1641) -> (x = 0?=w1640:bool)
            }
          }
          frame #25 {
            n1063 = while {
              tunnel: w1645 -> [w1649]
              tunnel: [w1647] -> w1644
              tunnel: w1643 -> [w1646]
              stop <- w1648 stop-if-true
              n1064 = call "PCI1240电动缸位置模式 .vi"("Distance"=w1646, "AxisHandle IN"=w1649) -> ("AbsSuccess"=w1648:bool, "AxisHandle OUT"=w1647:u32)  [unwired: 8 in]
              n1065 = Wait (ms)(milliseconds to wait=u32 50 ("毫秒倍数")) -> ()  [unwired: 1 out]
            }
          }
          frame #26 {
            n1066 = while {
              tunnel: w1651 -> [w1655]
              stop <- w1653 stop-if-true
              n1067 = call <userlib>:"Acm_AxGetCmdVelocity.vi"("AxisHandle"=w1655) -> ("Velocity"=w1654:dbl)  [unwired: 1 in, 3 out]
              n1068 = Wait Until Next ms Multiple(millisecond multiple=u32 50 ("毫秒倍数")) -> ()  [unwired: 1 out]
              n1069 = Equal To 0?(x=w1654) -> (x = 0?=w1653:bool)
            }
          }
          frame #27 {
            n1070 = local read "轴向力已做次数"() -> (w1658:dbl)
            n1071 = Add(x=w1658, y=1.0) -> (x+y=w1656:dbl)
            n1072 = local write "轴向力已做次数"(w1656) -> ()
          }
          frame #28 {
            n1073 = local read "轴向力及全行程间隙合格"() -> (w1659:bool)
            n1074 = case shown="假" w1659 {
              frame False {
                n1075 = Less?(x="轴向力已做次数", y="轴向力设定次数") -> (x < y?=w1661:bool)
                n1076 = case shown="假" w1661 {
                  frame False {
                    n1077 = local write "工步号"(u32 45 ("工步号")) -> ()
                  }
                  frame True {
                    n1078 = local write "工步号"(u32 30 ("工步号")) -> ()
                  }
                }
              }
              frame True {
                n1079 = local write "工步号"(u32 45 ("工步号")) -> ()
              }
            }
          }
        }
      }
      frame 45 {
        # "测头退回"
        n1080 = flat-sequence {
          tunnel: [w1669] -> w1666
          tunnel: w1666 -> [w1676]
          frame #0 {
            n1081 = local write "测头机构轴速度(mm/s)"(30.0 ("测头机构轴速度(mm/s)")) -> ()
          }
          frame #1 {
            n1082 = local read "测头机构轴后退位"() -> (w1668:dbl)
            n1083 = local read "测头机构电机"() -> (w1670:u32)
            n1084 = while {
              tunnel: w1670 -> [w1674]
              tunnel: w1668 -> [w1673]
              tunnel: [w1672] -> w1669
              stop <- w1675 stop-if-true
              n1085 = call "PCI1220U进给轴位置模式.vi"("Distance"=w1673, "AxisHandle IN"=w1674) -> ("AbsSuccess"=w1675:bool, "AxisHandle OUT"=w1672:u32)  [unwired: 8 in]
              n1086 = Wait Until Next ms Multiple(millisecond multiple=u32 50 ("毫秒倍数")) -> ()  [unwired: 1 out]
            }
          }
          frame #2 {
            n1087 = while {
              tunnel: w1676 -> [w1680]
              stop <- w1678 stop-if-true
              n1088 = call <userlib>:"Acm_AxGetCmdVelocity.vi"("AxisHandle"=w1680) -> ("Velocity"=w1679:dbl)  [unwired: 1 in, 3 out]
              n1089 = Wait Until Next ms Multiple(millisecond multiple=u32 50 ("毫秒倍数")) -> ()  [unwired: 1 out]
              n1090 = Equal To 0?(x=w1679) -> (x = 0?=w1678:bool)
            }
          }
          frame #3 {
            n1091 = while {
              stop <- w1682 stop-if-true
              n1092 = Wait Until Next ms Multiple(millisecond multiple=u32 50 ("毫秒倍数")) -> ()  [unwired: 1 out]
              n1093 = local read "测头机构轴位置(mm)"() -> (w1684:dbl)
              n1094 = Less Or Equal?(x=w1684, y=35.0) -> (x <= y?=w1682:bool)
            }
          }
          frame #4 {
            n1095 = local write "测头气缸左移"(TRUE ("测头气缸左移")) -> ()
            n1096 = local write "测头气缸右移"(FALSE ("测头气缸右移")) -> ()
          }
          frame #5 {
            n1097 = Wait Until Next ms Multiple(millisecond multiple=u32 500 ("毫秒倍数")) -> ()  [unwired: 1 out]
          }
          frame #6 {
            n1098 = local write "工步号"(u32 50 ("工步号")) -> ()
          }
        }
      }
      frame 50 {
        n1099 = flat-sequence {
          tunnel: [w1711] -> w1700
          tunnel: w1700 -> [w1718]
          tunnel: [w1717] -> w1697
          tunnel: w1697 -> [w1729]
          tunnel: [w1735] -> w1694
          tunnel: w1694 -> [w1738]
          tunnel: [w1737] -> w1693
          tunnel: w1693 -> [w1742]
          tunnel: [w1742] -> w1692
          tunnel: w1692 -> [w1744]
          tunnel: [w1743] -> w1690
          tunnel: [w1750] -> w1691
          tunnel: w1690 -> [w1751]
          tunnel: w1691 -> [w1753]
          tunnel: [w1752] -> w1689
          tunnel: [w1759] -> w1699
          tunnel: w1689 -> [w1759]
          tunnel: w1699 -> [w1762]
          tunnel: [w1761] -> w1698
          tunnel: w1698 -> [w1768]
          tunnel: [w1769] -> w1696
          tunnel: w1696 -> [w1776]
          tunnel: [w1775] -> w1695
          tunnel: w1695 -> [w1786]
          frame #0 {
            n1100 = local write "夹头夹紧"(FALSE ("夹头夹紧")) -> ()
            n1101 = local write "夹头松开"(TRUE ("夹头松开")) -> ()
            n1102 = local write "旋转齿条轴速度(°/s)"(15.0 ("调整螺塞轴速度(°/s)")) -> ()
            n1103 = local write "测头机构轴速度(mm/s)"(15.0 ("调整机构轴速度(mm/s)")) -> ()
            n1104 = local write "电动缸速度(mm/s)"(15.0 ("电动缸速度(mm/s)")) -> ()
          }
          frame #1 {
            n1105 = while {
              stop <- w1706 stop-if-true
              n1106 = Wait Until Next ms Multiple(millisecond multiple=u32 50 ("毫秒倍数")) -> ()  [unwired: 1 out]
              n1107 = local read "夹头夹紧"() -> (w1709:bool)
              n1108 = local read "夹头松开"() -> (w1707:bool)
              n1109 = Not(x=w1709) -> (.not. x?=w1708:bool)
              n1110 = And(x=w1708, y=w1707) -> (x .and. y?=w1706:bool)
            }
          }
          frame #2 {
            n1111 = while {
              tunnel: [w1714] -> w1711
              stop <- w1713 stop-if-true
              n1112 = local read "电动缸电机"() -> (w1715:u32)
              n1113 = local read "齿条右极限"() -> (w1712:dbl)
              n1114 = Wait Until Next ms Multiple(millisecond multiple=u32 50 ("毫秒倍数")) -> ()  [unwired: 1 out]
              n1115 = call "PCI1240电动缸位置模式 .vi"("Distance"=w1712, "AxisHandle IN"=w1715) -> ("AbsSuccess"=w1713:bool, "AxisHandle OUT"=w1714:u32)  [unwired: 8 in]
            }
          }
          frame #3 {
            n1116 = while {
              tunnel: w1718 -> [w1727]
              tunnel: [w1719] -> w1717
              stop <- w1720 stop-if-true
              n1117 = Wait Until Next ms Multiple(millisecond multiple=u32 50 ("毫秒倍数")) -> ()  [unwired: 1 out]
              n1118 = local read "齿条推拉力(N)"() -> (w1725:dbl)
              n1119 = Absolute Value(x=w1725) -> (abs(x)=w1724:dbl)
              n1120 = call <userlib>:"Acm_AxGetCmdVelocity.vi"("AxisHandle"=w1727) -> ("Velocity"=w1728:dbl, "AxisHandle"=w1719:u32)  [unwired: 1 in, 2 out]
              n1121 = Greater Or Equal?(x=w1724, y=1000.0) -> (x >= y?=w1721:bool)
              n1122 = Equal To 0?(x=w1728) -> (x = 0?=w1722:bool)
              n1123 = Or(x=w1722, y=w1721) -> (x .or. y?=w1720:bool)
            }
          }
          frame #4 {
            n1124 = while {
              tunnel: w1729 -> [w1733]
              tunnel: [w1732] -> _
              stop <- w1731 stop-if-true
              n1125 = call "PCI1220U停止.vi"("AxisHandle IN"=w1733) -> ("完成"=w1731:bool, "AxisHandle OUT"=w1732:u32)  [unwired: 9 in]
              n1126 = Wait (ms)(milliseconds to wait=u32 50 ("毫秒倍数")) -> ()  [unwired: 1 out]
            }
          }
          frame #5 {
            n1127 = local write "旋转齿条轴使能"(TRUE ("旋转齿条轴使能")) -> ()
          }
          frame #6 {
            n1128 = local read "旋转齿条电机"() -> (w1735:u32)
            n1129 = Wait Until Next ms Multiple(millisecond multiple=u32 500 ("毫秒倍数")) -> ()  [unwired: 1 out]
          }
          frame #7 {
            n1130 = call <userlib>:"Acm_AxHome.vi"("DirMode"=u32 0, "HomeMode"=u32 11, "AxisHandle"=w1738) -> ("AxisHandle"=w1737:u32)  [unwired: 1 in, 2 out]
          }
          frame #8 {
            n1131 = Wait Until Next ms Multiple(millisecond multiple=u32 100 ("毫秒倍数")) -> ()  [unwired: 1 out]
          }
          frame #9 {
            n1132 = while {
              tunnel: w1744 -> [w1747]
              tunnel: [w1746] -> w1743
              stop <- w1745 stop-if-true
              n1133 = call <userlib>:"Acm_AxGetCmdVelocity.vi"("AxisHandle"=w1747) -> ("Velocity"=w1749:dbl, "AxisHandle"=w1746:u32)  [unwired: 1 in, 2 out]
              n1134 = Wait Until Next ms Multiple(millisecond multiple=u32 50 ("毫秒倍数")) -> ()  [unwired: 1 out]
              n1135 = Equal To 0?(x=w1749) -> (x = 0?=w1745:bool)
            }
          }
          frame #10 {
            n1136 = call "PCI1220U角度置零.vi"("AxisHandle IN"=w1751) -> ("AxisHandle OUT"=w1750:u32)  [unwired: 10 in]
          }
          frame #11 {
            n1137 = while {
              tunnel: w1753 -> [w1755]
              tunnel: [w1754] -> w1752
              stop <- w1758 stop-if-true
              n1138 = Wait Until Next ms Multiple(millisecond multiple=u32 50 ("毫秒倍数")) -> ()  [unwired: 1 out]
              n1139 = call "PCI1220U扭矩轴位置模式.vi"("Distance"=10.0, "AxisHandle IN"=w1755) -> ("AbsSuccess"=w1758:bool, "AxisHandle OUT"=w1754:u32)  [unwired: 8 in]
            }
          }
          frame #12 {
            n1140 = Wait Until Next ms Multiple(millisecond multiple=u32 500 ("毫秒倍数")) -> ()  [unwired: 1 out]
          }
          frame #13 {
            n1141 = while {
              tunnel: w1762 -> [w1765]
              tunnel: [w1764] -> w1761
              stop <- w1763 stop-if-true
              n1142 = call <userlib>:"Acm_AxGetCmdVelocity.vi"("AxisHandle"=w1765) -> ("Velocity"=w1767:dbl, "AxisHandle"=w1764:u32)  [unwired: 1 in, 2 out]
              n1143 = Wait Until Next ms Multiple(millisecond multiple=u32 50 ("毫秒倍数")) -> ()  [unwired: 1 out]
              n1144 = Equal To 0?(x=w1767) -> (x = 0?=w1763:bool)
            }
          }
          frame #14 {
            n1145 = call "PCI1220U角度置零.vi"("AxisHandle IN"=w1768) -> ()  [unwired: 10 in, 1 out]
          }
          frame #15 {
            n1146 = while {
              tunnel: [w1772] -> w1769
              stop <- w1771 stop-if-true
              n1147 = local read "电动缸电机"() -> (w1773:u32)
              n1148 = local read "齿条右极限"() -> (w1770:dbl)
              n1149 = Wait Until Next ms Multiple(millisecond multiple=u32 50 ("毫秒倍数")) -> ()  [unwired: 1 out]
              n1150 = call "PCI1240电动缸位置模式 .vi"("Distance"=w1770, "AxisHandle IN"=w1773) -> ("AbsSuccess"=w1771:bool, "AxisHandle OUT"=w1772:u32)  [unwired: 8 in]
            }
          }
          frame #16 {
            n1151 = while {
              tunnel: w1776 -> [w1784]
              tunnel: [w1782] -> w1775
              stop <- w1777 stop-if-true
              n1152 = Wait Until Next ms Multiple(millisecond multiple=u32 50 ("毫秒倍数")) -> ()  [unwired: 1 out]
              n1153 = local read "齿条推拉力(N)"() -> (w1781:dbl)
              n1154 = call <userlib>:"Acm_AxGetCmdVelocity.vi"("AxisHandle"=w1784) -> ("Velocity"=w1785:dbl, "AxisHandle"=w1782:u32)  [unwired: 1 in, 2 out]
              n1155 = Equal To 0?(x=w1785) -> (x = 0?=w1779:bool)
              n1156 = Greater Or Equal?(x=w1781, y=300.0) -> (x >= y?=w1778:bool)
              n1157 = Or(x=w1779, y=w1778) -> (x .or. y?=w1777:bool)
            }
          }
          frame #17 {
            n1158 = while {
              tunnel: w1786 -> [w1790]
              tunnel: [w1789] -> _
              stop <- w1788 stop-if-true
              n1159 = call "PCI1220U停止.vi"("AxisHandle IN"=w1790) -> ("完成"=w1788:bool, "AxisHandle OUT"=w1789:u32)  [unwired: 9 in]
              n1160 = Wait (ms)(milliseconds to wait=u32 50 ("毫秒倍数")) -> ()  [unwired: 1 out]
            }
          }
          frame #18 {
            n1161 = local write "工步号"(u32 100 ("工步号")) -> ()
          }
        }
      }
      frame 100 {
        n1162 = flat-sequence {
          tunnel: [w1825] -> w1815
          tunnel: [w1823] -> w1814
          tunnel: [w1817] -> w1802
          tunnel: [w1816] -> w1799
          tunnel: w1815 -> [w1832]
          tunnel: w1814 -> [w1829]
          tunnel: ["F:\\报表存储\\" ("字符串")] -> w1813
          tunnel: w1802 -> [w1831]
          tunnel: [w1832] -> w1801
          tunnel: [w1831] -> w1800
          tunnel: w1799 -> [w1830]
          tunnel: [w1830] -> w1798
          tunnel: [w1829] -> w1797
          tunnel: w1813 -> [w1844]
          tunnel: [w1851] -> w1812
          tunnel: [w1849] -> w1811
          tunnel: [w1848] -> w1810
          tunnel: [w1847] -> w1809
          tunnel: w1801 -> [w1843]
          tunnel: w1800 -> [w1842]
          tunnel: w1798 -> [w1841]
          tunnel: w1797 -> [w1834]
          tunnel: [w1836] -> w1792
          tunnel: w1812 -> [w1858]
          tunnel: [w1859] -> w1808
          tunnel: w1811 -> [w1859]
          tunnel: w1810 -> [w1857]
          tunnel: w1809 -> [w1856]
          tunnel: [w1855] -> w1807
          tunnel: [w1854] -> w1806
          tunnel: [w1853] -> w1793
          tunnel: w1792 -> [w1853]
          tunnel: [w1866] -> w1805
          tunnel: w1808 -> [w1866]
          tunnel: w1807 -> [w1865]
          tunnel: [w1865] -> w1804
          tunnel: [w1864] -> w1803
          tunnel: w1806 -> [w1864]
          tunnel: [w1862] -> w1794
          tunnel: w1793 -> [w1862]
          tunnel: w1805 -> [w1869]
          tunnel: w1804 -> [w1877]
          tunnel: w1803 -> [w1876]
          tunnel: [w1868] -> w1795
          tunnel: w1794 -> [w1868]
          tunnel: [w1885] -> w1796
          tunnel: w1795 -> [w1885]
          tunnel: w1796 -> [w1887]
          frame #0 {
            n1163 = local read "产品ID"() -> (w1824:string)
            n1164 = Format Date/Time String(time format string (%c)="%Y%m%d" ("时间格式字符串(%c)")) -> (date/time string=w1818:string)  [unwired: 2 in]
            n1165 = call <vilib>:"Trim Whitespace.vi"("string"=w1824) -> ("trimmed string"=w1823:string)  [unwired: 1 in]
            n1166 = String Subset(string=w1818, offset (0)=0 ("偏移量(0)"), length (rest)=4 ("长度（剩余）")) -> (substring=w1825:string)
            n1167 = String Subset(string=w1818, offset (0)=4 ("偏移量(0)"), length (rest)=2 ("长度（剩余）")) -> (substring=w1817:string)
            n1168 = String Subset(string=w1818, offset (0)=6 ("偏移量(0)"), length (rest)=2 ("长度（剩余）")) -> (substring=w1816:string)
          }
          frame #1 {
          }
          frame #2 {
            w1835 = "\\" ("字符串")
            n1169 = Concatenate Strings(w1844, w1843, w1835, w1842, w1835, w1841, w1835, w1834, w1835) -> (w1852:string)
            n1170 = Concatenate Strings(w1844, w1843, w1835, w1842, w1835, w1841, w1835, w1834, w1835) -> (w1838:string)
            n1171 = Concatenate Strings(w1838, w1834, "间隙曲线.JPG" ("字符串")) -> (w1850:string)
            n1172 = String To Path(string=w1852) -> (path=w1851:path)
            n1173 = String To Path(string=w1850) -> (path=w1849:path)
            n1174 = Concatenate Strings(w1838, w1834, "轴向力曲线.JPG" ("字符串")) -> (w1840:string)
            n1175 = Concatenate Strings(w1838, "扭动曲线数组.txt" ("字符串")) -> (w1848:string)
            n1176 = Concatenate Strings(w1838, "轴向力曲线数组.txt" ("字符串")) -> (w1847:string)
            n1177 = String To Path(string=w1840) -> (path=w1836:path)
          }
          frame #3 {
            n1178 = call <vilib>:"Check if File or Folder Exists.vi"("path"=w1858) -> ("file or folder exists?"=w1860:bool)  [unwired: 8 in, 2 out]
            n1179 = String To Path(string=w1857) -> (path=w1855:path)
            n1180 = String To Path(string=w1856) -> (path=w1854:path)
            n1181 = case shown="假" w1860 {
              tunnel: w1858 -> [w1861 _]
              frame False {
                n1182 = Create Folder(path (use dialog)=w1861) -> ()  [unwired: 2 in, 3 out]
              }
              frame True {
              }
            }
          }
          frame #4 {
            n1183 = Wait Until Next ms Multiple(millisecond multiple=u32 1000 ("毫秒倍数")) -> ()  [unwired: 1 out]
            n1184 = local write "选项卡控件"(T1."间隙测量" ("选项卡控件")) -> ()
          }
          frame #5 {
            n1185 = disable-structure shown="禁用" {
              disable-tunnel: w1869 -> [w1878 _]
              frame Disabled {
                w1882 = T3 2 items=["快速打印", "标准报表", "HTML", "双字节", "Excel"] ("report type (Quick Print)")
                w1881 = T4 1 items=["完整前面板", "前面板可见部分", "图标、说明、前面板和程序框图", "说明信息: 使用前面板", "说明信息: 作为子VI使用", "说明信息: 完整", "说明信息: 自定义"] ("contents (complete front panel)")
                n1186 = Current VI's Path() -> (path=w1880:path)
                n1187 = call-poly <vilib>:"Easy Print VI Panel or Documentation.vi"("report type (Quick Print)"=w1882, "contents (complete front panel)"=w1881, "VI path"=w1880) -> ("error out"=w1884:errorcluster, "report out"=w1883:refnum<class "NI_report.lvclass">)  [unwired: 1 in, 6 out]
                n1188 = call-dynamic "Save Report to File.vi"("report in"=w1883, "report file path"=w1878, "error in (no error)"=w1884) -> ("error out"=→"error out 3":errorcluster)  [unwired: 2 in, 10 out]
              }
              frame Enabled {
              }
            }
            n1189 = control-ref of="本VI"() -> (w1871:refnum<vi>)
            n1190 = invoke class="VI" method="FP.Get Image"(reference=w1871) -> ("image data"=w1870:T5)  [unwired: 5 in, 5 out]
            n1191 = local read "间隙Y数组"() -> (w1874:dbl[])
            n1192 = local read "间隙X数组"() -> (w1875:dbl[])
            n1193 = local read "轴向力Y"() -> (w1872:dbl[])
            n1194 = local read "轴向力X"() -> (w1873:dbl[])
            n1195 = call <vilib>:"Write JPEG File.vi"("image data"=w1870, "path to JPEG file"=w1869) -> ()  [unwired: 8 in, 2 out]
            n1196 = call "导出曲线数组.vi"("file path (dialog if empty)"=w1877, "数组 2"=w1874, "数组"=w1875) -> ()  [unwired: 9 in]
            n1197 = call "导出曲线数组.vi"("file path (dialog if empty)"=w1876, "数组 2"=w1872, "数组"=w1873) -> ()  [unwired: 9 in]
          }
          frame #6 {
            n1198 = local write "选项卡控件"(T1."轴向力测量" ("选项卡控件")) -> ()
          }
          frame #7 {
            n1199 = control-ref of="本VI"() -> (w1888:refnum<vi>)
            n1200 = invoke class="VI" method="FP.Get Image"(reference=w1888) -> ("image data"=w1889:T5)  [unwired: 5 in, 5 out]
            n1201 = call <vilib>:"Write JPEG File.vi"("image data"=w1889, "path to JPEG file"=w1887) -> ()  [unwired: 8 in, 2 out]
          }
          frame #8 {
            n1202 = local read "联线按钮"() -> (w1890:bool)
            n1203 = case shown="真" w1890 {
              frame False {
              }
              frame True {
                n1204 = flat-sequence {
                  tunnel: [w1893] -> w1891
                  tunnel: [w1921] -> w1892
                  tunnel: w1891 -> [w1917]
                  tunnel: w1892 -> [w1933]
                  frame #0 {
                    n1205 = local read "轴向力及全行程间隙合格"() -> (w1894:bool)
                    n1206 = local read "单点间隙合格"() -> (w1895:bool)
                    n1207 = And(x=w1895, y=w1894) -> (x .and. y?=w1893:bool)
                  }
                  frame #1 {
                    w1915 = i16 3 ("精度(6)")
                    n1208 = local read "左180°内全行程间隙"() -> (w1924:dbl)
                    n1209 = local read "右180°内全行程间隙"() -> (w1914:dbl)
                    n1210 = local read "左180°外全行程间隙"() -> (w1906:dbl)
                    n1211 = local read "右180°外全行程间隙"() -> (w1907:dbl)
                    n1212 = local read "左最大轴向力(N)"() -> (w1908:dbl)
                    n1213 = local read "右最大轴向力(N)"() -> (w1909:dbl)
                    n1214 = local read "左轴向力波动(N)"() -> (w1910:dbl)
                    n1215 = local read "右轴向力波动(N)"() -> (w1911:dbl)
                    n1216 = local read "中间位置间隙"() -> (w1926:dbl)
                    n1217 = local read "总行程"() -> (w1912:dbl)
                    n1218 = local read "总圈数"() -> (w1913:dbl)
                    n1219 = Boolean To (0,1)(Boolean=w1917) -> (0, 1=w1919:i16)
                    n1220 = local read "员工ID"() -> (w1896:string)
                    n1221 = local read "产品ID"() -> (w1931:string)
                    n1222 = Format Date/Time String(time format string (%c)="%Y%m%d%H%M" ("时间格式字符串(%c)")) -> (date/time string=w1929:string)  [unwired: 2 in]
                    n1223 = Number To Fractional String(number=w1924, precision (6)=w1915) -> (F-format string=w1922:string)  [unwired: 2 in]
                    n1224 = Number To Fractional String(number=w1914, precision (6)=w1915) -> (F-format string=w1905:string)  [unwired: 2 in]
                    n1225 = Number To Fractional String(number=w1906, precision (6)=w1915) -> (F-format string=w1904:string)  [unwired: 2 in]
                    n1226 = Number To Fractional String(number=w1907, precision (6)=w1915) -> (F-format string=w1903:string)  [unwired: 2 in]
                    n1227 = Number To Fractional String(number=w1908, precision (6)=w1915) -> (F-format string=w1902:string)  [unwired: 2 in]
                    n1228 = Number To Fractional String(number=w1909, precision (6)=w1915) -> (F-format string=w1901:string)  [unwired: 2 in]
                    n1229 = Number To Fractional String(number=w1910, precision (6)=w1915) -> (F-format string=w1900:string)  [unwired: 2 in]
                    n1230 = Number To Fractional String(number=w1911, precision (6)=w1915) -> (F-format string=w1899:string)  [unwired: 2 in]
                    n1231 = Number To Fractional String(number=w1912, precision (6)=w1915) -> (F-format string=w1898:string)  [unwired: 2 in]
                    n1232 = Number To Fractional String(number=w1913, precision (6)=w1915) -> (F-format string=w1897:string)  [unwired: 2 in]
                    n1233 = Number To Decimal String(number=w1919, width (-)=i16 1 ("宽度(-)")) -> (decimal integer string=w1916:string)
                    n1234 = Number To Fractional String(number=w1926, precision (6)=i16 3 ("精度(6)")) -> (F-format string=w1923:string)  [unwired: 2 in]
                    n1235 = local read "KSJJ"() -> (w1930:string)
                    n1236 = local read "FGCS"() -> (w1928:string)
                    n1237 = Build Array(w1931, w1896, "1", w1916, w1930, w1929, w1928, "Q14073-11A", w1923, w1922, w1905, w1904, w1903, w1902, w1901, w1900, w1899, w1898, w1897) -> (w1921:string[])
                  }
                  frame #2 {
                    n1238 = Wait (ms)(milliseconds to wait=u32 500 ("等待时间（毫秒）")) -> ()  [unwired: 1 out]
                    n1239 = call "数据库更新.vi"("设备号"="06", "数据"=w1933) -> ()  [unwired: 13 in, 1 out]
                  }
                  frame #3 {
                  }
                }
              }
            }
          }
          frame #9 {
            n1240 = local write "工步号"(u32 0 ("工步号")) -> ()
            n1241 = local write "产品ID"("") -> ()
          }
        }
      }
    }
    n1242 = local read "停止"() -> (w612:bool)
  }
  n1243 = while {
    stop <- w1939 stop-if-true
    n1244 = local read "rfid工步号"() -> (w1938:u32)
    n1245 = Wait Until Next ms Multiple(millisecond multiple=u32 50 ("毫秒倍数")) -> ()  [unwired: 1 out]
    n1246 = case shown="10" w1938 {
      frame 0, Default {
      }
      frame 10 {
        n1247 = flat-sequence {
          tunnel: [w1949] -> w1943
          tunnel: w1943 -> [w1951]
          tunnel: [w1950] -> w1942
          tunnel: w1942 -> [w1953]
          tunnel: [w1953] -> w1941
          tunnel: w1941 -> [w1956]
          frame #0 {
            n1248 = while {
              stop <- w1944 stop-if-true
              n1249 = local read "rfid触发"() -> (w1944:bool)
              n1250 = Wait Until Next ms Multiple(millisecond multiple=u32 50 ("毫秒倍数")) -> ()  [unwired: 1 out]
            }
          }
          frame #1 {
            n1251 = local write "rfid完成"(FALSE ("RFID完成")) -> ()
            n1252 = local write "rfid触发"(FALSE ("RFID读取触发")) -> ()
            n1253 = local write "芯片ID"("" ("随行板ID")) -> ()
          }
          frame #2 {
            n1254 = local read "Z060BRFID"() -> (w1949:string)
            n1255 = local write "芯片ID"(w1949) -> ()
          }
          frame #3 {
            n1256 = call "查询产品ID.vi"("芯片编码"=w1951) -> ("产品ID"=w1950:string)  [unwired: 8 in, 2 out]
            "读取产品ID" <- w1950
          }
          frame #4 {
            n1257 = Wait (ms)(milliseconds to wait=u32 500 ("等待时间（毫秒）")) -> ()  [unwired: 1 out]
          }
          frame #5 {
            n1258 = call "查询上序合格.vi"("产品ID"=w1956) -> ("本序已做"=w1954:bool, "上序合格"=w1955:bool)  [unwired: 8 in, 1 out]
            n1259 = Not(x=w1955) -> (.not. x?=w1957:bool)
            n1260 = local write "上序合格"(w1955) -> ()
            n1261 = local write "本序已做"(w1954) -> ()
            n1262 = local write "上序不合格"(w1957) -> ()
          }
          frame #6 {
            n1263 = local write "rfid完成"(TRUE ("RFID读取完成")) -> ()
            n1264 = Wait Until Next ms Multiple(millisecond multiple=u32 500 ("毫秒倍数")) -> ()  [unwired: 1 out]
          }
          frame #7 {
            "rfid工步号" <- 15.0 ("工步号")
          }
        }
      }
      frame 210 {
        n1265 = local read "读取产品ID"() -> (w1961:string)
        n1266 = local write "产品ID"(w1961) -> ()
      }
    }
    n1267 = local read "停止"() -> (w1939:bool)
  }
